vi "Text control 2 v7.3.vi"() -> ()   [LabVIEW 2019]
panel:
  in  "Tab Control":enum32{"Main", "Other parameters"}(tab)
  out "Vdg vs time (Bias Stress)":cluster{"Y data in":dbl[], "X data in":dbl[]}[](graph)
  out "Vp vs Vg (FPP)":cluster{"Y data in":dbl[], "X data in":dbl[]}[](graph)
  out "Vp2":dbl format="%.2e"
  out "Vp1":dbl format="%.2e"
  out "Vp vs time (FPP Bias Stress)":cluster{"Y data in":dbl[], "X data in":dbl[]}[](graph)
  in  "Plot sample extrema vs time":bool
  out "Line running":i32
  out "Total lines":i32
  out "Path":path=path "C:/users/rlp38/09Apr2009LTtesting/test2.txt"
  out "I vs Vg":cluster{"Y data in":dbl[], "X data in":dbl[]}[](graph)
  out "Is max":dbl format="%.2e"
  out "Id max":dbl format="%.2e"
  out "Ig max":dbl format="%.2e"
  out "Imax vs time":cluster{"Y data in":dbl[], "X data in":dbl[]}[](graph)
  out "Imin vs time":cluster{"Y data in":dbl[], "X data in":dbl[]}[](graph)
  out "I vs Vd":cluster{"Y data in":dbl[], "X data in":dbl[]}[](graph)
  in  "Script":string="#pulsedstressV d 0.03 20 0 0.5 0.0827 5\n#\n#itime m\n#gaterangemode a\n#drainrangemode a\n#pulsed on 0.05 0 0.02\n#transfer d -10 40 1 5 40 35\n#transfer d -10 40 1 5 40 35\n#transfer d -10 40 1 5 40 35\n#output d 0 40 20 0 40 1\n#\n#\n#sample 1 0.008 221 6 0.003\n#samplei 400e-6 200 6 0.002 0.1\n#vsu2pulse -10 4\n#\n#stressV 0.016 0.03 2e-4 0.1e-3 11\n#stressI 220e-7 0.08 15\n#transfer s -1 1 0.5 -0.005 0.005 0.005\n#output s 0 0 0 -0.008 0.008 0.002"
  out "Command running:":string
  out "Serial port data":string
  out "Elapsed Time":dbl caption="Elapsed Time (s)"
  in  "Time Units":u16(ring)=1 items=["Seconds", "Minutes", "Hours"]
  in  "Time Offset":dbl caption="Set Start Time (s)"
  in  "Reset":bool
  in  "Auto Reset":bool
  in  "integration time":u32(slide) max=2 step=1 scale=0.0..2.0
  out "Is on":dbl format="%.2e"
  out "Id on":dbl format="%.2e"
  out "Ig on":dbl format="%.2e"
  out "Ion vs time":cluster{"Y data in":dbl[], "X data in":dbl[]}[](graph)
  out "Ioff vs time":cluster{"Y data in":dbl[], "X data in":dbl[]}[](graph)
  out "Ig min":dbl format="%.2e"
  out "Id min":dbl format="%.2e"
  out "Is min":dbl format="%.2e"
  out "Is off":dbl format="%.2e"
  out "Id off":dbl format="%.2e"
  out "Ig off":dbl format="%.2e"
  in  "Integration time (long)":dbl=0.32 min=0.04 max=2.0 step=0.02 format="%.2f"
  in  "Integration time (short)":dbl=0.0019 min=8e-05 max=0.0019 step=8e-05 format="%^.0e"
  in  "Drain: Compliance":dbl=0.001 format="%.8f"
  in  "Gate: Compliance":dbl=0.001 format="%.8f"
  in  "Interrupt scan":bool
  in  "Interrupt program":bool
  in  "Plot output curve extrema vs time":bool
  in  "Plot transfer curve extrema vs time":bool
  out "I vs time (Bias Stress)":cluster{"Y data in":dbl[], "X data in":dbl[]}[](graph)
  in  "Sample I - Probe 4 (Disabled)":u32(ring)=3 items=["SMU1  ", "SMU2  ", "SMU3  ", "SMU4  ", "SMU5  ", "SMU6  ", "VSU1  ", "VSU2  "]
  in  "Sample I - Source/Common":u32(ring) items=["SMU1  ", "SMU2  ", "SMU3  ", "SMU4  ", "SMU5  ", "SMU6  ", "VSU1  ", "VSU2  "]
  in  "Sample I - Probe 3 (Disabled)":u32(ring)=2 items=["SMU1  ", "SMU2  ", "SMU3  ", "SMU4  ", "SMU5  ", "SMU6  ", "VSU1  ", "VSU2  "]
  in  "Sample I - Drain/Gate":u32(ring)=1 items=["SMU1  ", "SMU2  ", "SMU3  ", "SMU4  ", "SMU5  ", "SMU6  ", "VSU1  ", "VSU2  "]
  in  "Sample - Probe 4":u32(ring)=3 items=["SMU1  ", "SMU2  ", "SMU3  ", "SMU4  ", "SMU5  ", "SMU6  ", "VSU1  ", "VSU2  "]
  in  "Sample - Source/Common":u32(ring) items=["SMU1  ", "SMU2  ", "SMU3  ", "SMU4  ", "SMU5  ", "SMU6  ", "VSU1  ", "VSU2  "]
  in  "Sample - Gate":u32(ring)=2 items=["SMU1  ", "SMU2  ", "SMU3  ", "SMU4  ", "SMU5  ", "SMU6  ", "VSU1  ", "VSU2  "]
  in  "Sample - Drain":u32(ring)=1 items=["SMU1  ", "SMU2  ", "SMU3  ", "SMU4  ", "SMU5  ", "SMU6  ", "VSU1  ", "VSU2  "]
  in  "Gate Range\nmode":u16(ring) items=["Auto", "Limited", "Fixed"]
  in  "Gate Range":u8(slide)=3 max=11 scale=0.0..11.0
  in  "Source/Drain\nRange mode":u16(ring) items=["Auto", "Limited", "Fixed"]
  in  "Source/Drain Range":u8(slide)=3 max=11 scale=0.0..11.0
  in  "Panel Controls":T1={"Emergency Stop"=refnum, "TransGraph Max"=1e-05, "Text/Graph (text=false)"=TRUE} {"TransGraph Max" format="%.2e"}
  in  "Panel Controls 2":T2={"Emergency Stop"=refnum, "TransGraph Max"=1e-05, "Text/Graph (text=false)"=TRUE, "TransGraph Min"=1e-11} {"TransGraph Min" format="%.2e"; "TransGraph Max" format="%.2e"}
  out "error out":errorcluster
  in  "Delay before read (ms)":u32=1000
  in  "byte count":u32=64
  in  "Serial End Mode for Reads":u16(ring)=2 items=["None", "LastBit", "TermChar"]
  in  "Timeout (ms)":u32=10000
  in  "Enable Termination\nChar (T)":bool=TRUE
  in  "Termination char\n(0xA = '\\n' = LF)\n(0xD = '\\r' = CR)":u8=13 format="%.0x"
  in  "flow control":u16(ring) items=["None"=0, "XON/XOFF"=1, "RTS/CTS"=2, "DTR/DSR"=4]
  in  "stop bits":u16(ring)=10 items=["1.0"=10, "1.5"=15, "2.0"=20]
  in  "parity":u16(ring) items=["None", "Odd", "Even", "Mark", "Space"]
  in  "data bits":u16=8 min=5 max=8 step=1
  in  "VISA resource name":refnum<visa-resource-name>="COM6"
  in  "baud rate":u32=9600
  out "Timings Indicator":T3
  in  "Timings (overwritten by the Front Panel)":T4={"integration time"=0, "Short/Long integration time"=0.00064, "hold time (sec)"=0.0, "delay time (sec)"=0.0, "Step Time (0 disables)"=0.0, "sweep method"=0, "Pulse period"=0.005, "Base voltage"=0.0, "Pulse width"=0.0005} {"Pulse width" min=0.0005 max=0.1 step=0.0001 format="%.4f"; "Base voltage" format="%^.4e"; "Pulse period" min=0.005 max=1.0 step=0.0001 format="%.4f"; "sweep method" items=["Continuous", "Pulsed"]; "Step Time (0 disables)" format="%.2f"; "delay time (sec)" format="%.4f"; "hold time (sec)" format="%.4f"; "Short/Long integration time" format="%^.0e"; "integration time" scale=0.0..2.0}
  in  "Probe 4":cluster{"on/off":bool, "Voltage":dbl} {"Voltage" min=-100.0 max=100.0 format="%.2f"}
  in  "Full Reset":bool
  in  "Standby":T5
  out "Probe 4 Indicator":cluster{"on/off":bool, "Voltage":dbl} {"Voltage" min=-100.0 max=100.0 format="%.2f"}
  in  "Transfer/Output - Drain":u32(ring)=1 items=["SMU1  ", "SMU2  ", "SMU3  ", "SMU4  ", "SMU5  ", "SMU6  ", "VSU1  ", "VSU2  "]
  in  "Transfer/Output - Gate":u32(ring)=2 items=["SMU1  ", "SMU2  ", "SMU3  ", "SMU4  ", "SMU5  ", "SMU6  ", "VSU1  ", "VSU2  "]
  in  "Transfer/Output - Source/Common":u32(ring) items=["SMU1  ", "SMU2  ", "SMU3  ", "SMU4  ", "SMU5  ", "SMU6  ", "VSU1  ", "VSU2  "]
  in  "Transfer/Output - Probe 4":u32(ring)=3 items=["SMU1  ", "SMU2  ", "SMU3  ", "SMU4  ", "SMU5  ", "SMU6  ", "VSU1  ", "VSU2  "]
  in  "Pulsed Stress V - Probe 4":u32(ring)=3 items=["SMU1  ", "SMU2  ", "SMU3  ", "SMU4  ", "SMU5  ", "SMU6  ", "VSU1  ", "VSU2  "]
  in  "Pulsed Stress V - Vextra":u32(ring)=6 items=["SMU1  ", "SMU2  ", "SMU3  ", "SMU4  ", "SMU5  ", "SMU6  ", "VSU1  ", "VSU2  "]
  in  "Pulsed Stress V - Drain":u32(ring)=1 items=["SMU1  ", "SMU2  ", "SMU3  ", "SMU4  ", "SMU5  ", "SMU6  ", "VSU1  ", "VSU2  "]
  in  "Pulsed Stress V - Source/Common":u32(ring) items=["SMU1  ", "SMU2  ", "SMU3  ", "SMU4  ", "SMU5  ", "SMU6  ", "VSU1  ", "VSU2  "]
  in  "Pulsed Stress V - Gate":u32(ring)=2 items=["SMU1  ", "SMU2  ", "SMU3  ", "SMU4  ", "SMU5  ", "SMU6  ", "VSU1  ", "VSU2  "]
  in  "FPP - Drain":u32(ring)=1 items=["SMU1  ", "SMU2  ", "SMU3  ", "SMU4  ", "SMU5  ", "SMU6  ", "VSU1  ", "VSU2  "]
  in  "FPP - Gate":u32(ring)=2 items=["SMU1  ", "SMU2  ", "SMU3  ", "SMU4  ", "SMU5  ", "SMU6  ", "VSU1  ", "VSU2  "]
  in  "FPP - Probe 1":u32(ring) items=["SMU1  ", "SMU2  ", "SMU3  ", "SMU4  ", "SMU5  ", "SMU6  ", "VSU1  ", "VSU2  "]
  in  "FPP - Probe 2":u32(ring)=3 items=["SMU1  ", "SMU2  ", "SMU3  ", "SMU4  ", "SMU5  ", "SMU6  ", "VSU1  ", "VSU2  "]
  in  "FPP - Source":u32(ring)=6 items=["SMU1  ", "SMU2  ", "SMU3  ", "SMU4  ", "SMU5  ", "SMU6  ", "VSU1  ", "VSU2  "]
  in  "Stress V - Drain":u32(ring)=1 items=["SMU1  ", "SMU2  ", "SMU3  ", "SMU4  ", "SMU5  ", "SMU6  ", "VSU1  ", "VSU2  "]
  in  "Stress V - Gate":u32(ring)=2 items=["SMU1  ", "SMU2  ", "SMU3  ", "SMU4  ", "SMU5  ", "SMU6  ", "VSU1  ", "VSU2  "]
  in  "Stress V - Source/Common":u32(ring) items=["SMU1  ", "SMU2  ", "SMU3  ", "SMU4  ", "SMU5  ", "SMU6  ", "VSU1  ", "VSU2  "]
  in  "Stress I - Drain/Gate":u32(ring)=1 items=["SMU1  ", "SMU2  ", "SMU3  ", "SMU4  ", "SMU5  ", "SMU6  ", "VSU1  ", "VSU2  "]
  in  "Stress I - Source/Common":u32(ring) items=["SMU1  ", "SMU2  ", "SMU3  ", "SMU4  ", "SMU5  ", "SMU6  ", "VSU1  ", "VSU2  "]
  in  "VSU2 Stress - Source/Common":u32(ring) items=["SMU1  ", "SMU2  ", "SMU3  ", "SMU4  ", "SMU5  ", "SMU6  ", "VSU1  "]
  in  "VISA resource name in":refnum<visa-resource-name>="GPIB0::14::INSTR"
  in  "Gate":T6={"Gate Start"=0.0, "Gate Stop"=2.0, "Gate Step (linear only)"=1.0, "Gate Compliance"=0.0001, "Gate PComp"=0.0, "Range mode"=0, "Range"=6} {"Range" max=11 scale=0.0..11.0; "Range mode" items=["Auto", "Limited", "Fixed"]; "Gate PComp" format="%^.2e"; "Gate Compliance" format="%^.2e"; "Gate Step (linear only)" format="%^.4e"; "Gate Stop" format="%^.4e"; "Gate Start" format="%^.4e"}
  in  "Drain 2":T7={"Drain Start"=0.0, "Drain Stop"=2.0, "Drain Compliance"=0.0001, "Drain Step"=1.0, "Drain PComp"=0.0, "Range mode"=0, "Range"=6} {"Range" max=11 scale=0.0..11.0; "Range mode" items=["Auto", "Limited", "Fixed"]; "Drain PComp" format="%^.2e"; "Drain Step" format="%^.4e"; "Drain Compliance" format="%^.2e"; "Drain Stop" format="%^.4e"; "Drain Start" format="%^.4e"}
  # "Time"
  # "Syntax:\nitime [s|m|l] time(sec): [s|m|l] determines the integration time setting (small|medium|long) and time sets the value.\nNOTE: The value of the integration time has to be within the range allowed by its category (s|m|l), otherwise, the closest value will be used. (e.g. if the category is set to short but the time value is very long, the actual value used will be the maximum short integration time.\nIntegration times:\n    Short: Default: 640 us. Range: 8E-5 - 1.92E-3 seconds.\n    Medium: Fixed at 1 NPL cycle (0.02 seconds).\n    Long: Default: 16 NPL cycles (0.32 seconds). Range: 2-100 NPL cycles (0.04 seconds - 2 seconds).\ngaterangemode [a|l|f]\ndrainrangemode [a|l|f]\npulsed [on|off] PulsePeriod(sec) PulseBaseVoltage PulseONWidth(sec)\nstandby [on l off]\nwait NumMilliseconds\nwait-min NumMinutes\n# texthere = comment\nProbe4 [ON|OFF] Voltage\ntransfer [s|d] VgStart VgStop VgStep VdStart VdStop VdStep\noutput [s|d] VgStart VgStop VgStep VdStart VdStop VdStep\nsample Vg Vd NumSamples Time(s) SampleInterval(s)\nsamplei Idg NumSamples Time(s) SampleInterval(s) VDGcompliance\n100 samples is approximately 13 seconds with medium integration\n# if in doubt use SampleInterval(s) = 0.004\n    NOTE: When doing bias stress measurements, it is best to set the Time Units to \"Seconds\", as the \"sample\" command has been configured to give the output to seconds.\nstressV VG VD IGcompliance IDcompliance Duration(sec)\nstressI IDG VDGcompliance Duration(sec)\nvsu2pulse Bias Duration(s)\npulsedstressV [s|d] VEstop VgON VgOFF Period(s) PulseONwidth(s) Vd\nsample-fpp Vg Vd NumSamples Time\nresample-fpp Vg Vd\ntransfer-fpp [s|d] VgStart VgStop VgStep VdStart VdStop VdStep\noutput-fpp [s|d] VgStart VgStop VgStep VdStart VdStop VdStep\nserial SerialPortCommand"
  # "1\n2\n3\n4\n5\n6\n7\n8\n9\n10\n11\n12\n13\n14\n15\n16\n17\n18\n19\n20"
  # "SMUs"
  # "Serial port settings"
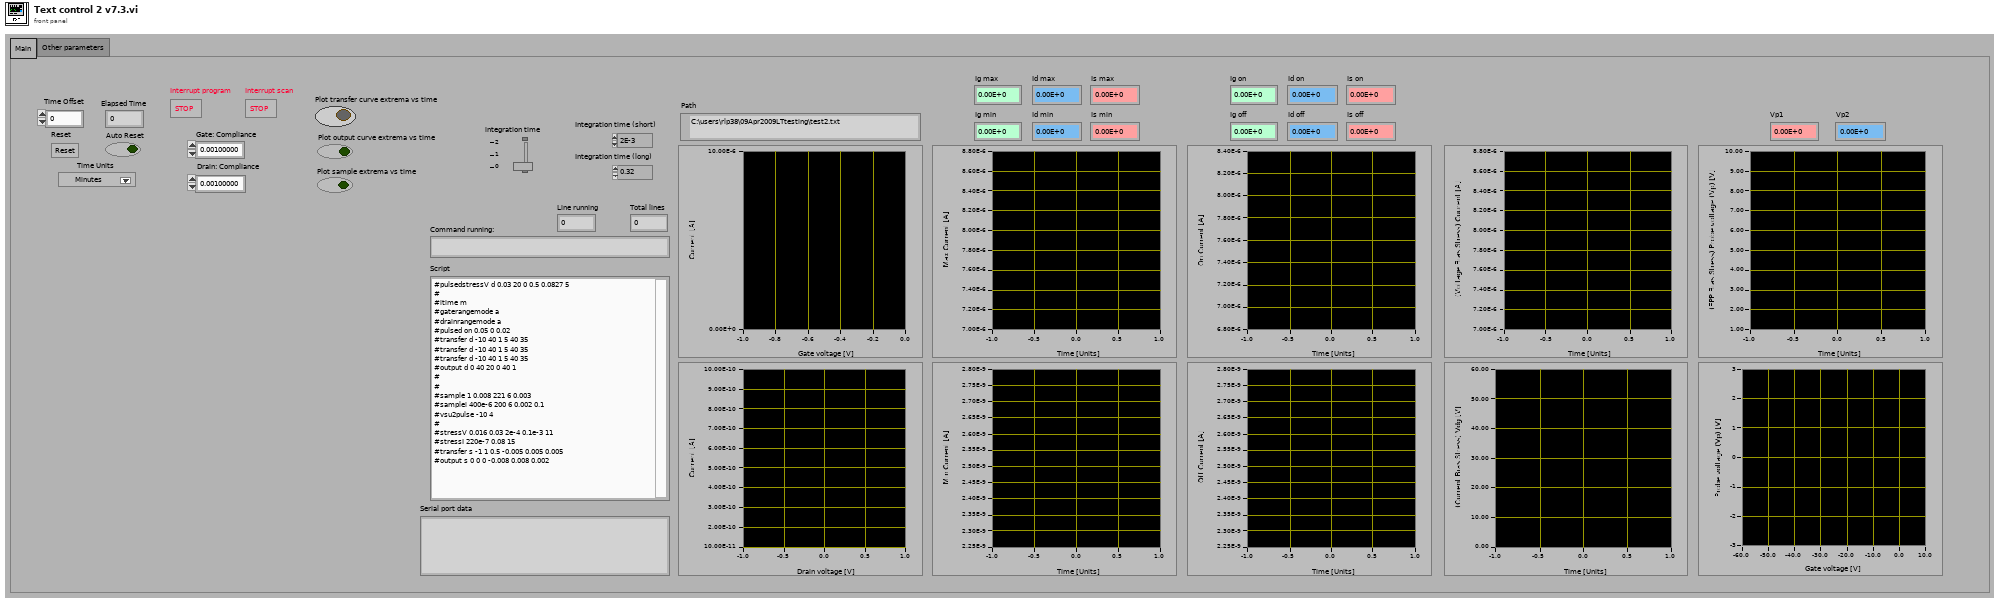
[diagram p1: front panel]
types:
  T1 = cluster{"Emergency Stop":refnum<vi>, "TransGraph Max":dbl, "Text/Graph (text=false)":bool}
  T2 = cluster{"Emergency Stop":refnum<vi>, "TransGraph Max":dbl, "Text/Graph (text=false)":bool, "TransGraph Min":dbl}
  T3 = cluster{"integration time (0:s, 1:m, 2:l)":u32, "Short/Long integration time":dbl, "hold time (sec)":dbl, "delay time (sec)":dbl, "Step Time (0 disables)":dbl, "sweep method":u16, "Pulse period":dbl, "Base voltage":dbl, "Pulse width":dbl}
  T4 = cluster{"integration time":u32, "Short/Long integration time":dbl, "hold time (sec)":dbl, "delay time (sec)":dbl, "Step Time (0 disables)":dbl, "sweep method":u16, "Pulse period":dbl, "Base voltage":dbl, "Pulse width":dbl}
  T5 = cluster{"Gate Standby":bool, "Drain Standby":bool}
  T6 = cluster{"Gate Start":dbl, "Gate Stop":dbl, "Gate Step (linear only)":dbl, "Gate Compliance":dbl, "Gate PComp":dbl, "Range mode":u16, "Range":u8}
  T7 = cluster{"Drain Start":dbl, "Drain Stop":dbl, "Drain Compliance":dbl, "Drain Step":dbl, "Drain PComp":dbl, "Range mode":u16, "Range":u8}
  T8 = enum16{"open", "replace", "create", "open or create", "replace or create", "replace or create with confirmation"}
  T9 = cluster{"V2 Start":dbl, "V2 Step":dbl, "Number of points":i32}
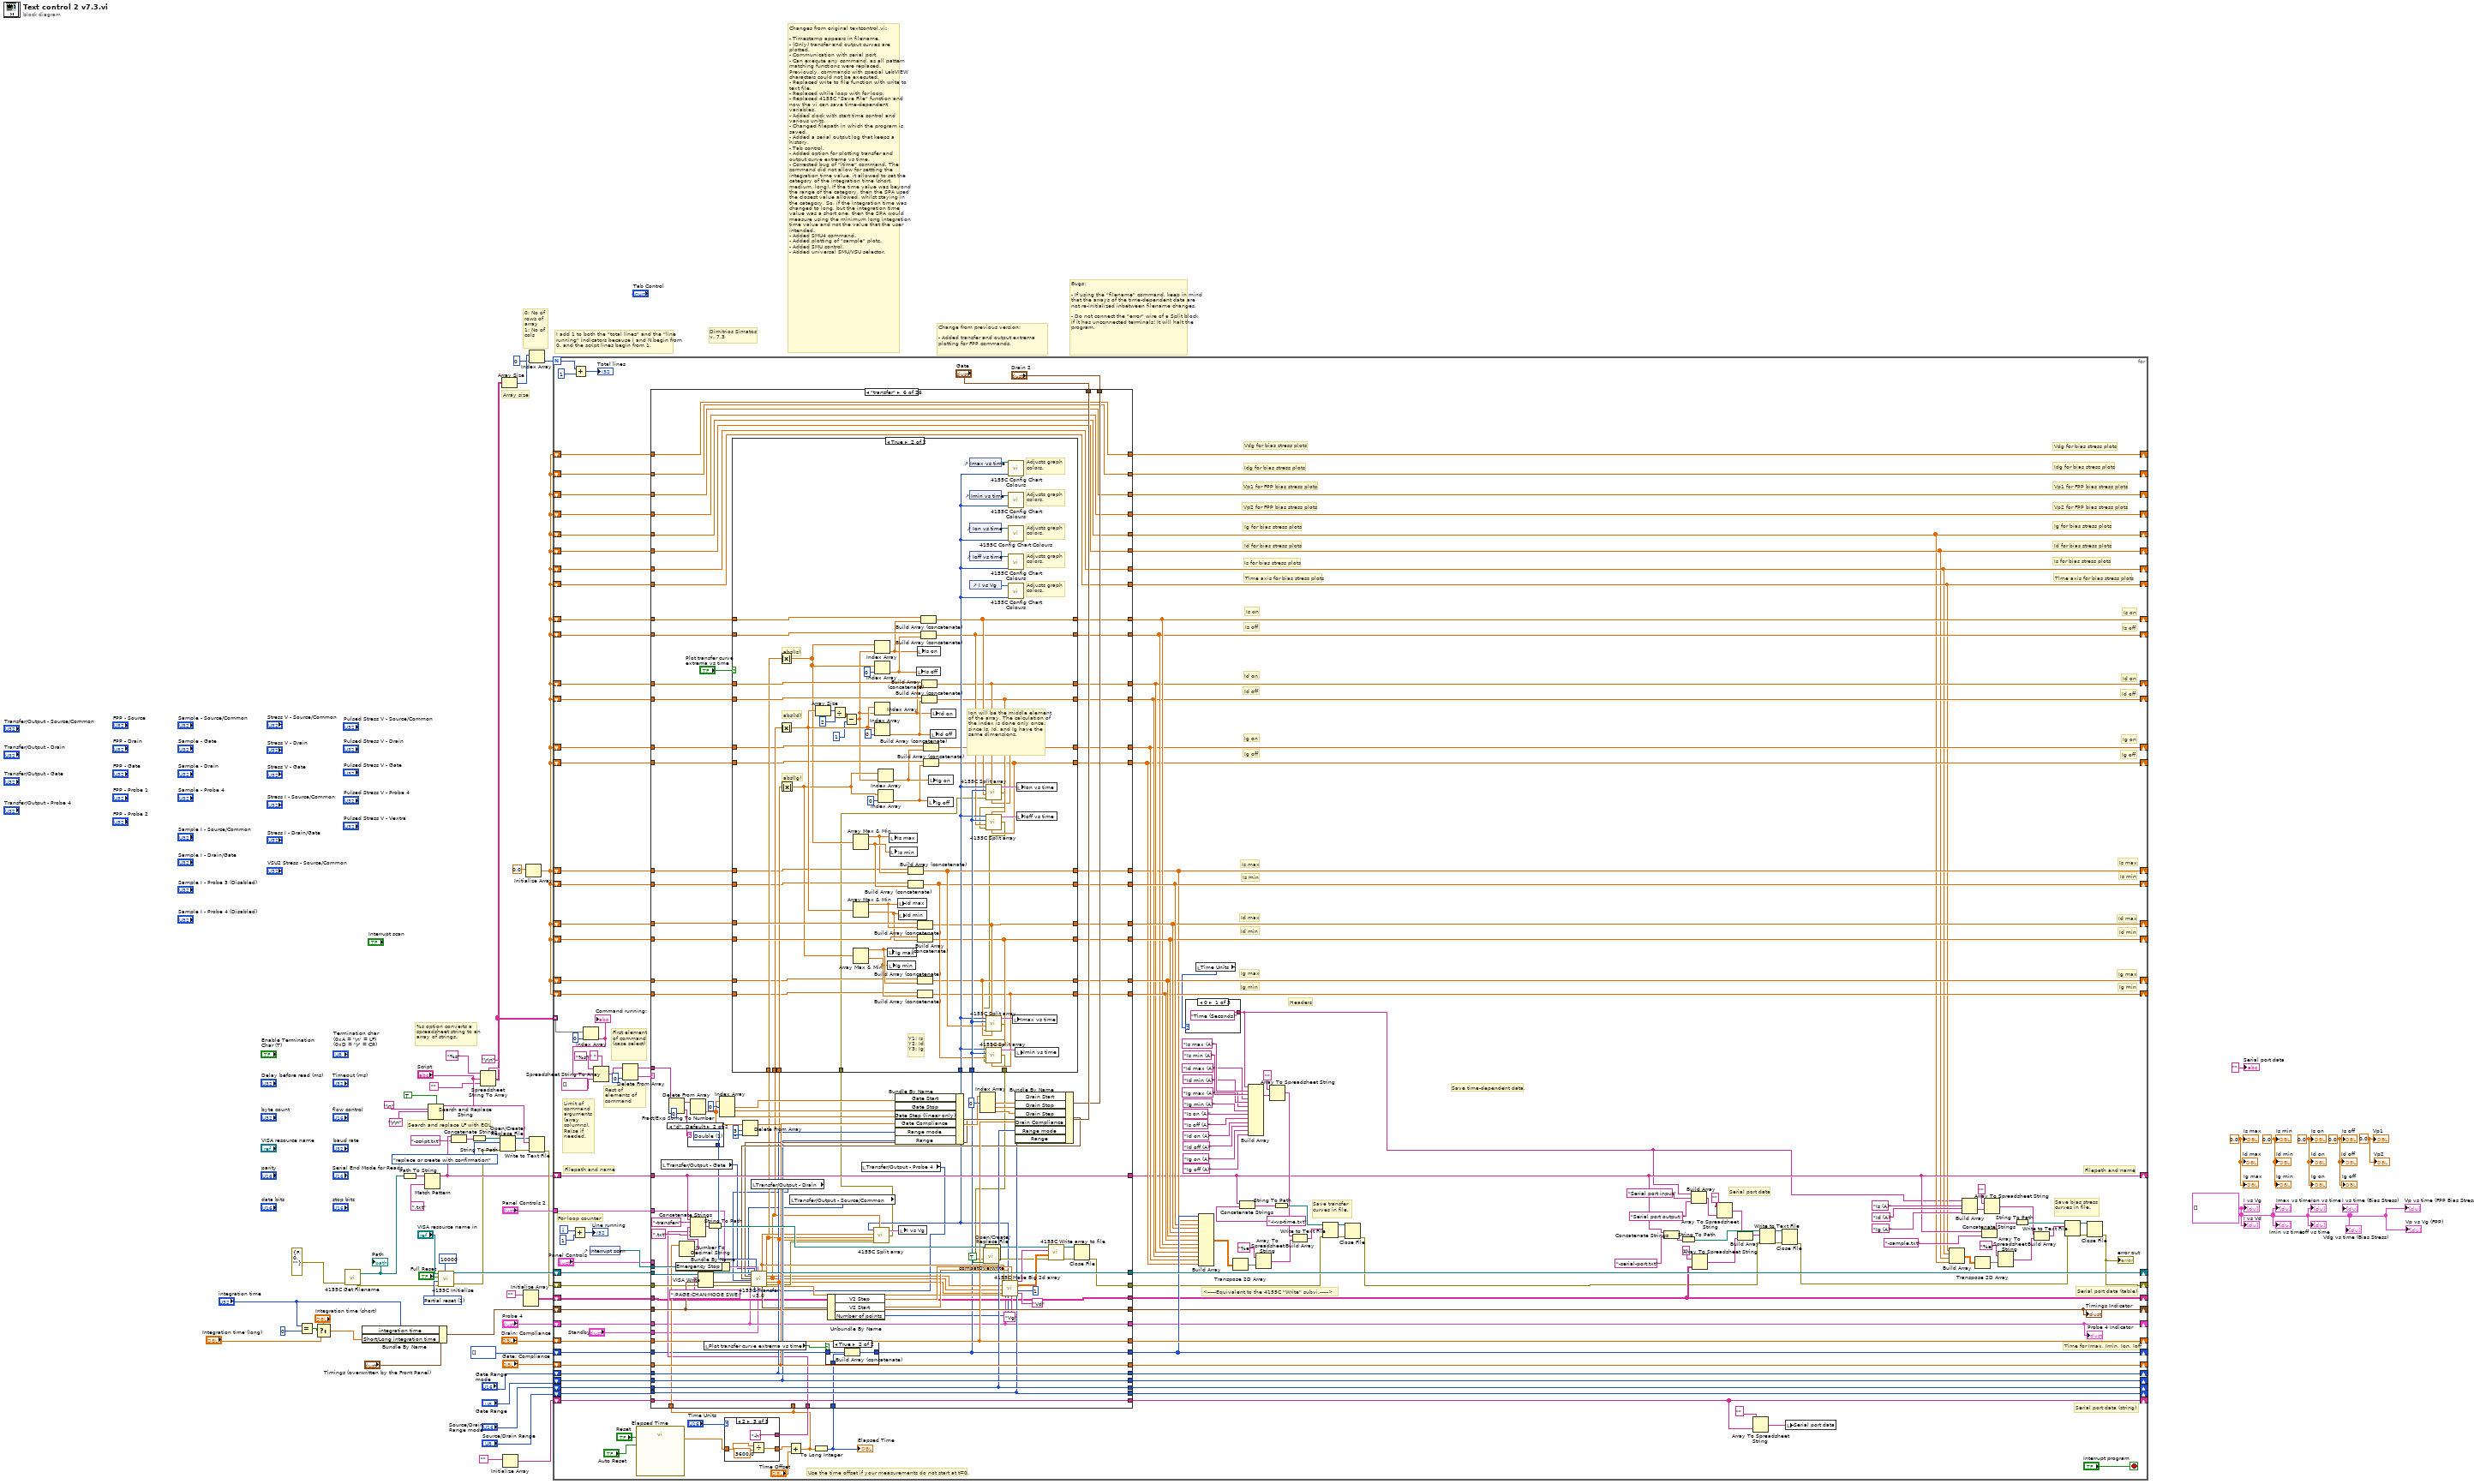
[diagram p0: block diagram]
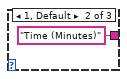
[diagram p2: hidden frame]
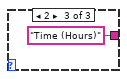
[diagram p3: hidden frame]
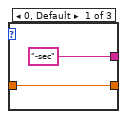
[diagram p4: hidden frame]
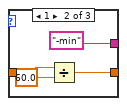
[diagram p5: hidden frame]
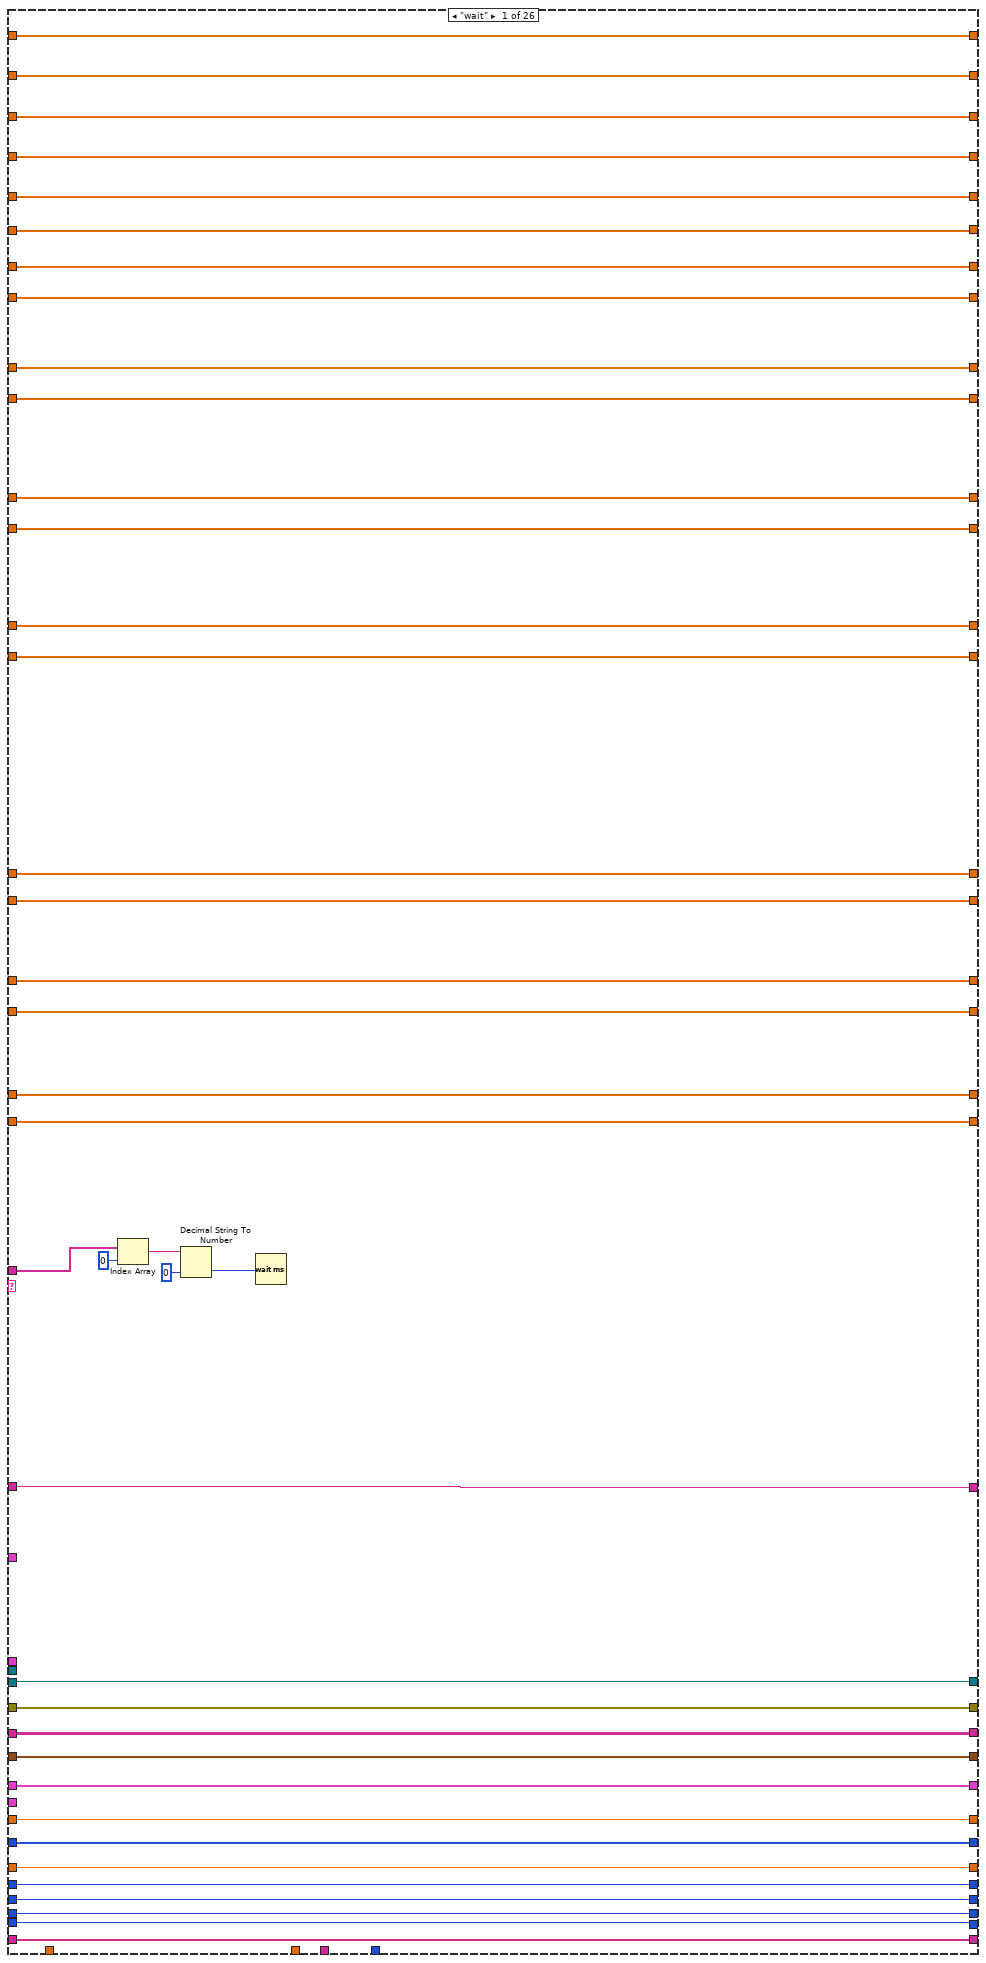
[diagram p6: hidden frame]
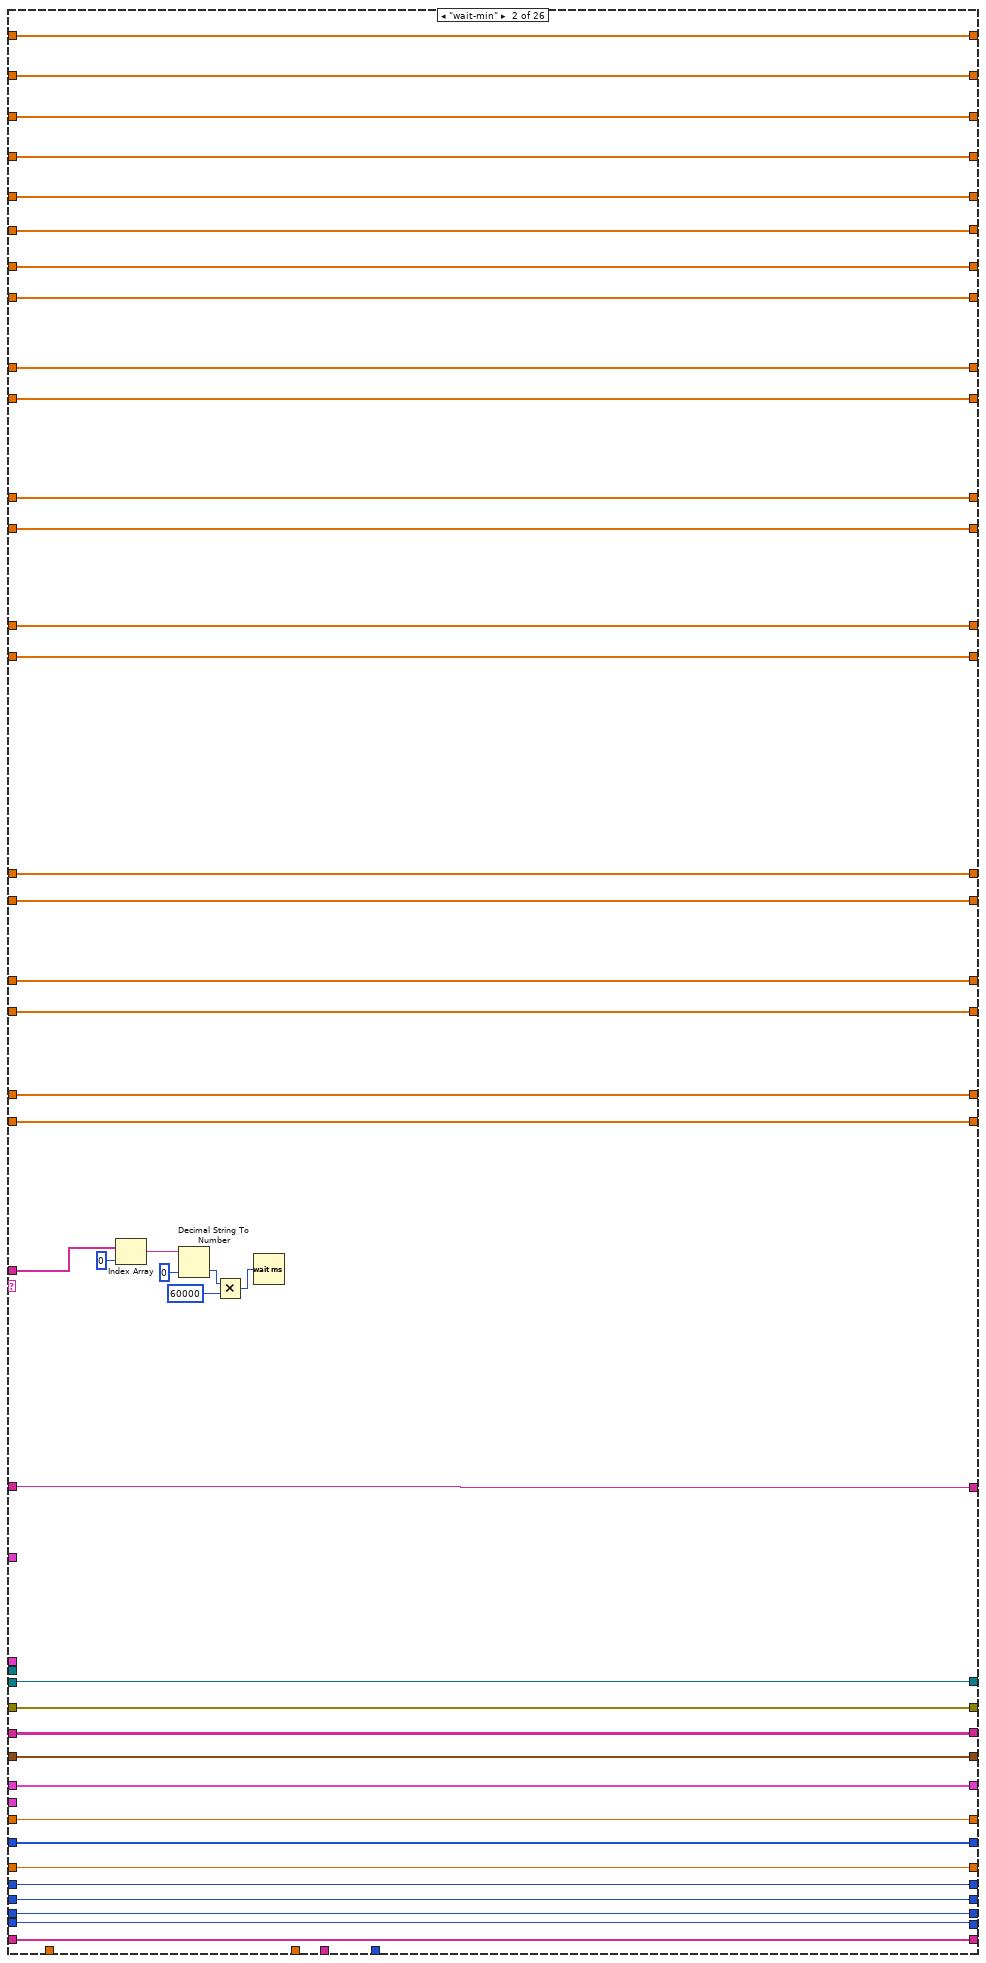
[diagram p7: hidden frame]
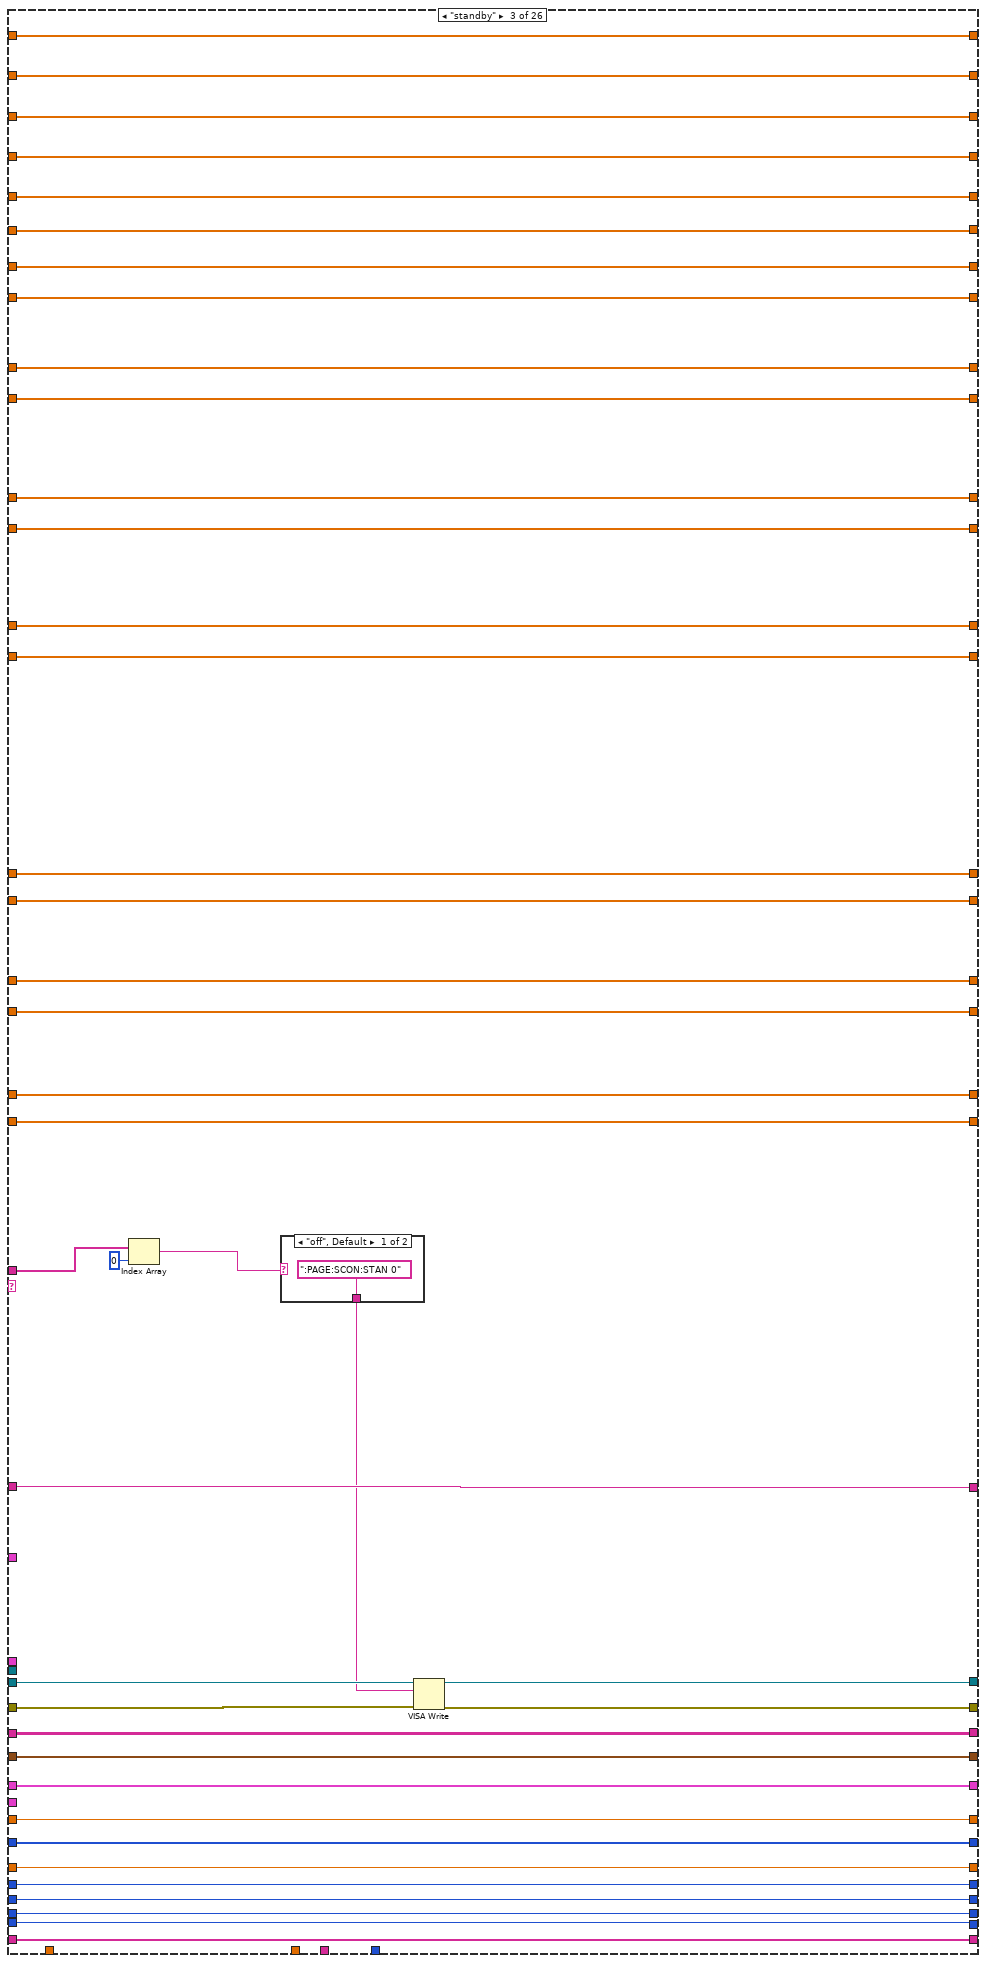
[diagram p8: hidden frame]
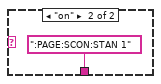
[diagram p9: hidden frame]
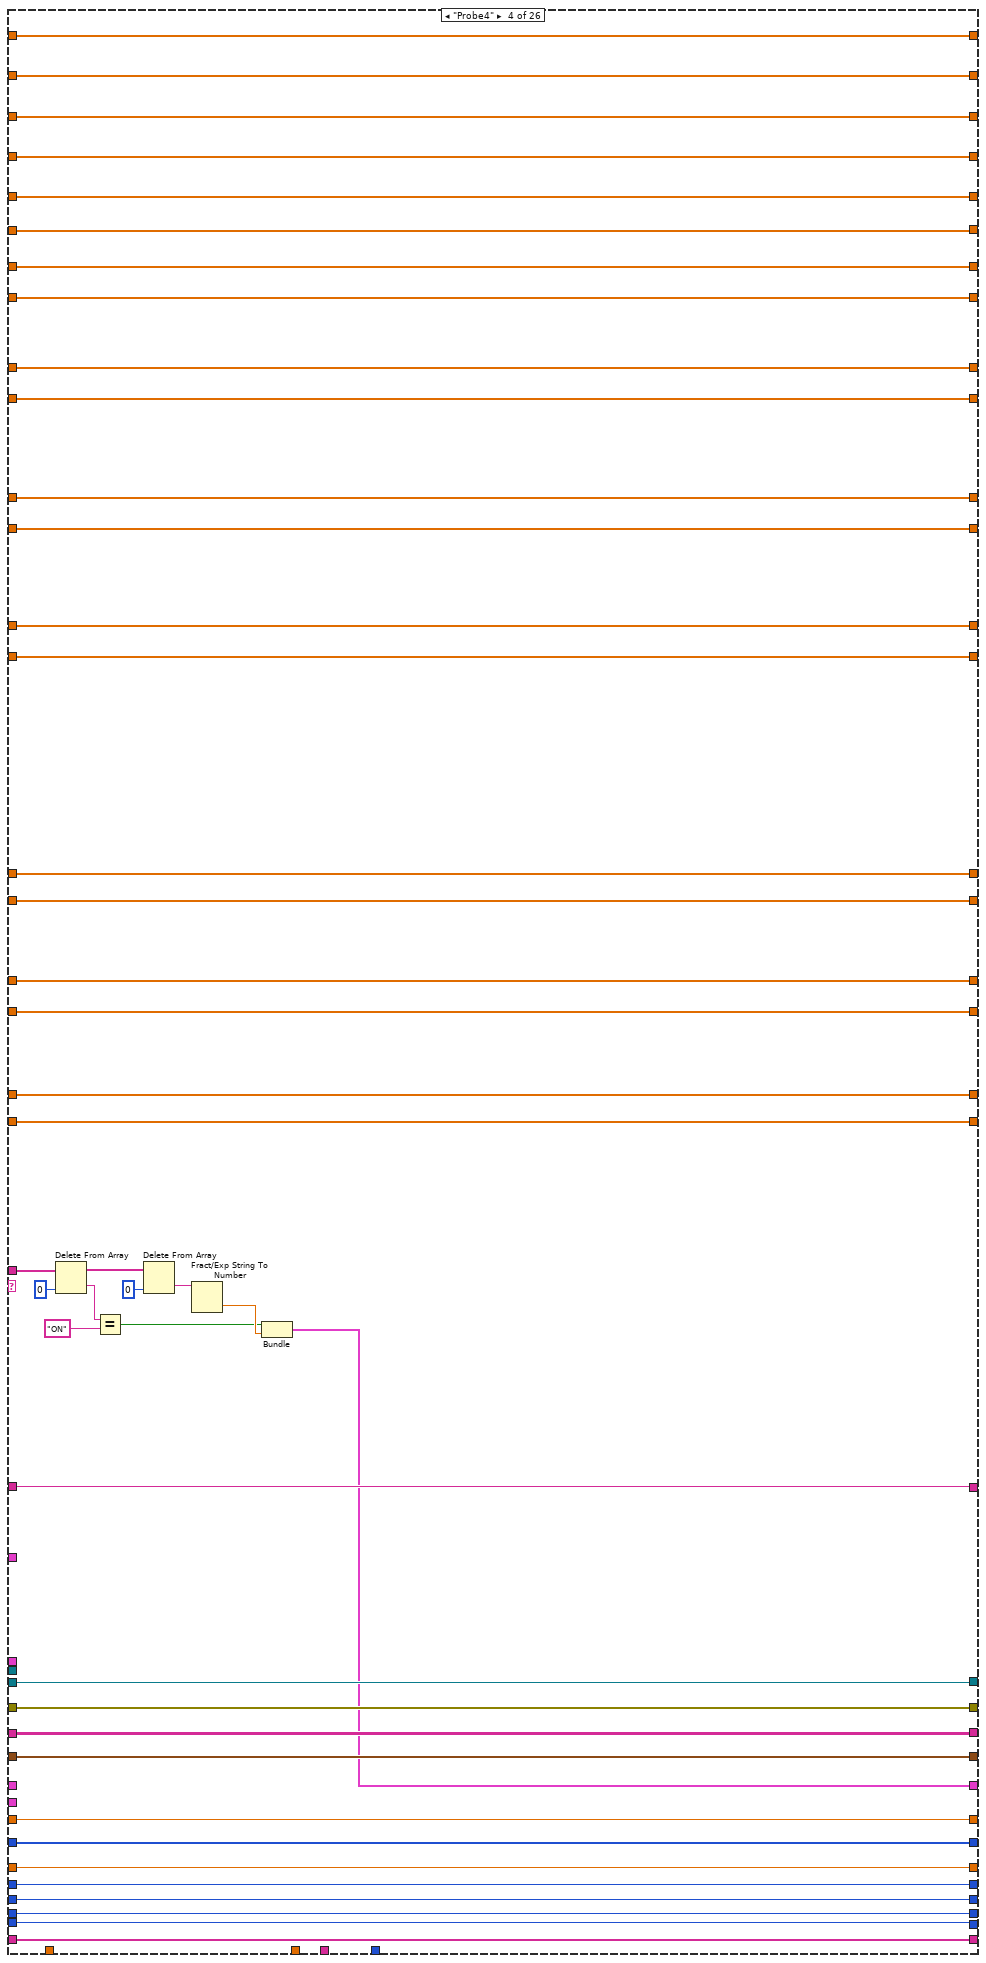
[diagram p10: hidden frame]
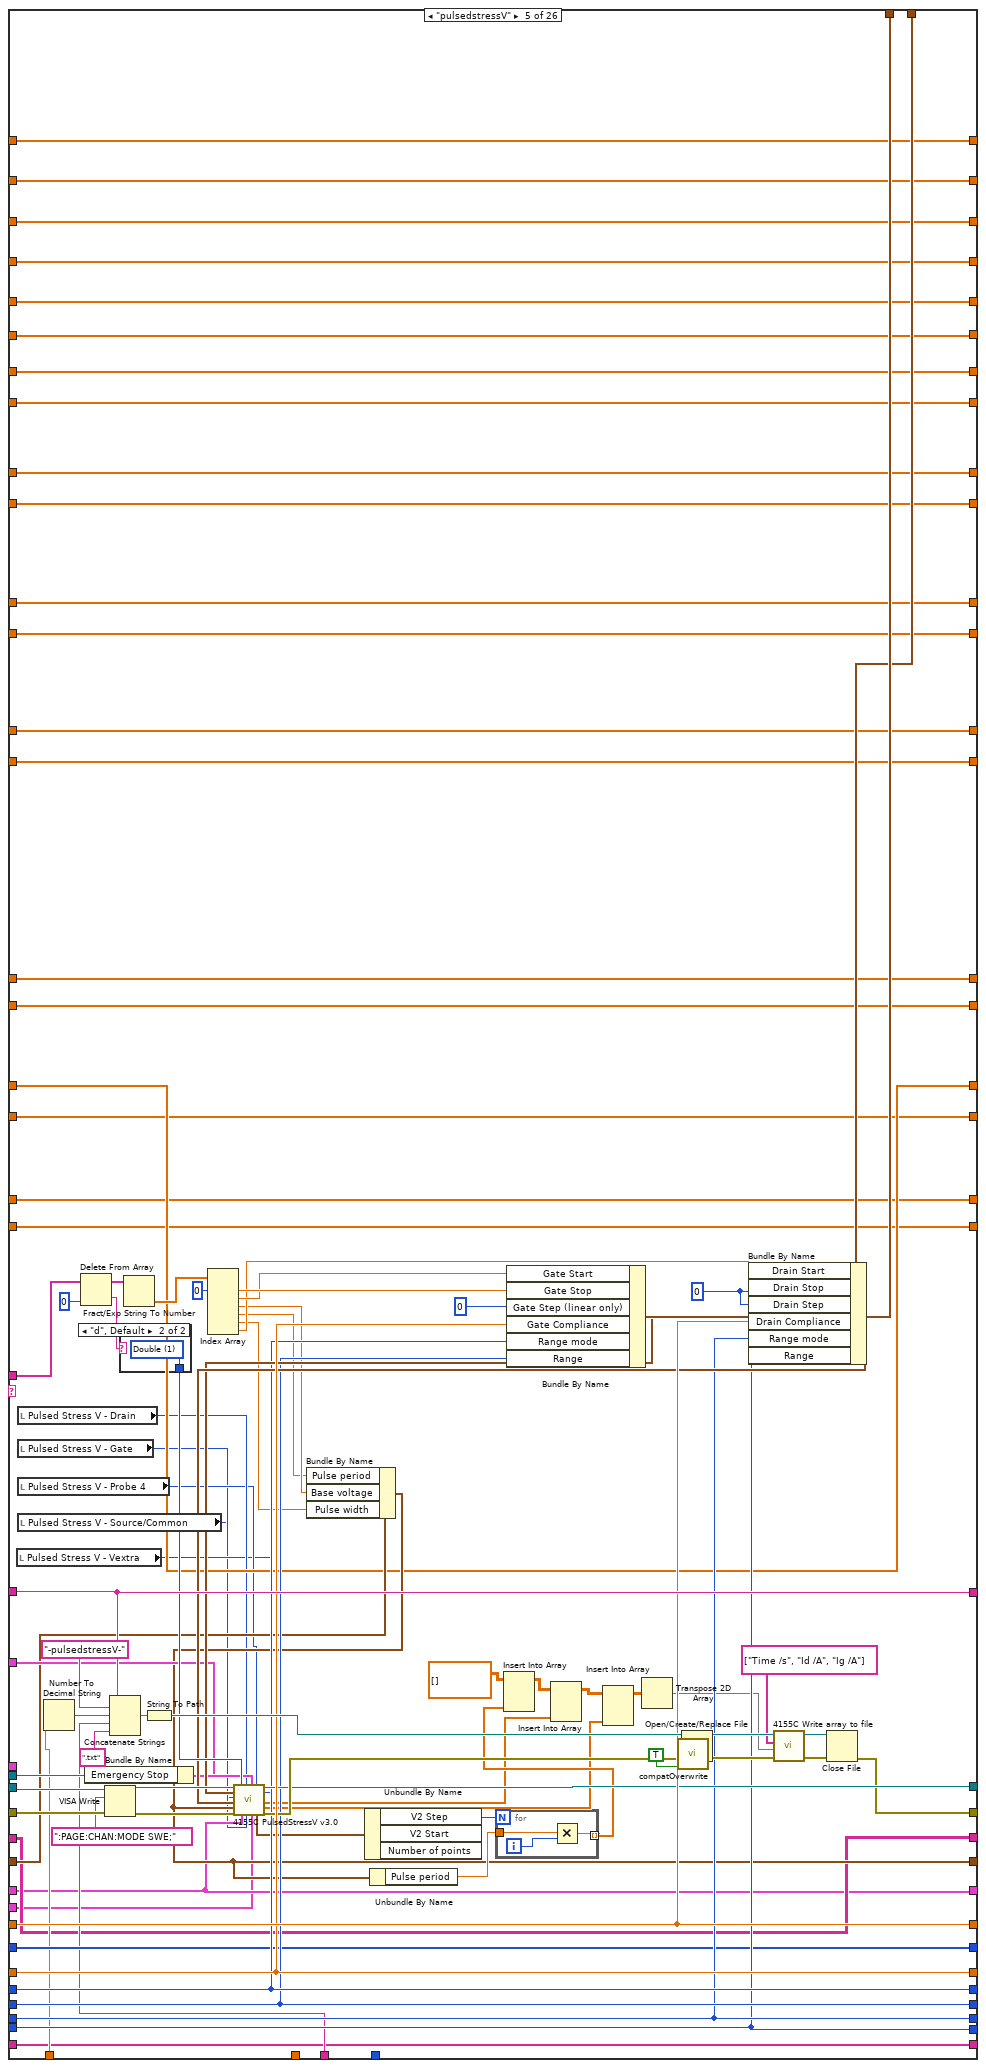
[diagram p11: hidden frame]
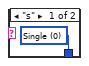
[diagram p12: hidden frame]
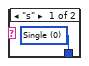
[diagram p15: hidden frame]
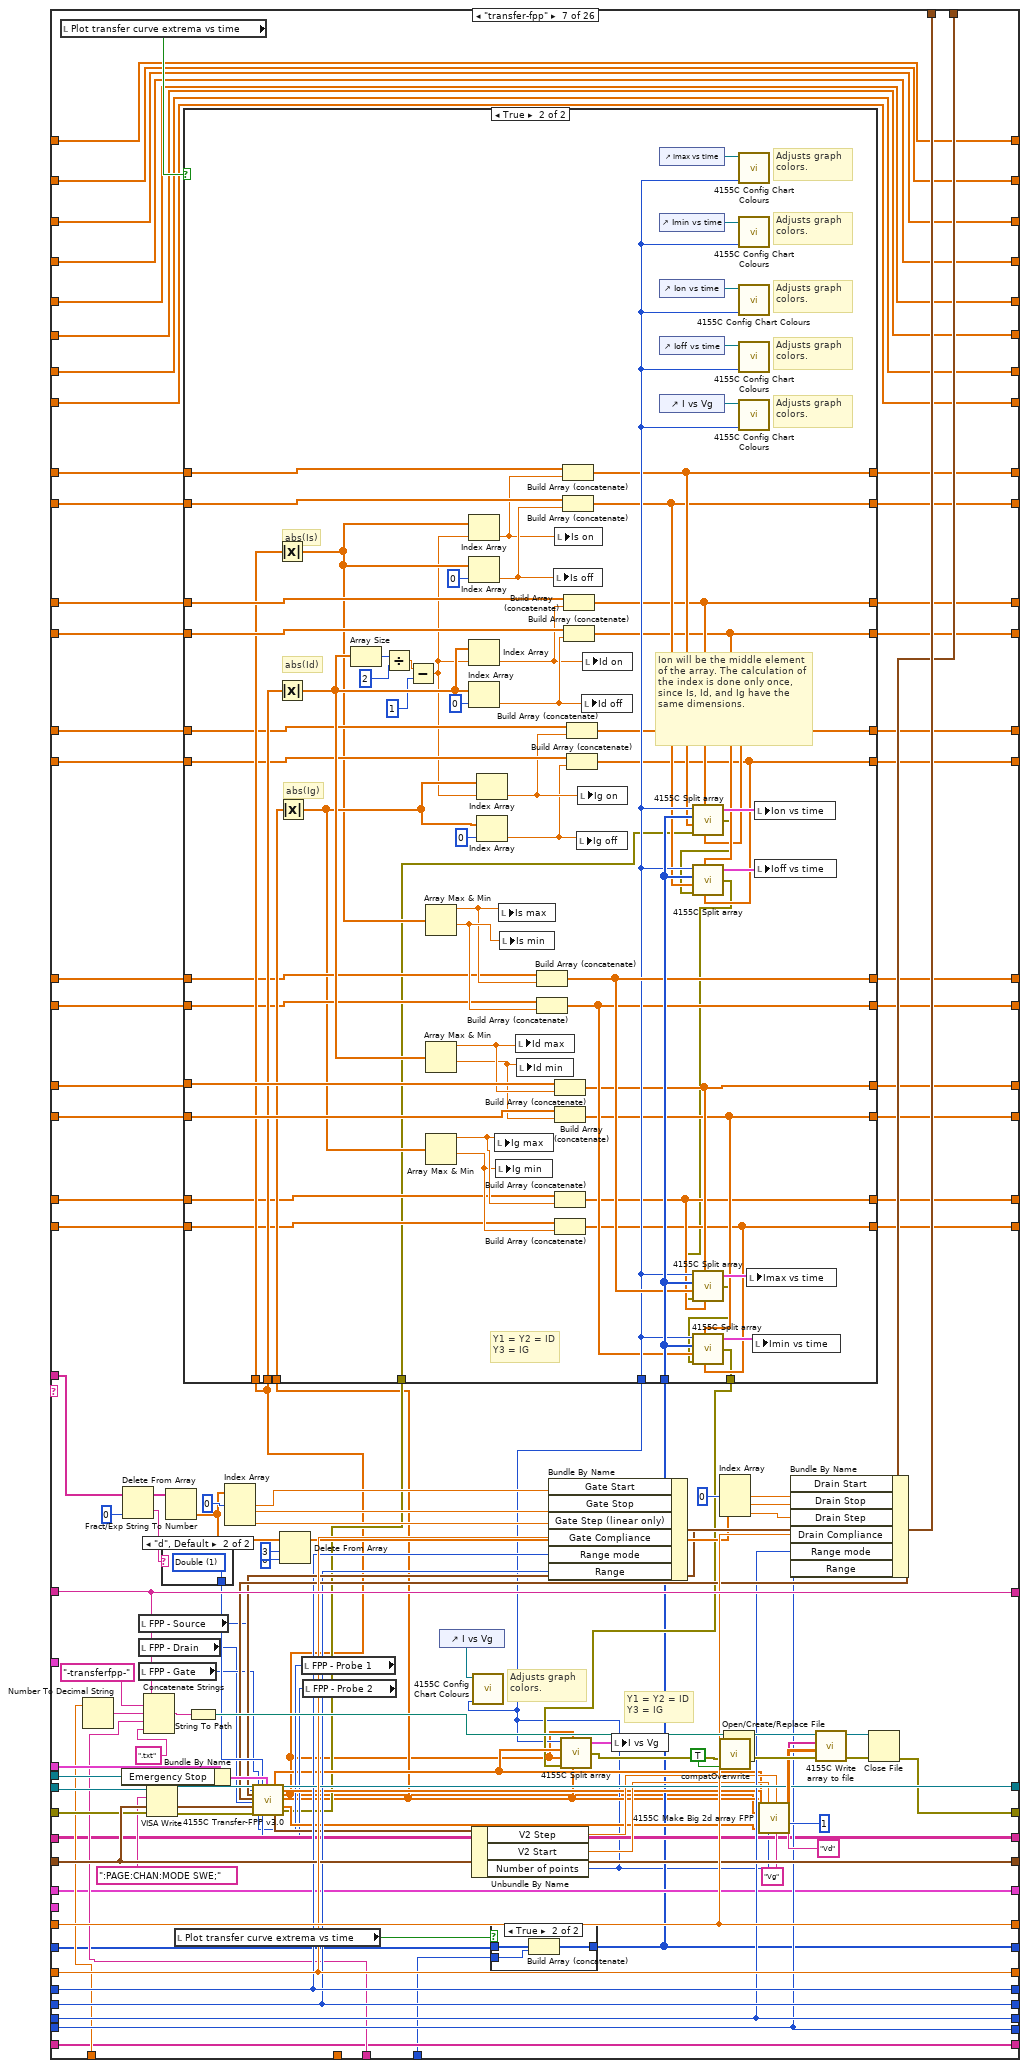
[diagram p16: hidden frame]
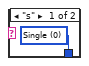
[diagram p19: hidden frame]
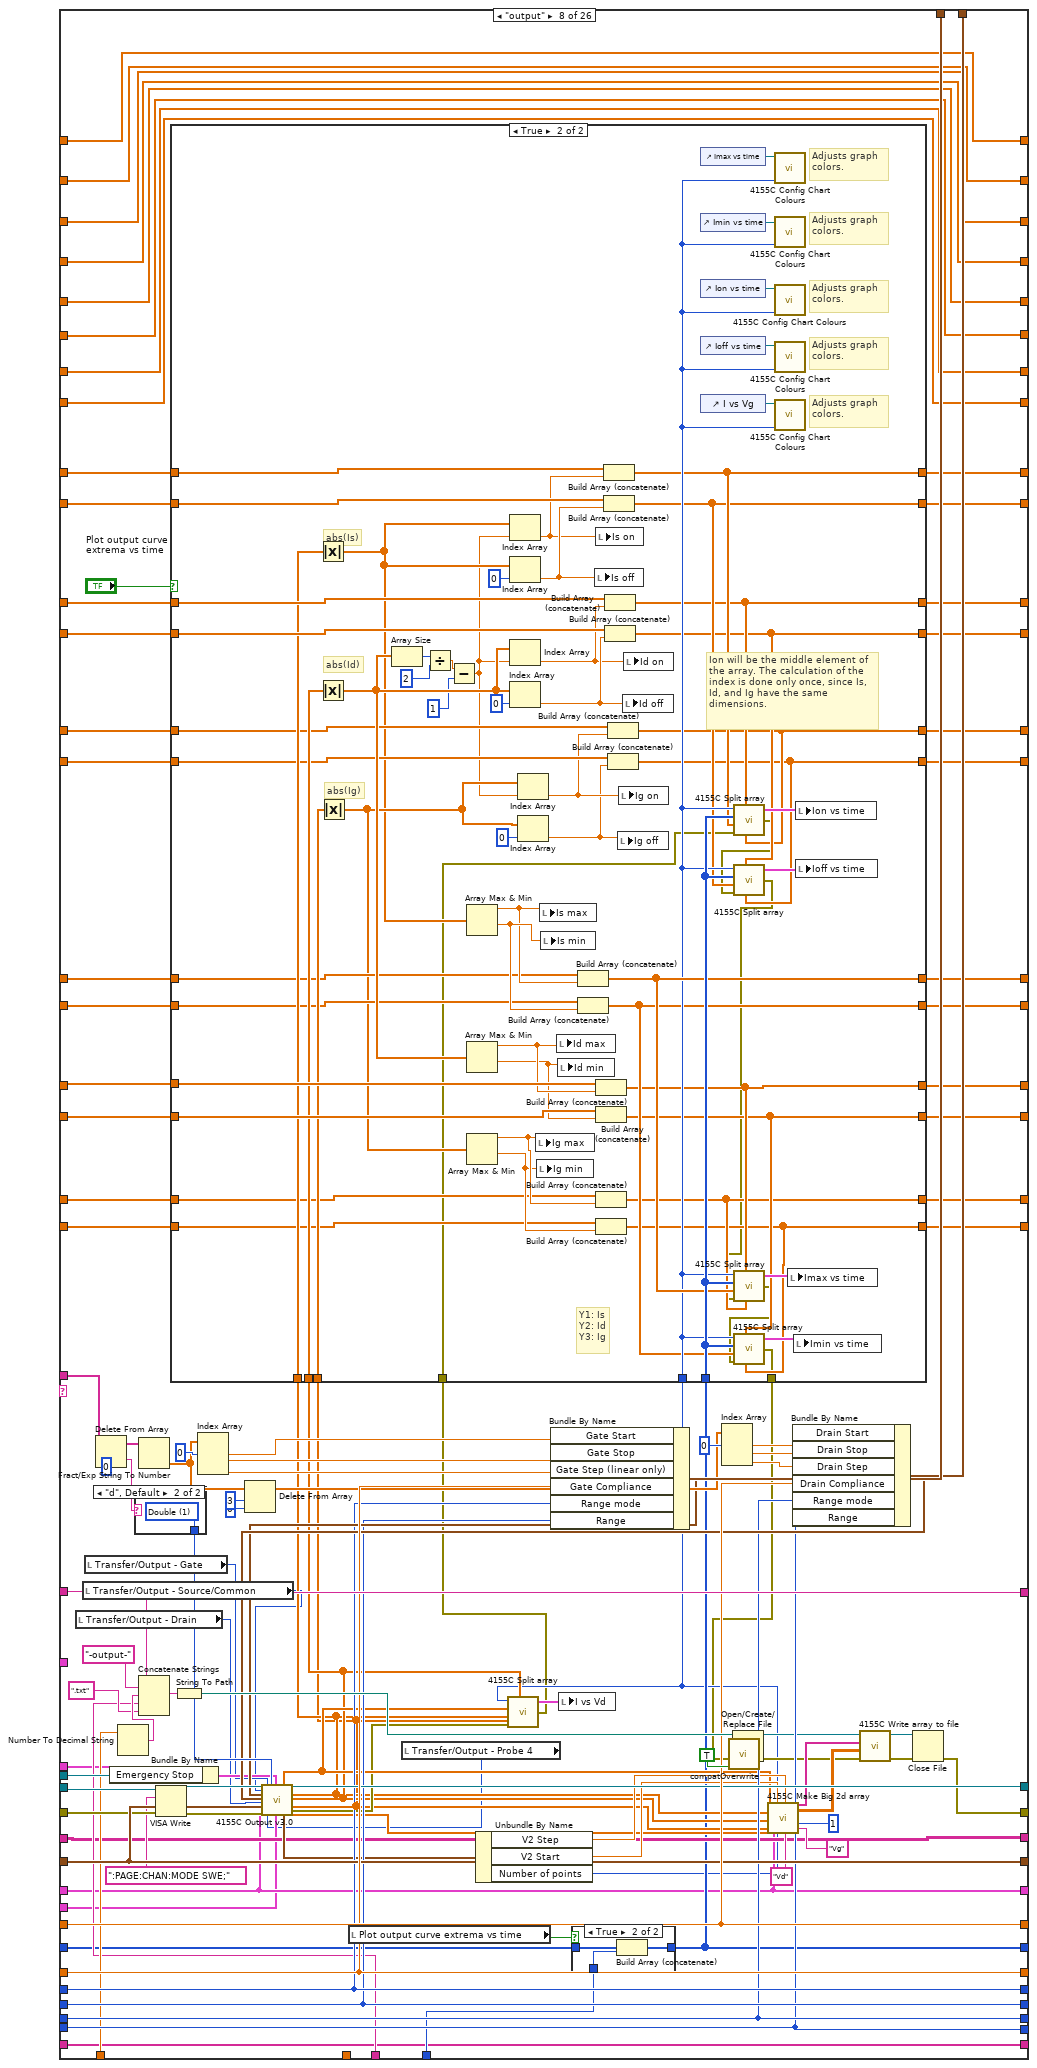
[diagram p20: hidden frame]
diagram:
  w3 = 0.0 ("Is off")
  w2 = cluster{"Y data in":dbl[], "X data in":dbl[]}[] [] ("I vs Vg")
  w10 = 0.0 ("Is off")
  w11 = 0.0 ("Is on")
  w12 = 0.0 ("Is min")
  w13 = 0.0 ("Is max")
  w56 = u16 1 items=["Reset All", "Partial reset"] ("Type of reset")
  # "Change from previous version:\n\n- Added transfer and output extrema plotting for FPP commands."
  # "I add 1 to both the \"total lines\" and the \"line running\" indicators because i and N begin from 0, and the script lines begin from 1."
  # "Bugs:\n\n- If using the \"filename\" command, keep in mind that the arrays of the time-dependent data are not re-initialized inbetween filename changes. \n\n- Do not connect the \"error\" wire of a Split block if it has unconnected terminals! It will halt the program."
  # "Array size"
  # "%s option converts a spreadsheet string to an array of strings."
  # "0: No of rows of array\n1: No of cols"
  # "Dimitrios Simatos\nv. 7.3"
  # "Changes from original textcontrol.vi:\n\n- Timestamp appears in filename.\n- (Only) transfer and output curves are plotted.\n- Communication with serial port.\n- Can execute any command, as all pattern matching functions were replaced. Previously, commands with special LabVIEW characters could not be executed.\n- Replaced write to file function with write to text file.\n- Replaced while loop with for loop.\n- Replaced 4155C \"Save File\" function and now the vi can save time-dependent variables.\n- Added clock with start time control and various units.\n- Changed filepath in which the program is saved.\n- Added a serial output log that keeps a history.\n- Tab control.\n- Added option for plotting transfer and output curve extrema vs time.\n- Corrected bug of \"itime\" command. The command did not allow for settting the integration time value, it allowed to set the category of the integration time (short, medium, long). If the time value was beyond the range of the category, then the SPA used the closest value allowed, whilst staying in the category. So, if the integration time was changed to long, but the integration time value was a short one, then the SPA would measure using the minimum long integration time value and not the value that the user intended.\n- Added SMU4 command.\n- Added plotting of \"sample\" plots.\n- Added SMU control.\n- Added universal SMU/VSU selector."
  # "Search and replace LF with EOL"
  n1 = Equal?(x="integration time", y=u32 0) -> (x = y?=w57:bool)
  n2 = Select(t="Integration time (short)", s=w57, f="Integration time (long)") -> (s? t:f=w18:dbl)
  n3 = call "4155C Get Filename.vi"("error in (no error)"=errorcluster {"status"=FALSE, "code"=0, "source"=""}) -> ("error out"=w51:errorcluster, "path"=w26:path)  [unwired: 2 in, 1 out]
  "Path" <- w26
  n4 = Bundle By Name(cluster="Timings (overwritten by the Front Panel)", "integration time"="integration time", "Short/Long integration time"=w18) -> (w49:T4)
  n5 = Path To String(path=w26) -> (string=w27:string)
  n6 = Match Pattern(string=w27, regular expression=".txt") -> (before substring=w16:string)  [unwired: 1 in, 3 out]
  n7 = Search and Replace String(replace all?=TRUE ("replace all? (F)"), input string="Script", search string="\n", replace string="\r\n") -> (result string=w39:string)  [unwired: 4 in, 3 out]
  n8 = call "4155C Initialise.vi"("VISA resource name in"="VISA resource name in", "Reset"="Full Reset", "Type of reset"=w56, "error in (no error)"=w51, "VISA Timeout Value"=u32 10000) -> ("VISA Resource Name out"=w50:refnum<visa-resource-name>, "error out"=w8:errorcluster)
  n9 = Concatenate Strings(w16, "-script.txt" ("string")) -> (w17:string)
  n10 = String To Path(string=w17) -> (path=w6:path)
  n11 = Spreadsheet String To Array(delimiter (Tab)="\r\n", format string="%s", spreadsheet string="Script", array type (2D Dbl)="") -> (array=w30:string[][])
  n12 = Open/Create/Replace File(file path (use dialog)=w6, error in=w8, operation (0:open)=T8."replace or create with confirmation") -> (refnum out=w5:refnum<file>, error out=w7:errorcluster)  [unwired: 3 in, 1 out]
  n13 = Array Size(array=w30) -> (size(s)=w34:i32[])
  n14 = Initialize Array("") -> (w21:string[])  [unwired: 1 in]
  n15 = Initialize Array("") -> (w19:string[][])  [unwired: 2 in]
  n16 = Initialize Array(0.0 ("element")) -> (w1:dbl[])  [unwired: 1 in]
  n17 = Index Array(array=w34, index=0) -> (element=w32:i32)
  n18 = Write to Text File(file (use dialog)=w5, text=w39, error in=w7) -> (error out=w24:errorcluster)  [unwired: 1 in, 2 out]
  n19 = for {
    N: w32 -> [w166]
    shift-left: "Source/Drain Range" -> [w206]
    shift-right: [w202] -> _
    shift-left: "Source/Drain\nRange mode" -> [w207]
    shift-right: [w203] -> _
    shift-left: "Gate Range" -> [w208]
    shift-right: [w204] -> _
    shift-left: "Gate Range\nmode" -> [w209]
    shift-right: [w205] -> _
    shift-left: "Gate: Compliance" -> [w217]
    shift-right: [w214] -> _
    shift-left: "Drain: Compliance" -> [w218]
    shift-right: [w215] -> _
    shift-left: w49 -> [w219]
    shift-right: [w71] -> _
    shift-left: w24 -> [w220]
    shift-right: [w72] -> _
    shift-left: w50 -> [w221]
    shift-right: [w216] -> _
    shift-left: w16 -> [w222]
    shift-right: [w79] -> _
    tunnel: "Panel Controls 2" -> [w200]
    shift-right: [w119] -> _
    shift-left: w1 -> [w199]
    shift-right: [w153] -> _
    shift-left: i32[] [] -> [w195]
    tunnel: w30 -> [w194] mode=indexing
    shift-right: [w118] -> _
    shift-left: w1 -> [w171]
    shift-right: [w148] -> _
    shift-left: w21 -> [w158]
    shift-right: [w149] -> _
    shift-left: w19 -> [w151]
    shift-right: [w112] -> _
    shift-left: w1 -> [w140]
    shift-right: [w113] -> _
    shift-left: w1 -> [w139]
    shift-right: [w117] -> _
    shift-left: w1 -> [w128]
    shift-right: [w116] -> _
    shift-left: w1 -> [w127]
    shift-right: [w110] -> _
    shift-left: w1 -> [w126]
    shift-right: [w120] -> _
    shift-left: w1 -> [w125]
    shift-right: [w111] -> _
    shift-left: w1 -> [w124]
    shift-right: [w109] -> _
    shift-left: w1 -> [w123]
    shift-right: [w115] -> _
    shift-left: w1 -> [w122]
    shift-right: [w114] -> _
    shift-left: w1 -> [w121]
    shift-right: [w70] -> _
    shift-left: "Probe 4" -> [w201]
    shift-right: [w75] -> _
    shift-left: w1 -> [w100]
    shift-right: [w76] -> _
    shift-left: w1 -> [w99]
    shift-right: [w77] -> _
    shift-left: w1 -> [w98]
    shift-right: [w78] -> _
    shift-left: w1 -> [w97]
    shift-right: [w67] -> _
    shift-left: w1 -> [w69]
    shift-right: [w66] -> _
    shift-left: w1 -> [w68]
    shift-right: [w63] -> _
    shift-left: w1 -> [w65]
    shift-right: [w62] -> _
    shift-left: w1 -> [w64]
    i -> [w161]
    stop <- "Interrupt program" stop-if-true
    # "Vdg for bias stress plots"
    # "Idg for bias stress plots"
    # "Vp2 for FPP bias stress plots"
    # "Vp1 for FPP bias stress plots"
    # "Ig for bias stress plots"
    # "Id for bias stress plots"
    # "Is for bias stress plots"
    # "Time axis for bias stress plots"
    # "Vdg for bias stress plots"
    # "Idg for bias stress plots"
    # "Vp2 for FPP bias stress plots"
    # "Vp1 for FPP bias stress plots"
    # "Ig for bias stress plots"
    # "Id for bias stress plots"
    # "Is for bias stress plots"
    # "Time axis for bias stress plots"
    # "Save bias stress curves in file."
    # "Is off"
    # "Is on"
    # "Ig off"
    # "Ig on"
    # "Is min"
    # "Is max"
    # "Ig min"
    # "Ig max"
    # "Id min"
    # "Id max"
    # "Id off"
    # "Id on"
    # "Is off"
    # "Is on"
    # "Ig off"
    # "Ig on"
    # "Is min"
    # "Is max"
    # "Ig min"
    # "Ig max"
    # "Id min"
    # "Id max"
    # "Id off"
    # "Id on"
    # "Filepath and name"
    # "Limit of command arguments (array columns). Raise if needed."
    # "Serial port data (string)"
    # "Serial port data (table)"
    # "Serial port data"
    # "For loop counter"
    # "<-----Equivalent to the 4155C \"Write\" subvi.----->"
    # "Headers"
    # "Save transfer curves in file."
    # "Filepath and name"
    # "Save time-dependent data."
    # "Use the time offset if your measurements do not start at t=0."
    # "Time for Imax, Imin, Ion, Ioff"
    # "Rest of elements of command"
    # "First element of command\n(case select)"
    n20 = Add(x=w161, y=1) -> (x+y=→"Line running":i32)
    n21 = Add(x=w166, y=1) -> (x+y=→"Total lines":i32)
    n22 = Index Array(array=w194, index=0 ("line index")) -> (element=w189:string)
    "Command running:" <- w189
    n23 = control-ref of="Interrupt scan"() -> (w213:refnum<vi>)
    n24 = Spreadsheet String To Array(delimiter (Tab)=" ", format string="%s", spreadsheet string=w189, array type (2D Dbl)=string[] []) -> (array=w187:string[])
    n25 = Delete From Array(array=w187, index=0) -> (deleted portion=w141:string, array with subset deleted=w186:string[])  [unwired: 1 in]
    n26 = call "Elapsed Time"("Reset"="Reset", "Auto Reset"="Auto Reset") -> ("Elapsed Time (s)"=w196:dbl)  [unwired: 10 in, 7 out]
    n27 = case shown="2" "Time Units" {
      tunnel: ["-sec" "-min" "-h"] -> w197
      tunnel: [w226 w230 w233] -> w167
      tunnel: w196 -> [w226 w229 w234]
      frame 0, Default {
      }
      frame 1 {
        n28 = Divide(x=w229, y=60.0) -> (x/y=w230:dbl)
      }
      frame 2 {
        n29 = Divide(x=w234, y=3600.0) -> (x/y=w233:dbl)
      }
    }
    n30 = Add(x=w167, y="Time Offset") -> (x+y=w101:dbl)
    n31 = To Long Integer(number=w101) -> (32bit integer=w102:i32)
    "Elapsed Time" <- w102
    n32 = case shown="\"transfer\"" w141 {
      tunnel: w186 -> [w274 w315 w355 w375 w426 w604 w739 w1005 w1141 w1316 w1393 w1442 w1489 w1532 w1568 _ _ w1766 w1917 _ w2038 w2106 w2171 w2292 w2444 w2530]
      tunnel: w222 -> [w269 w311 w353 w388 w485 w611 w803 w1012 w1205 w1333 w1382 w1434 w1482 w1526 w1561 w1602 w1666 w1747 w1901 w1961 w2025 w2093 w2159 w2286 w2440 w2532]
      tunnel: w221 -> [w268 w310 w344 w387 w470 w582 w774 w983 w1175 w1334 w1383 w1435 w1483 w1527 w1562 w1607 w1668 w1772 w1923 w1965 w2044 w2112 w2177 w2298 w2404 w2536]
      tunnel: w220 -> [w267 w309 w343 w386 w469 w581 w773 w982 w1172 w1335 w1384 w1436 w1484 w1528 w1563 w1606 w1639 w1771 w1922 w1964 w2043 w2111 w2176 w2297 w2403 w2535]
      tunnel: w219 -> [w266 w308 w352 w384 w446 w607 w799 w1008 w1201 w1343 w1392 w1433 w1481 w1525 w1560 w1605 w1663 w1739 w1893 w1970 w2018 w2086 w2152 w2285 w2439 w2537]
      tunnel: w218 -> [w265 w307 w351 w383 w483 w609 w801 w1010 w1203 w1342 w1391 w1441 w1488 w1531 w1567 w1604 w1648 w1770 w1921 w1973 w2042 w2110 w2175 w2296 w2448 w2538]
      tunnel: w217 -> [w264 w306 w350 w381 w482 w608 w800 w1009 w1202 w1341 w1390 w1440 w1487 w1530 w1566 w1603 w1649 w1748 w1902 w1972 w2026 w2094 w2160 w2287 w2441 w2540]
      tunnel: [w268 w310 w342 w387 w480 w606 w798 w1007 w1200 w1334 w1383 w1435 w1483 w1527 w1562 w1607 w1668 w1740 w1875 w1963 w2019 w2087 w2153 w2245 w2406 w2536] -> w216
      tunnel: [w267 w309 w341 w386 w479 w605 w797 w1006 w1199 w1335 w1384 w1436 w1484 w1528 w1563 w1606 w1638 w1749 w1876 w1962 w2027 w2095 w2161 w2244 w2405 w2534] -> w152
      tunnel: [w266 w308 w352 w384 w442 w607 w799 w1008 w1201 w1336 w1385 w1433 w1481 w1525 w1560 w1605 w1663 w1739 w1893 w1970 w2018 w2086 w2152 w2285 w2439 w2537] -> w71
      tunnel: [w265 w307 w351 w383 w483 w609 w801 w1010 w1203 w1342 w1391 w1441 w1488 w1531 w1567 w1604 w1648 w1770 w1921 w1973 w2042 w2110 w2175 w2296 w2448 w2538] -> w215
      tunnel: [w264 w306 w350 w381 w482 w608 w800 w1009 w1202 w1341 w1390 w1440 w1487 w1530 w1566 w1603 w1649 w1748 w1902 w1972 w2026 w2094 w2160 w2287 w2441 w2540] -> w214
      tunnel: [w269 w311 w353 w388 w485 w611 w803 w1012 w1205 w1333 w1382 w1434 w1482 w1526 w1561 w1602 w1666 w1747 w1901 w1961 w2025 w2093 w2159 w2286 w2440 w2532] -> w79
      tunnel: w213 -> [_ _ _ _ w489 w613 w807 w1014 w1209 _ _ _ _ _ _ _ _ w1744 w1898 _ w2024 w2092 w2158 w2264 w2422 _]
      tunnel: "Gate" -> [_ _ _ _ w473 w591 w784 w992 w1186 _ _ _ _ _ _ _ _ _ _ _ _ _ _ _ _ _]
      tunnel: "Drain 2" -> [_ _ _ _ w472 w590 w783 w991 w1185 _ _ _ _ _ _ _ _ _ _ _ _ _ _ _ _ _]
      tunnel: "Panel Controls" -> [_ _ _ _ _ _ w782 w918 w1184 _ _ _ _ _ _ _ _ _ _ _ _ _ _ _ _ _]
      tunnel: w209 -> [w263 w305 w349 w380 w463 w575 w767 w976 w1170 w1340 w1389 _ w1480 w1524 w1559 w1601 w1650 w1735 w1889 w1966 w2014 w2082 w2148 w2281 w2435 w2541]
      tunnel: w208 -> [w262 w304 w348 w379 w462 w574 w766 w975 w1169 w1339 w1388 w1439 _ w1515 w1565 w1600 w1651 w1736 w1890 w1967 w2015 w2083 w2149 w2282 w2436 w2542]
      tunnel: w207 -> [w261 w303 w347 w378 w461 w573 w765 w974 w1168 w1338 w1387 w1438 w1486 w1529 _ w1599 w1652 w1737 w1891 w1968 w2016 w2084 w2150 w2283 w2437 w2543]
      tunnel: w206 -> [w260 w302 w346 w377 w460 w572 w764 w973 w1171 w1337 w1386 w1437 w1485 _ w1564 w1598 w1653 w1738 w1892 w1969 w2017 w2085 w2151 w2284 w2438 w2544]
      tunnel: [w263 w305 w349 w380 w463 w575 w767 w976 w1170 w1340 w1389 w1432 w1480 w1524 w1559 w1601 w1650 w1735 w1889 w1966 w2014 w2082 w2148 w2281 w2435 w2541] -> w205
      tunnel: [w262 w304 w348 w379 w462 w574 w766 w975 w1169 w1339 w1388 w1439 w1472 w1515 w1565 w1600 w1651 w1736 w1890 w1967 w2015 w2083 w2149 w2282 w2436 w2542] -> w204
      tunnel: [w261 w303 w347 w378 w461 w573 w765 w974 w1168 w1338 w1387 w1438 w1486 w1529 w1558 w1599 w1652 w1737 w1891 w1968 w2016 w2084 w2150 w2283 w2437 w2543] -> w203
      tunnel: [w260 w302 w346 w377 w460 w572 w764 w973 w1171 w1337 w1386 w1437 w1485 w1516 w1564 w1598 w1653 w1738 w1892 w1969 w2017 w2085 w2151 w2284 w2438 w2544] -> w202
      tunnel: w201 -> [w244 w283 w324 _ w415 w513 w752 w914 w1158 w1313 w1365 w1416 w1456 w1499 w1542 w1582 w1616 w1722 w1856 w1945 w1985 w2057 w2124 w2231 w2388 w2501]
      tunnel: w200 -> [_ _ _ _ w457 w566 _ _ _ _ _ _ _ _ _ _ _ _ _ _ _ _ _ _ _ _]
      tunnel: [w259 w298 w339 w392 w434 w528 w724 w930 w1124 w1332 w1380 w1431 w1471 w1514 w1557 w1597 w1634 w1712 w1860 w1960 w2003 w2075 w2142 w2206 w2367 w2533] -> w119
      tunnel: w199 -> [w259 w298 w339 w392 w434 w563 w700 w965 w1136 w1332 w1380 w1431 w1471 w1514 w1557 w1597 w1634 w1718 w1860 w1960 w2003 w2075 w2142 w2212 w2373 w2533]
      tunnel: w101 -> [_ _ _ _ w431 w562 w757 w964 w1162 _ _ _ _ _ _ _ w1632 w1727 w1872 _ w2000 w2072 w2139 w2241 w2397 _]
      tunnel: w197 -> [_ _ _ _ w430 w559 w755 w961 w1161 _ _ _ _ _ _ _ w1630 w1725 w1871 _ w1999 w2071 w2138 w2240 w2398 _]
      tunnel: w102 -> [_ _ _ _ _ w555 w740 w957 w1144 _ _ _ _ _ _ _ _ _ _ _ _ _ _ _ _ _]
      tunnel: [w258 w297 w338 w382 w433 w532 w704 w934 w1103 w1331 w1379 w1430 w1470 w1513 w1556 w1596 w1633 w1697 w1844 w1959 w2002 w2074 w2141 w2200 w2362 w2539] -> w153
      tunnel: w195 -> [w258 w297 w338 w382 w433 w558 w741 w960 w1143 w1331 w1379 w1430 w1470 w1513 w1556 w1596 w1633 w1699 w1845 w1959 w2002 w2074 w2141 w2201 w2364 w2539]
      tunnel: [w257 w296 w337 w391 w429 w527 w725 w929 w1125 w1330 w1378 w1429 w1469 w1512 w1555 w1595 w1629 w1711 w1859 w1958 w1998 w2070 w2137 w2205 w2366 w2528] -> w118
      tunnel: w171 -> [w257 w296 w337 w391 w429 w554 w730 w956 w1137 w1330 w1378 w1429 w1469 w1512 w1555 w1595 w1629 w1717 w1859 w1958 w1998 w2070 w2137 w2211 w2372 w2528]
      tunnel: [w256 w295 w336 w376 w428 w547 w754 w949 w1160 w1329 w1377 w1428 w1468 w1511 w1554 w1594 w1628 w1724 w1870 w1957 w1997 w2069 w2136 w2239 w2396 w2527] -> w148
      tunnel: w158 -> [w256 w295 w336 w376 w428 w547 w754 w949 w1160 w1329 w1377 w1428 w1468 w1511 w1554 w1594 w1628 w1724 w1870 w1957 w1997 w2069 w2136 w2239 w2396 w2526]
      tunnel: [w255 w294 w335 w385 w427 w546 w753 w948 w1159 w1328 w1376 w1427 w1467 w1510 w1553 w1593 w1627 w1723 w1869 w1956 w1996 w2068 w2135 w2238 w2395 w2512] -> w149
      tunnel: w151 -> [w255 w294 w335 w385 w427 w546 w753 w948 w1159 w1328 w1376 w1427 w1467 w1510 w1553 w1593 w1627 w1723 w1869 w1956 w1996 w2068 w2135 w2238 w2395 w2512]
      tunnel: [w253 w292 w333 w397 w424 w521 w716 w923 w1119 w1326 w1375 w1426 w1465 w1508 w1551 w1591 w1625 w1705 w1868 w1955 w1995 w2067 w2133 w2237 w2394 w2511] -> w112
      tunnel: w140 -> [w253 w292 w333 w397 w424 w545 w735 w947 w1131 w1326 w1375 w1426 w1465 w1508 w1551 w1591 w1625 w1705 w1868 w1955 w1995 w2067 w2133 w2237 w2394 w2511]
      tunnel: [w254 w293 w334 w398 w425 w522 w717 w924 w1118 w1327 w1374 w1425 w1466 w1509 w1552 w1592 w1626 w1706 w1867 w1954 w1994 w2066 w2134 w2236 w2393 w2510] -> w113
      tunnel: w139 -> [w254 w293 w334 w398 w425 w544 w736 w946 w1130 w1327 w1374 w1425 w1466 w1509 w1552 w1592 w1626 w1706 w1867 w1954 w1994 w2066 w2134 w2236 w2393 w2510]
      tunnel: [w246 w285 w326 w390 w421 w526 w726 w928 w1126 w1319 w1372 w1423 w1463 w1506 w1549 w1589 w1618 w1710 w1858 w1953 w1987 w2059 w2126 w2204 w2369 w2503] -> w117
      tunnel: w128 -> [w246 w285 w326 w390 w421 w540 w731 w942 w1138 w1319 w1372 w1423 w1463 w1506 w1549 w1589 w1618 w1716 w1858 w1953 w1987 w2059 w2126 w2210 w2371 w2503]
      tunnel: [w245 w284 w325 w389 w422 w525 w727 w927 w1127 w1318 w1373 w1424 w1464 w1507 w1550 w1590 w1617 w1709 w1857 w1952 w1986 w2058 w2125 w2203 w2368 w2502] -> w116
      tunnel: w127 -> [w245 w284 w325 w389 w422 w539 w732 w941 w1139 w1318 w1373 w1424 w1464 w1507 w1550 w1590 w1617 w1715 w1857 w1952 w1986 w2058 w2125 w2209 w2370 w2502]
      tunnel: [w248 w287 w328 w394 w420 w531 w722 w933 w1122 w1324 w1370 w1421 w1461 w1504 w1547 w1587 w1620 w1714 w1862 w1947 w1989 w2061 w2128 w2208 w2375 w2507] -> w110
      tunnel: w126 -> [w248 w287 w328 w394 w420 w538 w728 w940 w1134 w1324 w1370 w1421 w1461 w1504 w1547 w1587 w1620 w1720 w1862 w1947 w1989 w2061 w2128 w2214 w2377 w2507]
      tunnel: [w247 w286 w327 w393 w423 w529 w723 w931 w1123 w1325 w1371 w1422 w1462 w1505 w1548 w1588 w1619 w1713 w1861 w1946 w1988 w2060 w2127 w2207 w2365 w2506] -> w120
      tunnel: w125 -> [w247 w286 w327 w393 w423 w537 w729 w939 w1135 w1325 w1371 w1422 w1462 w1505 w1548 w1588 w1619 w1719 w1861 w1946 w1988 w2060 w2127 w2213 w2374 w2506]
      tunnel: [w250 w289 w330 w396 w419 w520 w720 w922 w1120 w1322 w1368 w1419 w1459 w1502 w1545 w1585 w1622 w1704 w1864 w1949 w1991 w2063 w2130 w2233 w2390 w2509] -> w111
      tunnel: w124 -> [w250 w289 w330 w396 w419 w536 w734 w938 w1132 w1322 w1368 w1419 w1459 w1502 w1545 w1585 w1622 w1704 w1864 w1949 w1991 w2063 w2130 w2233 w2390 w2509]
      tunnel: [w249 w288 w329 w395 w418 w519 w721 w921 w1121 w1323 w1369 w1420 w1460 w1503 w1546 w1586 w1621 w1703 w1863 w1948 w1990 w2062 w2129 w2232 w2389 w2508] -> w109
      tunnel: w123 -> [w249 w288 w329 w395 w418 w535 w733 w937 w1133 w1323 w1369 w1420 w1460 w1503 w1546 w1586 w1621 w1703 w1863 w1948 w1990 w2062 w2129 w2232 w2389 w2508]
      tunnel: [w252 w291 w332 w400 w417 w524 w719 w926 w1116 w1320 w1366 w1417 w1457 w1500 w1543 w1583 w1624 w1708 w1866 w1951 w1993 w2065 w2132 w2235 w2392 w2505] -> w115
      tunnel: w122 -> [w252 w291 w332 w400 w417 w534 w738 w936 w1128 w1320 w1366 w1417 w1457 w1500 w1543 w1583 w1624 w1708 w1866 w1951 w1993 w2065 w2132 w2235 w2392 w2505]
      tunnel: [w251 w290 w331 w399 w416 w523 w718 w925 w1117 w1321 w1367 w1418 w1458 w1501 w1544 w1584 w1623 w1707 w1865 w1950 w1992 w2064 w2131 w2234 w2391 w2504] -> w114
      tunnel: w121 -> [w251 w290 w331 w399 w416 w533 w737 w935 w1129 w1321 w1367 w1418 w1458 w1501 w1544 w1584 w1623 w1707 w1865 w1950 w1992 w2064 w2131 w2234 w2391 w2504]
      tunnel: [w244 w283 w324 w366 w415 w513 w752 w914 w1158 w1313 w1365 w1416 w1456 w1499 w1542 w1582 w1616 w1722 w1856 w1945 w1985 w2057 w2124 w2231 w2388 w2501] -> w70
      tunnel: w101 -> [_ _ _ _ _ _ _ _ _ _ _ _ _ _ _ _ _ w1674 w1840 _ _ _ _ w2215 w2381 _]
      tunnel: [w243 w282 w323 w365 w414 w512 w711 w913 w1109 w1312 w1364 w1415 w1455 w1498 w1541 w1581 w1615 w1686 w1855 w1944 w1984 w2056 w2123 w2221 w2384 w2500] -> w75
      tunnel: [w242 w281 w322 w364 w413 w511 w712 w912 w1110 w1311 w1363 w1414 w1454 w1497 w1540 w1580 w1614 w1683 w1854 w1943 w1983 w2055 w2122 w2182 w2345 w2499] -> w76
      tunnel: [w241 w280 w321 w363 w412 w510 w713 w911 w1111 w1310 w1362 w1413 w1453 w1496 w1539 w1579 w1613 w1684 w1827 w1942 w1982 w2054 w2121 w2194 w2357 w2498] -> w77
      tunnel: [w240 w279 w320 w362 w411 w509 w714 w910 w1112 w1309 w1361 w1412 w1452 w1495 w1538 w1578 w1612 w1685 w1834 w1941 w1981 w2053 w2120 w2190 w2353 w2497] -> w78
      tunnel: w100 -> [w243 w282 w323 w365 w414 w512 w711 w913 w1109 w1312 w1364 w1415 w1455 w1498 w1541 w1581 w1615 w1690 w1855 w1944 w1984 w2056 w2123 w2224 w2387 w2500]
      tunnel: w99 -> [w242 w281 w322 w364 w413 w511 w712 w912 w1110 w1311 w1363 w1414 w1454 w1497 w1540 w1580 w1614 w1689 w1854 w1943 w1983 w2055 w2122 w2223 w2386 w2499]
      tunnel: w98 -> [w241 w280 w321 w363 w412 w510 w713 w911 w1111 w1310 w1362 w1413 w1453 w1496 w1539 w1579 w1613 w1688 w1828 w1942 w1982 w2054 w2121 w2194 w2357 w2498]
      tunnel: w97 -> [w240 w279 w320 w362 w411 w509 w714 w910 w1112 w1309 w1361 w1412 w1452 w1495 w1538 w1578 w1612 w1687 w1836 w1941 w1981 w2053 w2120 w2222 w2385 w2497]
      tunnel: "Standby" -> [_ _ _ _ w410 w508 _ w909 _ _ _ _ _ _ _ _ _ w1681 w1853 _ _ _ _ w2230 _ _]
      tunnel: w69 -> [w239 w278 w319 w361 w404 w503 w709 w903 w1107 w1308 w1360 w1411 w1451 w1494 w1537 w1577 w1611 w1672 w1848 w1940 w1977 w2050 w2118 w2188 w2351 w2496]
      tunnel: w68 -> [w238 w277 w318 w360 w403 w502 w710 w904 w1108 w1307 w1359 w1410 w1450 w1493 w1536 w1576 w1610 w1671 w1847 w1939 w1976 w2049 w2117 w2187 w2350 w2495]
      tunnel: [w239 w278 w319 w361 w404 w503 w709 w903 w1107 w1308 w1360 w1411 w1451 w1494 w1537 w1577 w1611 w1672 w1848 w1940 w1977 w2050 w2118 w2183 w2346 w2496] -> w67
      tunnel: [w238 w277 w318 w360 w403 w502 w710 w904 w1108 w1307 w1359 w1410 w1450 w1493 w1536 w1576 w1610 w1671 w1847 w1939 w1976 w2049 w2117 w2186 w2349 w2495] -> w66
      tunnel: w65 -> [w237 w276 w317 w359 w401 w500 w707 w901 w1105 w1305 w1357 w1408 w1448 w1491 w1534 w1574 w1608 w1670 w1833 w1938 w1975 w2048 w2116 w2181 w2344 w2494]
      tunnel: w64 -> [w236 w275 w316 w358 w402 w501 w708 w902 w1106 w1306 w1358 w1409 w1449 w1492 w1535 w1575 w1609 w1669 w1832 w1937 w1974 w2047 w2115 w2180 w2343 w2493]
      tunnel: [w237 w276 w317 w359 w401 w500 w707 w901 w1105 w1305 w1357 w1408 w1448 w1491 w1534 w1574 w1608 w1670 w1825 w1938 w1975 w2048 w2116 w2181 w2344 w2494] -> w63
      tunnel: [w236 w275 w316 w358 w402 w501 w708 w902 w1106 w1306 w1358 w1409 w1449 w1492 w1535 w1575 w1609 w1669 w1831 w1937 w1974 w2047 w2115 w2180 w2343 w2493] -> w62
      frame "wait" {
        n33 = Index Array(array=w274, index=0 ("Index")) -> (element=w272:string)
        n34 = Decimal String To Number(string=w272, default (0L)=u32 0) -> (number=w271:u32)  [unwired: 1 in, 1 out]
        n35 = Wait (ms)(milliseconds to wait=w271) -> ()  [unwired: 1 out]
      }
      frame "wait-min" {
        n36 = Index Array(array=w315, index=0 ("Index")) -> (element=w313:string)
        n37 = Decimal String To Number(string=w313, default (0L)=u32 0) -> (number=w301:u32)  [unwired: 1 in, 1 out]
        n38 = Multiply(x=w301, y=u32 60000) -> (x*y=w300:u32)
        n39 = Wait (ms)(milliseconds to wait=w300) -> ()  [unwired: 1 out]
      }
      frame "standby" {
        n40 = Index Array(array=w355, index=0 ("Index")) -> (element=w345:string)
        n41 = case shown="\"off\", Default" w345 {
          tunnel: [":PAGE:SCON:STAN 0" ":PAGE:SCON:STAN 1"] -> w340
          frame "off", Default {
          }
          frame "on" {
          }
        }
        n42 = VISA Write(VISA resource name=w344, write buffer=w340, error in (no error)=w343) -> (VISA resource name out=w342:refnum<visa-resource-name>, error out=w341:errorcluster)  [unwired: 1 out]
      }
      frame "Probe4" {
        n43 = Delete From Array(array=w375, index=0) -> (deleted portion=w369:string, array with subset deleted=w372:string[])  [unwired: 1 in]
        n44 = Equal?(x=w369, y="ON") -> (x = y?=w367:bool)
        n45 = Delete From Array(array=w372, index=0) -> (deleted portion=w371:string)  [unwired: 1 in, 1 out]
        n46 = Fract/Exp String To Number(string=w371) -> (number=w368:dbl)  [unwired: 3 in, 1 out]
        n47 = Bundle(w367, w368) -> (w366:cluster{bool, dbl})  [unwired: 1 in]
      }
      frame "pulsedstressV" {
        w440 = 0
        n48 = local read "Pulsed Stress V - Vextra"() -> (w407:u32)
        n49 = local read "Pulsed Stress V - Drain"() -> (w409:u32)
        n50 = local read "Pulsed Stress V - Gate"() -> (w406:u32)
        n51 = local read "Pulsed Stress V - Probe 4"() -> (w408:u32)
        n52 = local read "Pulsed Stress V - Source/Common"() -> (w405:u32)
        n53 = Number To Decimal String(number=w431) -> (decimal integer string=w486:string)  [unwired: 1 in]
        n54 = Delete From Array(array=w426, index=0 ("Index")) -> (deleted portion=w477:string, array with subset deleted=w476:string[])  [unwired: 1 in]
        n55 = Bundle By Name(cluster=w457, "Emergency Stop"=w489) -> (w458:T2)
        n56 = VISA Write(VISA resource name=w470, write buffer=":PAGE:CHAN:MODE SWE;" ("write buffer (\"\")"), error in (no error)=w469) -> (VISA resource name out=w467:refnum<visa-resource-name>, error out=w468:errorcluster)  [unwired: 1 out]
        n57 = Concatenate Strings(w485, "-pulsedstressV-" ("Substring"), w486, w430, ".txt" ("Substring")) -> (w488:string)
        n58 = case shown="\"d\", Default" w477 {
          tunnel: [w498 w499] -> w475
          frame "s" {
            w498 = u16 0 items=["Single", "Double"] ("sweep mode")
          }
          frame "d", Default {
            w499 = u16 1 items=["Single", "Double"] ("sweep mode")
          }
        }
        n59 = Fract/Exp String To Number(string=w476) -> (number=w471:dbl[])  [unwired: 3 in, 1 out]
        n60 = String To Path(string=w488) -> (path=w484:path)
        n61 = Index Array(array=w471, index #1=0 ("Index")) -> (element #1=w449:dbl, element #2=w448:dbl, element #3=w445:dbl, element #4=w444:dbl, element #5=w443:dbl, element #6=w447:dbl)  [unwired: 5 in]
        n62 = Bundle By Name(cluster=w446, "Pulse period"=w444, "Base voltage"=w445, "Pulse width"=w443) -> (w442:T4)
        n63 = Unbundle By Name(w442) -> ("Pulse period"=w450:dbl)
        n64 = Bundle By Name(cluster=w473, "Gate Start"=w448, "Gate Stop"=w449, "Gate Step (linear only)"=0, "Gate Compliance"=w482, "Range mode"=w463, "Range"=w462) -> (w464:T6)
        n65 = call <vilib>:"compatOverwrite.vi"("overwrite (F)"=TRUE) -> ("overwrite?"=w435:T8)
        n66 = Bundle By Name(cluster=w472, "Drain Start"=w447, "Drain Stop"=w440, "Drain Step"=w440, "Drain Compliance"=w483, "Range mode"=w461, "Range"=w460) -> (w465:T7)
        n67 = call "4155C PulsedStressV v3.0.vi"("VISA resource name in"=w467, "Gate"=w464, "Pulsed Stress V - Source/Common"=w405, "Drain"=w465, "Timings"=w442, "error in (no error)"=w468, "sweep mode"=w475, "Probe 4"=w415, "Pulsed Stress V - Drain"=w409, "Pulsed Stress V - Gate"=w406, "Panel Controls"=w458, "Standby"=w410, "Pulsed Stress V - Probe 4"=w408, "Pulsed Stress V - Vextra"=w407) -> ("Outparams"=w459:T9, "VISA Resource Name out"=w480:refnum<visa-resource-name>, "ID"=w438:dbl[], "IG"=w436:dbl[], "error out"=w481:errorcluster)  [unwired: 1 in]
        n68 = Unbundle By Name(w459) -> ("Number of points"=w437:i32)  [unwired: 2 out]
        n69 = for {
          N: w437 -> [_]
          tunnel: [w495] -> w439 mode=indexing
          tunnel: w450 -> [w497]
          i -> [w496]
          n70 = Multiply(x=w497, y=w496) -> (x*y=w495:dbl)
        }
        n71 = Insert Into Array(array=dbl[][] [] ("Input Array"), new element=w439) -> (w451:dbl[][])  [unwired: 2 in]
        n72 = Insert Into Array(array=w451, new element=w438) -> (w456:dbl[][])  [unwired: 2 in]
        n73 = Insert Into Array(array=w456, new element=w436) -> (w455:dbl[][])  [unwired: 2 in]
        n74 = Transpose 2D Array(2D array=w455) -> (transposed array=w454:dbl[][])
        n75 = Open/Create/Replace File(file path (use dialog)=w484, error in=w481, operation (0:open)=w435) -> (refnum out=w492:refnum<file>, error out=w493:errorcluster)  [unwired: 3 in, 1 out]
        n76 = call "4155C Write array to file.vi"("Byte Stream File Refnum"=w492, "Header"=string[] ["Time /s", "Id /A", "Ig /A"], "Data Array"=w454, "error in (no error)"=w493) -> ("dup refnum"=w490:refnum<file>, "error out"=w491:errorcluster)  [unwired: 1 in]
        n77 = Close File(refnum=w490, error in=w491) -> (error out=w479:errorcluster)  [unwired: 1 out]
      }
      frame "transfer" {
        n78 = local read "Transfer/Output - Gate"() -> (w507:u32)
        n79 = Delete From Array(array=w604, index=0 ("Index")) -> (deleted portion=w602:string, array with subset deleted=w601:string[])  [unwired: 1 in]
        n80 = Bundle By Name(cluster=w566, "Emergency Stop"=w613) -> (w567:T2)
        n81 = Number To Decimal String(number=w562) -> (decimal integer string=w561:string)  [unwired: 1 in]
        n82 = case shown="\"d\", Default" w602 {
          tunnel: [w698 w699] -> w600
          frame "s" {
            w698 = u16 0 items=["Single", "Double"] ("sweep mode")
          }
          frame "d", Default {
            w699 = u16 1 items=["Single", "Double"] ("sweep mode")
          }
        }
        n83 = Fract/Exp String To Number(string=w601) -> (number=w586:dbl[])  [unwired: 3 in, 1 out]
        n84 = Concatenate Strings(w611, "-transfer-" ("Prefix"), w561, w559, ".txt" ("Suffix (transfer)")) -> (w612:string)
        n85 = VISA Write(VISA resource name=w582, write buffer=":PAGE:CHAN:MODE SWE;" ("write buffer (\"\")"), error in (no error)=w581) -> (VISA resource name out=w579:refnum<visa-resource-name>, error out=w580:errorcluster)  [unwired: 1 out]
        n86 = local read "Plot transfer curve extrema vs time"() -> (w514:bool)
        n87 = String To Path(string=w612) -> (path=w610:path)
        n88 = Index Array(array=w586, index #1=0 ("Index")) -> (element #1=w599:dbl, element #2=w598:dbl, element #3=w597:dbl)  [unwired: 2 in]
        n89 = Delete From Array(array=w586, length=3 ("Length"), index=0 ("Index")) -> (array with subset deleted=w584:dbl[])  [unwired: 1 out]
        n90 = local read "Transfer/Output - Drain"() -> (w504:u32)
        n91 = local read "Transfer/Output - Source/Common"() -> (w506:u32)
        n92 = case shown="True" w514 {
          tunnel: w558 -> [w615 w618]
          tunnel: w555 -> [_ w617]
          tunnel: [w615 w616] -> w532
          frame False {
          }
          frame True {
            n93 = Build Array (concatenate)(w618, w617) -> (w616:i32[])
          }
        }
        n94 = local read "Transfer/Output - Probe 4"() -> (w505:u32)
        n95 = Bundle By Name(cluster=w591, "Gate Start"=w599, "Gate Stop"=w598, "Gate Step (linear only)"=w597, "Gate Compliance"=w608, "Range mode"=w575, "Range"=w574) -> (w576:T6)
        n96 = Index Array(array=w584, index #1=0 ("Index")) -> (element #1=w594:dbl, element #2=w593:dbl, element #3=w592:dbl)  [unwired: 2 in]
        n97 = call <vilib>:"compatOverwrite.vi"("overwrite (F)"=TRUE) -> ("overwrite?"=w565:T8)
        n98 = Bundle By Name(cluster=w590, "Drain Start"=w594, "Drain Stop"=w593, "Drain Step"=w592, "Drain Compliance"=w609, "Range mode"=w573, "Range"=w572) -> (w577:T7)
        n99 = call "4155C Transfer v3.0.vi"("VISA resource name in"=w579, "Source/Common"=w506, 2:"Gate"=w576, 3:"Drain"=w577, 4:"Drain"=w504, "Timings"=w607, "error in (no error)"=w580, 7:"Probe 4"=w513, 8:"Gate"=w507, 9:"Probe 4"=w505, "sweep mode"=w600, "Panel Controls"=w567, "Standby"=w508) -> ("VG"=w564:dbl[], "Outparams"=w571:T9, "VISA Resource Name out"=w606:refnum<visa-resource-name>, "IS"=w542:dbl[], "ID"=w543:dbl[], "IG"=w541:dbl[], "error out"=w556:errorcluster, "Probe 4"=w568:dbl[])  [unwired: 7 in]
        n100 = Unbundle By Name(w571) -> ("V2 Step"=w570:dbl, "V2 Start"=w569:dbl, "Number of points"=w530:i32)
        n101 = call "4155C Split array.vi"("Number of VAR2 steps"=w530, "Y2 data in"=w543, "X data in"=w564, "Y1 data in"=w542, "Y3 data in"=w541, "error in (no error)"=w556) -> ("Array of clusters"=w557:cluster{"Y data in":dbl[], "X data in":dbl[]}[], "error out"=w518:errorcluster)  [unwired: 1 in]
        n102 = case shown="True" "Plot transfer curve extrema vs time" {
          tunnel: w563 -> [w621 w697]
          tunnel: w554 -> [w622 w692]
          tunnel: w545 -> [w628 w688]
          tunnel: w544 -> [w629 w687]
          tunnel: w543 -> [_ w684]
          tunnel: w542 -> [_ w682]
          tunnel: w541 -> [_ w681]
          tunnel: w540 -> [w623 w677]
          tunnel: w539 -> [w625 w676]
          tunnel: w538 -> [w619 w673]
          tunnel: w537 -> [w620 w672]
          tunnel: w536 -> [w627 w669]
          tunnel: w535 -> [w626 w668]
          tunnel: w534 -> [w631 w665]
          tunnel: w533 -> [w630 w664]
          tunnel: w532 -> [_ w657]
          tunnel: [w619 w652] -> w531
          tunnel: w530 -> [_ w651]
          tunnel: [w620 w650] -> w529
          tunnel: [w621 w649] -> w528
          tunnel: [w622 w648] -> w527
          tunnel: [w623 w647] -> w526
          tunnel: [w625 w646] -> w525
          tunnel: [w631 w645] -> w524
          tunnel: [w630 w644] -> w523
          tunnel: [w629 w643] -> w522
          tunnel: [w628 w642] -> w521
          tunnel: [w627 w641] -> w520
          tunnel: [w626 w640] -> w519
          tunnel: w518 -> [w624 w639]
          tunnel: [w624 w635] -> w517
          frame False {
          }
          frame True {
            # "Adjusts graph colors."
            # "Adjusts graph colors."
            # "Ion will be the middle element of the array. The calculation of the index is done only once, since Is, Id, and Ig have the same dimensions."
            # "abs(Ig)"
            # "abs(Is)"
            # "Y1: Is\nY2: Id\nY3: Ig"
            # "abs(Id)"
            # "Adjusts graph colors."
            # "Adjusts graph colors."
            # "Adjusts graph colors."
            n103 = Absolute Value(x=w682) -> (abs(x)=w667:dbl[])
            n104 = Absolute Value(x=w684) -> (abs(x)=w683:dbl[])
            n105 = Absolute Value(x=w681) -> (abs(x)=w670:dbl[])
            n106 = Array Size(array=w683) -> (size(s)=w691:i32)
            n107 = Divide(x=w691, y=2) -> (x/y=w634:dbl)
            n108 = Subtract(x=w634, y=1) -> (x-y=w633:dbl)
            n109 = Array Max & Min(array=w667) -> (max value=w674:dbl, min value=w675:dbl)  [unwired: 2 out]
            n110 = Array Max & Min(array=w683) -> (max value=w696:dbl, min value=w680:dbl)  [unwired: 2 out]
            n111 = Array Max & Min(array=w670) -> (max value=w679:dbl, min value=w678:dbl)  [unwired: 2 out]
            n112 = Index Array(array=w667, index=w633) -> (element=w658:dbl)
            n113 = Index Array(array=w667, index=0) -> (element=w659:dbl)
            n114 = Index Array(array=w683, index=w633) -> (element=w660:dbl)
            n115 = Index Array(array=w683, index=0) -> (element=w661:dbl)
            n116 = Index Array(array=w670, index=w633) -> (element=w663:dbl)
            n117 = Index Array(array=w670, index=0) -> (element=w662:dbl)
            n118 = local write "Ig max"(w679) -> ()
            n119 = local write "Ig min"(w678) -> ()
            n120 = local write "Is max"(w674) -> ()
            n121 = local write "Is min"(w675) -> ()
            n122 = local write "Id max"(w696) -> ()
            n123 = local write "Id min"(w680) -> ()
            n124 = Build Array (concatenate)(w673, w674) -> (w652:dbl[])
            n125 = Build Array (concatenate)(w672, w675) -> (w650:dbl[])
            n126 = local write "Is off"(w659) -> ()
            n127 = local write "Is on"(w658) -> ()
            n128 = Build Array (concatenate)(w697, w696) -> (w649:dbl[])
            n129 = Build Array (concatenate)(w692, w680) -> (w648:dbl[])
            n130 = Build Array (concatenate)(w677, w679) -> (w647:dbl[])
            n131 = Build Array (concatenate)(w676, w678) -> (w646:dbl[])
            n132 = Build Array (concatenate)(w665, w658) -> (w645:dbl[])
            n133 = Build Array (concatenate)(w664, w659) -> (w644:dbl[])
            n134 = Build Array (concatenate)(w687, w660) -> (w643:dbl[])
            n135 = Build Array (concatenate)(w688, w661) -> (w642:dbl[])
            n136 = Build Array (concatenate)(w669, w663) -> (w641:dbl[])
            n137 = Build Array (concatenate)(w668, w662) -> (w640:dbl[])
            n138 = local write "Ig off"(w662) -> ()
            n139 = local write "Ig on"(w663) -> ()
            n140 = local write "Id off"(w661) -> ()
            n141 = local write "Id on"(w660) -> ()
            n142 = control-ref of="Imax vs time"() -> (w686:refnum<vi>)
            n143 = control-ref of="Imin vs time"() -> (w685:refnum<vi>)
            n144 = control-ref of="Ion vs time"() -> (w654:refnum<vi>)
            n145 = control-ref of="Ioff vs time"() -> (w653:refnum<vi>)
            n146 = control-ref of="I vs Vg"() -> (w695:refnum<vi>)
            n147 = call "4155C Split array.vi"("Number of VAR2 steps"=w651, "Y2 data in"=w643, "X data in"=w657, "Y1 data in"=w645, "Y3 data in"=w641, "error in (no error)"=w639) -> ("Array of clusters"=w655:cluster{"Y data in":dbl[], "X data in":dbl[]}[], "error out"=w638:errorcluster)  [unwired: 1 in]
            n148 = call "4155C Split array.vi"("Number of VAR2 steps"=w651, "Y2 data in"=w642, "X data in"=w657, "Y1 data in"=w644, "Y3 data in"=w640, "error in (no error)"=w638) -> ("Array of clusters"=w656:cluster{"Y data in":dbl[], "X data in":dbl[]}[], "error out"=w637:errorcluster)  [unwired: 1 in]
            n149 = call "4155C Split array.vi"("Number of VAR2 steps"=w651, "Y2 data in"=w649, "X data in"=w657, "Y1 data in"=w652, "Y3 data in"=w647, "error in (no error)"=w637) -> ("Array of clusters"=w694:cluster{"Y data in":dbl[], "X data in":dbl[]}[], "error out"=w636:errorcluster)  [unwired: 1 in]
            n150 = call "4155C Split array.vi"("Number of VAR2 steps"=w651, "Y2 data in"=w648, "X data in"=w657, "Y1 data in"=w650, "Y3 data in"=w646, "error in (no error)"=w636) -> ("Array of clusters"=w693:cluster{"Y data in":dbl[], "X data in":dbl[]}[], "error out"=w635:errorcluster)  [unwired: 1 in]
            n151 = call "4155C Config Chart Colours.vi"("Numeric"=w651, "XY Graph 2"=w686) -> ()  [unwired: 6 in]
            n152 = call "4155C Config Chart Colours.vi"("Numeric"=w651, "XY Graph 2"=w685) -> ()  [unwired: 6 in]
            n153 = call "4155C Config Chart Colours.vi"("Numeric"=w651, "XY Graph 2"=w654) -> ()  [unwired: 6 in]
            n154 = call "4155C Config Chart Colours.vi"("Numeric"=w651, "XY Graph 2"=w653) -> ()  [unwired: 6 in]
            n155 = call "4155C Config Chart Colours.vi"("Numeric"=w651, "XY Graph 2"=w695) -> ()  [unwired: 6 in]
            n156 = local write "Imax vs time"(w694) -> ()
            n157 = local write "Imin vs time"(w693) -> ()
            n158 = local write "Ion vs time"(w655) -> ()
            n159 = local write "Ioff vs time"(w656) -> ()
          }
        }
        n160 = local write "I vs Vg"(w557) -> ()
        n161 = Open/Create/Replace File(file path (use dialog)=w610, error in=w517, operation (0:open)=w565) -> (refnum out=w552:refnum<file>, error out=w550:errorcluster)  [unwired: 3 in, 1 out]
        n162 = call "4155C Make Big 2d array.vi"("1D Var1"=w564, "1d IS"=w542, "1d ID"=w543, "1d IG"=w541, "1d SMU4"=w568, "SMU4"=w513, "VAR2 START"=w569, "Number of VAR2 steps"=w530, "VAR2 STEP"=w570, "VAR1 Name"="Vg", "Decimal places in header"=i8 1, "VAR2 Name"="Vd") -> ("Header array"=w553:string[], "Data array"=w551:dbl[][])  [unwired: 14 in]
        n163 = call "4155C Write array to file.vi"("Byte Stream File Refnum"=w552, "Header"=w553, "Data Array"=w551, "error in (no error)"=w550) -> ("dup refnum"=w549:refnum<file>, "error out"=w548:errorcluster)  [unwired: 1 in]
        n164 = Close File(refnum=w549, error in=w548) -> (error out=w605:errorcluster)  [unwired: 1 out]
      }
      frame "transfer-fpp" {
        # "Adjusts graph colors."
        # "Y1 = Y2 = ID\nY3 = IG"
        n165 = local read "Plot transfer curve extrema vs time"() -> (w715:bool)
        n166 = Number To Decimal String(number=w757) -> (decimal integer string=w804:string)  [unwired: 1 in]
        n167 = Bundle By Name(cluster=w782, "Emergency Stop"=w807) -> (w815:T1)
        n168 = Delete From Array(array=w739, index=0 ("Index")) -> (deleted portion=w795:string, array with subset deleted=w794:string[])  [unwired: 1 in]
        n169 = local read "FPP - Source"() -> (w751:u32)
        n170 = local read "FPP - Drain"() -> (w749:u32)
        n171 = local read "FPP - Gate"() -> (w750:u32)
        n172 = Concatenate Strings(w803, "-transferfpp-" ("Substring"), w804, w755, ".txt" ("Substring")) -> (w806:string)
        n173 = VISA Write(VISA resource name=w774, write buffer=":PAGE:CHAN:MODE SWE;" ("write buffer (\"\")"), error in (no error)=w773) -> (VISA resource name out=w771:refnum<visa-resource-name>, error out=w772:errorcluster)  [unwired: 1 out]
        n174 = case shown="\"d\", Default" w795 {
          tunnel: [w899 w900] -> w793
          frame "s" {
            w899 = u16 0 items=["Single", "Double"] ("sweep mode")
          }
          frame "d", Default {
            w900 = u16 1 items=["Single", "Double"] ("sweep mode")
          }
        }
        n175 = Fract/Exp String To Number(string=w794) -> (number=w778:dbl[])  [unwired: 3 in, 1 out]
        n176 = local read "Plot transfer curve extrema vs time"() -> (w742:bool)
        n177 = String To Path(string=w806) -> (path=w802:path)
        n178 = Index Array(array=w778, index #1=0 ("Index")) -> (element #1=w792:dbl, element #2=w791:dbl, element #3=w790:dbl)  [unwired: 2 in]
        n179 = Delete From Array(array=w778, length=3 ("Length"), index=0 ("Index")) -> (array with subset deleted=w776:dbl[])  [unwired: 1 out]
        n180 = local read "FPP - Probe 1"() -> (w747:u32)
        n181 = local read "FPP - Probe 2"() -> (w748:u32)
        n182 = control-ref of="I vs Vg"() -> (w743:refnum<vi>)
        n183 = case shown="True" w742 {
          tunnel: w741 -> [w895 w898]
          tunnel: [w895 w897] -> w704
          tunnel: w740 -> [_ w896]
          frame False {
          }
          frame True {
            n184 = Build Array (concatenate)(w898, w896) -> (w897:i32[])
          }
        }
        n185 = Bundle By Name(cluster=w784, "Gate Start"=w792, "Gate Stop"=w791, "Gate Step (linear only)"=w790, "Gate Compliance"=w800, "Range mode"=w767, "Range"=w766) -> (w768:T6)
        n186 = Index Array(array=w776, index #1=0 ("Index")) -> (element #1=w787:dbl, element #2=w786:dbl, element #3=w785:dbl)  [unwired: 2 in]
        n187 = call <vilib>:"compatOverwrite.vi"("overwrite (F)"=TRUE) -> ("overwrite?"=w758:T8)
        n188 = Bundle By Name(cluster=w783, "Drain Start"=w787, "Drain Stop"=w786, "Drain Step"=w785, "Drain Compliance"=w801, "Range mode"=w765, "Range"=w764) -> (w769:T7)
        n189 = call "4155C Transfer-FPP v3.0.vi"("VISA resource name in"=w771, "FPP - Source"=w751, "Gate"=w768, "Drain"=w769, "FPP - Drain"=w749, "Timings"=w799, "error in (no error)"=w772, "FPP - Gate"=w750, "FPP - Probe 1"=w747, "sweep mode"=w793, "FPP - Probe 2"=w748, "Panel Controls"=w815) -> ("VG"=w745:dbl[], "Outparams"=w763:T9, "VISA Resource Name out"=w798:refnum<visa-resource-name>, "Vprobe2"=w760:dbl[], "ID"=w701:dbl[], "IG"=w703:dbl[], "Vprobe1"=w759:dbl[], "error out"=w706:errorcluster)  [unwired: 8 in]
        n190 = Unbundle By Name(w763) -> ("V2 Step"=w762:dbl, "V2 Start"=w761:dbl, "Number of points"=w702:i32)
        n191 = case shown="True" w715 {
          tunnel: w700 -> [w818 w894]
          tunnel: w730 -> [w819 w889]
          tunnel: w735 -> [w825 w885]
          tunnel: w736 -> [w826 w884]
          tunnel: w701 -> [_ w881]
          tunnel: w701 -> [_ w879]
          tunnel: w703 -> [_ w878]
          tunnel: w731 -> [w820 w874]
          tunnel: w732 -> [w822 w873]
          tunnel: w728 -> [w816 w870]
          tunnel: w729 -> [w817 w869]
          tunnel: w734 -> [w824 w866]
          tunnel: w733 -> [w823 w865]
          tunnel: w738 -> [w828 w862]
          tunnel: w737 -> [w827 w861]
          tunnel: w704 -> [_ w854]
          tunnel: [w816 w849] -> w722
          tunnel: w702 -> [_ w848]
          tunnel: [w817 w847] -> w723
          tunnel: [w818 w846] -> w724
          tunnel: [w819 w845] -> w725
          tunnel: [w820 w844] -> w726
          tunnel: [w822 w843] -> w727
          tunnel: [w828 w842] -> w719
          tunnel: [w827 w841] -> w718
          tunnel: [w826 w840] -> w717
          tunnel: [w825 w839] -> w716
          tunnel: [w824 w838] -> w720
          tunnel: [w823 w837] -> w721
          tunnel: w706 -> [w821 w836]
          tunnel: [w821 w832] -> w705
          frame False {
          }
          frame True {
            # "Y1 = Y2 = ID\nY3 = IG"
            # "Adjusts graph colors."
            # "Adjusts graph colors."
            # "Ion will be the middle element of the array. The calculation of the index is done only once, since Is, Id, and Ig have the same dimensions."
            # "abs(Ig)"
            # "abs(Is)"
            # "abs(Id)"
            # "Adjusts graph colors."
            # "Adjusts graph colors."
            # "Adjusts graph colors."
            n192 = Absolute Value(x=w879) -> (abs(x)=w864:dbl[])
            n193 = Absolute Value(x=w881) -> (abs(x)=w880:dbl[])
            n194 = Absolute Value(x=w878) -> (abs(x)=w867:dbl[])
            n195 = Array Size(array=w880) -> (size(s)=w888:i32)
            n196 = Divide(x=w888, y=2) -> (x/y=w831:dbl)
            n197 = Subtract(x=w831, y=1) -> (x-y=w830:dbl)
            n198 = Array Max & Min(array=w864) -> (max value=w871:dbl, min value=w872:dbl)  [unwired: 2 out]
            n199 = Array Max & Min(array=w880) -> (max value=w893:dbl, min value=w877:dbl)  [unwired: 2 out]
            n200 = Array Max & Min(array=w867) -> (max value=w876:dbl, min value=w875:dbl)  [unwired: 2 out]
            n201 = Index Array(array=w864, index=w830) -> (element=w855:dbl)
            n202 = Index Array(array=w864, index=0) -> (element=w856:dbl)
            n203 = Index Array(array=w880, index=w830) -> (element=w857:dbl)
            n204 = Index Array(array=w880, index=0) -> (element=w858:dbl)
            n205 = Index Array(array=w867, index=w830) -> (element=w860:dbl)
            n206 = Index Array(array=w867, index=0) -> (element=w859:dbl)
            n207 = local write "Ig max"(w876) -> ()
            n208 = local write "Ig min"(w875) -> ()
            n209 = local write "Is max"(w871) -> ()
            n210 = local write "Is min"(w872) -> ()
            n211 = local write "Id max"(w893) -> ()
            n212 = local write "Id min"(w877) -> ()
            n213 = Build Array (concatenate)(w870, w871) -> (w849:dbl[])
            n214 = Build Array (concatenate)(w869, w872) -> (w847:dbl[])
            n215 = local write "Is off"(w856) -> ()
            n216 = local write "Is on"(w855) -> ()
            n217 = Build Array (concatenate)(w894, w893) -> (w846:dbl[])
            n218 = Build Array (concatenate)(w889, w877) -> (w845:dbl[])
            n219 = Build Array (concatenate)(w874, w876) -> (w844:dbl[])
            n220 = Build Array (concatenate)(w873, w875) -> (w843:dbl[])
            n221 = Build Array (concatenate)(w862, w855) -> (w842:dbl[])
            n222 = Build Array (concatenate)(w861, w856) -> (w841:dbl[])
            n223 = Build Array (concatenate)(w884, w857) -> (w840:dbl[])
            n224 = Build Array (concatenate)(w885, w858) -> (w839:dbl[])
            n225 = Build Array (concatenate)(w866, w860) -> (w838:dbl[])
            n226 = Build Array (concatenate)(w865, w859) -> (w837:dbl[])
            n227 = local write "Ig off"(w859) -> ()
            n228 = local write "Ig on"(w860) -> ()
            n229 = local write "Id off"(w858) -> ()
            n230 = local write "Id on"(w857) -> ()
            n231 = control-ref of="Imax vs time"() -> (w883:refnum<vi>)
            n232 = control-ref of="Imin vs time"() -> (w882:refnum<vi>)
            n233 = control-ref of="Ion vs time"() -> (w851:refnum<vi>)
            n234 = control-ref of="Ioff vs time"() -> (w850:refnum<vi>)
            n235 = control-ref of="I vs Vg"() -> (w892:refnum<vi>)
            n236 = call "4155C Split array.vi"("Number of VAR2 steps"=w848, "Y2 data in"=w840, "X data in"=w854, "Y1 data in"=w842, "Y3 data in"=w838, "error in (no error)"=w836) -> ("Array of clusters"=w852:cluster{"Y data in":dbl[], "X data in":dbl[]}[], "error out"=w835:errorcluster)  [unwired: 1 in]
            n237 = call "4155C Split array.vi"("Number of VAR2 steps"=w848, "Y2 data in"=w839, "X data in"=w854, "Y1 data in"=w841, "Y3 data in"=w837, "error in (no error)"=w835) -> ("Array of clusters"=w853:cluster{"Y data in":dbl[], "X data in":dbl[]}[], "error out"=w834:errorcluster)  [unwired: 1 in]
            n238 = call "4155C Split array.vi"("Number of VAR2 steps"=w848, "Y2 data in"=w846, "X data in"=w854, "Y1 data in"=w849, "Y3 data in"=w844, "error in (no error)"=w834) -> ("Array of clusters"=w891:cluster{"Y data in":dbl[], "X data in":dbl[]}[], "error out"=w833:errorcluster)  [unwired: 1 in]
            n239 = call "4155C Split array.vi"("Number of VAR2 steps"=w848, "Y2 data in"=w845, "X data in"=w854, "Y1 data in"=w847, "Y3 data in"=w843, "error in (no error)"=w833) -> ("Array of clusters"=w890:cluster{"Y data in":dbl[], "X data in":dbl[]}[], "error out"=w832:errorcluster)  [unwired: 1 in]
            n240 = call "4155C Config Chart Colours.vi"("Numeric"=w848, "XY Graph 2"=w883) -> ()  [unwired: 6 in]
            n241 = call "4155C Config Chart Colours.vi"("Numeric"=w848, "XY Graph 2"=w882) -> ()  [unwired: 6 in]
            n242 = call "4155C Config Chart Colours.vi"("Numeric"=w848, "XY Graph 2"=w851) -> ()  [unwired: 6 in]
            n243 = call "4155C Config Chart Colours.vi"("Numeric"=w848, "XY Graph 2"=w850) -> ()  [unwired: 6 in]
            n244 = call "4155C Config Chart Colours.vi"("Numeric"=w848, "XY Graph 2"=w892) -> ()  [unwired: 6 in]
            n245 = local write "Imax vs time"(w891) -> ()
            n246 = local write "Imin vs time"(w890) -> ()
            n247 = local write "Ion vs time"(w852) -> ()
            n248 = local write "Ioff vs time"(w853) -> ()
          }
        }
        n249 = call "4155C Config Chart Colours.vi"("Numeric"=w702, "XY Graph 2"=w743) -> ()  [unwired: 6 in]
        n250 = call "4155C Split array.vi"("Number of VAR2 steps"=w702, "Y2 data in"=w701, "X data in"=w745, "Y1 data in"=w701, "Y3 data in"=w703, "error in (no error)"=w705) -> ("Array of clusters"=w746:cluster{"Y data in":dbl[], "X data in":dbl[]}[], "error out"=w744:errorcluster)  [unwired: 1 in]
        n251 = local write "I vs Vg"(w746) -> ()
        n252 = Open/Create/Replace File(file path (use dialog)=w802, error in=w744, operation (0:open)=w758) -> (refnum out=w812:refnum<file>, error out=w813:errorcluster)  [unwired: 3 in, 1 out]
        n253 = call "4155C Make Big 2d array FPP.vi"("1D Var1"=w745, "1d ID"=w701, "1d Vp2"=w760, "1d IG"=w703, "1d Vp1"=w759, "VAR2 START"=w761, "Number of VAR2 steps"=w702, "VAR2 STEP"=w762, "VAR1 Name"="Vg", "Decimal places in header"=i8 1, "VAR2 Name"="Vd") -> ("Header array"=w808:string[], "Data array"=w809:dbl[][])  [unwired: 15 in]
        n254 = call "4155C Write array to file.vi"("Byte Stream File Refnum"=w812, "Header"=w808, "Data Array"=w809, "error in (no error)"=w813) -> ("dup refnum"=w810:refnum<file>, "error out"=w811:errorcluster)  [unwired: 1 in]
        n255 = Close File(refnum=w810, error in=w811) -> (error out=w797:errorcluster)  [unwired: 1 out]
      }
      frame "output" {
        n256 = local read "Transfer/Output - Drain"() -> (w906:u32)
        n257 = local read "Transfer/Output - Source/Common"() -> (w905:u32)
        n258 = local read "Transfer/Output - Gate"() -> (w907:u32)
        n259 = Delete From Array(array=w1005, index=0 ("Index")) -> (deleted portion=w1003:string, array with subset deleted=w1002:string[])  [unwired: 1 in]
        n260 = Bundle By Name(cluster=w918, "Emergency Stop"=w1014) -> (w968:T1)
        n261 = Number To Decimal String(number=w964) -> (decimal integer string=w963:string)  [unwired: 1 in]
        n262 = case shown="\"d\", Default" w1003 {
          tunnel: [w1099 w1100] -> w1001
          frame "s" {
            w1099 = u16 0 items=["Single", "Double"] ("sweep mode")
          }
          frame "d", Default {
            w1100 = u16 1 items=["Single", "Double"] ("sweep mode")
          }
        }
        n263 = Fract/Exp String To Number(string=w1002) -> (number=w987:dbl[])  [unwired: 3 in, 1 out]
        n264 = Concatenate Strings(w1012, "-output-" ("Substring"), w963, w961, ".txt" ("Suffix (transfer)")) -> (w1013:string)
        n265 = VISA Write(VISA resource name=w983, write buffer=":PAGE:CHAN:MODE SWE;" ("write buffer (\"\")"), error in (no error)=w982) -> (VISA resource name out=w980:refnum<visa-resource-name>, error out=w981:errorcluster)  [unwired: 1 out]
        n266 = String To Path(string=w1013) -> (path=w1011:path)
        n267 = Index Array(array=w987, index #1=0 ("Index")) -> (element #1=w1000:dbl, element #2=w999:dbl, element #3=w998:dbl)  [unwired: 2 in]
        n268 = Delete From Array(array=w987, length=3 ("Length"), index=0 ("Index")) -> (array with subset deleted=w985:dbl[])  [unwired: 1 out]
        n269 = local read "Plot output curve extrema vs time"() -> (w915:bool)
        n270 = local read "Transfer/Output - Probe 4"() -> (w908:u32)
        n271 = Bundle By Name(cluster=w992, "Gate Start"=w1000, "Gate Stop"=w999, "Gate Step (linear only)"=w998, "Gate Compliance"=w1009, "Range mode"=w976, "Range"=w975) -> (w977:T6)
        n272 = case shown="True" w915 {
          tunnel: w960 -> [w1016 w1019]
          tunnel: w957 -> [_ w1018]
          tunnel: [w1016 w1017] -> w934
          frame False {
          }
          frame True {
            n273 = Build Array (concatenate)(w1019, w1018) -> (w1017:i32[])
          }
        }
        n274 = Index Array(array=w985, index #1=0 ("Index")) -> (element #1=w995:dbl, element #2=w994:dbl, element #3=w993:dbl)  [unwired: 2 in]
        n275 = call <vilib>:"compatOverwrite.vi"("overwrite (F)"=TRUE) -> ("overwrite?"=w967:T8)
        n276 = Bundle By Name(cluster=w991, "Drain Start"=w995, "Drain Stop"=w994, "Drain Step"=w993, "Drain Compliance"=w1010, "Range mode"=w974, "Range"=w973) -> (w978:T7)
        n277 = call "4155C Output v3.0.vi"("VISA resource name in"=w980, "Source/Common"=w905, 2:"Gate"=w977, 3:"Drain"=w978, 4:"Drain"=w906, "Timings"=w1008, "error in (no error)"=w981, 7:"Probe 4"=w914, 8:"Gate"=w907, 9:"Probe 4"=w908, "sweep mode"=w1001, "Panel controls"=w968, "Standby"=w909) -> ("VD"=w966:dbl[], "Outparams"=w972:T9, "VISA Resource Name out"=w1007:refnum<visa-resource-name>, "IS"=w944:dbl[], "ID"=w945:dbl[], "IG"=w943:dbl[], "error out"=w958:errorcluster, "Probe 4"=w969:dbl[])  [unwired: 7 in]
        n278 = Unbundle By Name(w972) -> ("V2 Step"=w971:dbl, "V2 Start"=w970:dbl, "Number of points"=w932:i32)
        n279 = call "4155C Split array.vi"("Number of VAR2 steps"=w932, "Y2 data in"=w945, "X data in"=w966, "Y1 data in"=w944, "Y3 data in"=w943, "error in (no error)"=w958) -> ("Array of clusters"=w959:cluster{"Y data in":dbl[], "X data in":dbl[]}[], "error out"=w920:errorcluster)  [unwired: 1 in]
        n280 = case shown="True" "Plot output curve extrema vs time" {
          tunnel: w965 -> [w1028 w1098]
          tunnel: w956 -> [w1029 w1093]
          tunnel: w947 -> [w1023 w1089]
          tunnel: w946 -> [w1022 w1088]
          tunnel: w945 -> [_ w1085]
          tunnel: w944 -> [_ w1083]
          tunnel: w943 -> [_ w1082]
          tunnel: w942 -> [w1030 w1078]
          tunnel: w941 -> [w1031 w1077]
          tunnel: w940 -> [w1026 w1074]
          tunnel: w939 -> [w1027 w1073]
          tunnel: w938 -> [w1024 w1070]
          tunnel: w937 -> [w1025 w1069]
          tunnel: w936 -> [w1020 w1066]
          tunnel: w935 -> [w1021 w1065]
          tunnel: w934 -> [_ w1058]
          tunnel: [w1026 w1053] -> w933
          tunnel: w932 -> [_ w1052]
          tunnel: [w1027 w1051] -> w931
          tunnel: [w1028 w1050] -> w930
          tunnel: [w1029 w1049] -> w929
          tunnel: [w1030 w1048] -> w928
          tunnel: [w1031 w1047] -> w927
          tunnel: [w1020 w1046] -> w926
          tunnel: [w1021 w1045] -> w925
          tunnel: [w1022 w1044] -> w924
          tunnel: [w1023 w1043] -> w923
          tunnel: [w1024 w1042] -> w922
          tunnel: [w1025 w1041] -> w921
          tunnel: w920 -> [w1032 w1040]
          tunnel: [w1032 w1036] -> w919
          frame False {
          }
          frame True {
            # "Adjusts graph colors."
            # "Adjusts graph colors."
            # "Ion will be the middle element of the array. The calculation of the index is done only once, since Is, Id, and Ig have the same dimensions."
            # "abs(Ig)"
            # "abs(Is)"
            # "Y1: Is\nY2: Id\nY3: Ig"
            # "abs(Id)"
            # "Adjusts graph colors."
            # "Adjusts graph colors."
            # "Adjusts graph colors."
            n281 = Absolute Value(x=w1083) -> (abs(x)=w1068:dbl[])
            n282 = Absolute Value(x=w1085) -> (abs(x)=w1084:dbl[])
            n283 = Absolute Value(x=w1082) -> (abs(x)=w1071:dbl[])
            n284 = Array Size(array=w1084) -> (size(s)=w1092:i32)
            n285 = Divide(x=w1092, y=2) -> (x/y=w1035:dbl)
            n286 = Subtract(x=w1035, y=1) -> (x-y=w1034:dbl)
            n287 = Array Max & Min(array=w1068) -> (max value=w1075:dbl, min value=w1076:dbl)  [unwired: 2 out]
            n288 = Array Max & Min(array=w1084) -> (max value=w1097:dbl, min value=w1081:dbl)  [unwired: 2 out]
            n289 = Array Max & Min(array=w1071) -> (max value=w1080:dbl, min value=w1079:dbl)  [unwired: 2 out]
            n290 = Index Array(array=w1068, index=w1034) -> (element=w1059:dbl)
            n291 = Index Array(array=w1068, index=0) -> (element=w1060:dbl)
            n292 = Index Array(array=w1084, index=w1034) -> (element=w1061:dbl)
            n293 = Index Array(array=w1084, index=0) -> (element=w1062:dbl)
            n294 = Index Array(array=w1071, index=w1034) -> (element=w1064:dbl)
            n295 = Index Array(array=w1071, index=0) -> (element=w1063:dbl)
            n296 = local write "Ig max"(w1080) -> ()
            n297 = local write "Ig min"(w1079) -> ()
            n298 = local write "Is max"(w1075) -> ()
            n299 = local write "Is min"(w1076) -> ()
            n300 = local write "Id max"(w1097) -> ()
            n301 = local write "Id min"(w1081) -> ()
            n302 = Build Array (concatenate)(w1074, w1075) -> (w1053:dbl[])
            n303 = Build Array (concatenate)(w1073, w1076) -> (w1051:dbl[])
            n304 = local write "Is off"(w1060) -> ()
            n305 = local write "Is on"(w1059) -> ()
            n306 = Build Array (concatenate)(w1098, w1097) -> (w1050:dbl[])
            n307 = Build Array (concatenate)(w1093, w1081) -> (w1049:dbl[])
            n308 = Build Array (concatenate)(w1078, w1080) -> (w1048:dbl[])
            n309 = Build Array (concatenate)(w1077, w1079) -> (w1047:dbl[])
            n310 = Build Array (concatenate)(w1066, w1059) -> (w1046:dbl[])
            n311 = Build Array (concatenate)(w1065, w1060) -> (w1045:dbl[])
            n312 = Build Array (concatenate)(w1088, w1061) -> (w1044:dbl[])
            n313 = Build Array (concatenate)(w1089, w1062) -> (w1043:dbl[])
            n314 = Build Array (concatenate)(w1070, w1064) -> (w1042:dbl[])
            n315 = Build Array (concatenate)(w1069, w1063) -> (w1041:dbl[])
            n316 = local write "Ig off"(w1063) -> ()
            n317 = local write "Ig on"(w1064) -> ()
            n318 = local write "Id off"(w1062) -> ()
            n319 = local write "Id on"(w1061) -> ()
            n320 = control-ref of="Imax vs time"() -> (w1087:refnum<vi>)
            n321 = control-ref of="Imin vs time"() -> (w1086:refnum<vi>)
            n322 = control-ref of="Ion vs time"() -> (w1055:refnum<vi>)
            n323 = control-ref of="Ioff vs time"() -> (w1054:refnum<vi>)
            n324 = control-ref of="I vs Vg"() -> (w1096:refnum<vi>)
            n325 = call "4155C Split array.vi"("Number of VAR2 steps"=w1052, "Y2 data in"=w1044, "X data in"=w1058, "Y1 data in"=w1046, "Y3 data in"=w1042, "error in (no error)"=w1040) -> ("Array of clusters"=w1056:cluster{"Y data in":dbl[], "X data in":dbl[]}[], "error out"=w1039:errorcluster)  [unwired: 1 in]
            n326 = call "4155C Split array.vi"("Number of VAR2 steps"=w1052, "Y2 data in"=w1043, "X data in"=w1058, "Y1 data in"=w1045, "Y3 data in"=w1041, "error in (no error)"=w1039) -> ("Array of clusters"=w1057:cluster{"Y data in":dbl[], "X data in":dbl[]}[], "error out"=w1038:errorcluster)  [unwired: 1 in]
            n327 = call "4155C Split array.vi"("Number of VAR2 steps"=w1052, "Y2 data in"=w1050, "X data in"=w1058, "Y1 data in"=w1053, "Y3 data in"=w1048, "error in (no error)"=w1038) -> ("Array of clusters"=w1095:cluster{"Y data in":dbl[], "X data in":dbl[]}[], "error out"=w1037:errorcluster)  [unwired: 1 in]
            n328 = call "4155C Split array.vi"("Number of VAR2 steps"=w1052, "Y2 data in"=w1049, "X data in"=w1058, "Y1 data in"=w1051, "Y3 data in"=w1047, "error in (no error)"=w1037) -> ("Array of clusters"=w1094:cluster{"Y data in":dbl[], "X data in":dbl[]}[], "error out"=w1036:errorcluster)  [unwired: 1 in]
            n329 = call "4155C Config Chart Colours.vi"("Numeric"=w1052, "XY Graph 2"=w1087) -> ()  [unwired: 6 in]
            n330 = call "4155C Config Chart Colours.vi"("Numeric"=w1052, "XY Graph 2"=w1086) -> ()  [unwired: 6 in]
            n331 = call "4155C Config Chart Colours.vi"("Numeric"=w1052, "XY Graph 2"=w1055) -> ()  [unwired: 6 in]
            n332 = call "4155C Config Chart Colours.vi"("Numeric"=w1052, "XY Graph 2"=w1054) -> ()  [unwired: 6 in]
            n333 = call "4155C Config Chart Colours.vi"("Numeric"=w1052, "XY Graph 2"=w1096) -> ()  [unwired: 6 in]
            n334 = local write "Imax vs time"(w1095) -> ()
            n335 = local write "Imin vs time"(w1094) -> ()
            n336 = local write "Ion vs time"(w1056) -> ()
            n337 = local write "Ioff vs time"(w1057) -> ()
          }
        }
        n338 = local write "I vs Vd"(w959) -> ()
        n339 = Open/Create/Replace File(file path (use dialog)=w1011, error in=w919, operation (0:open)=w967) -> (refnum out=w954:refnum<file>, error out=w952:errorcluster)  [unwired: 3 in, 1 out]
        n340 = call "4155C Make Big 2d array.vi"("1D Var1"=w966, "1d IS"=w944, "1d ID"=w945, "1d IG"=w943, "1d SMU4"=w969, "SMU4"=w914, "VAR2 START"=w970, "Number of VAR2 steps"=w932, "VAR2 STEP"=w971, "VAR1 Name"="Vd", "Decimal places in header"=i8 1, "VAR2 Name"="Vg") -> ("Header array"=w955:string[], "Data array"=w953:dbl[][])  [unwired: 14 in]
        n341 = call "4155C Write array to file.vi"("Byte Stream File Refnum"=w954, "Header"=w955, "Data Array"=w953, "error in (no error)"=w952) -> ("dup refnum"=w951:refnum<file>, "error out"=w950:errorcluster)  [unwired: 1 in]
        n342 = Close File(refnum=w951, error in=w950) -> (error out=w1006:errorcluster)  [unwired: 1 out]
      }
      frame "output-fpp" {
        # "Y1 = Y2 = ID\nY3 = IG"
        # "Adjusts graph colors."
        # "Adjusts graph colors."
        # "Y1 = Vp2\nY2 = Y3 = Vp1"
        n343 = local read "Plot output curve extrema vs time"() -> (w1140:bool)
        n344 = Number To Decimal String(number=w1162) -> (decimal integer string=w1206:string)  [unwired: 1 in]
        n345 = Bundle By Name(cluster=w1184, "Emergency Stop"=w1209) -> (w1219:T1)
        n346 = local read "Plot output curve extrema vs time"() -> (w1142:bool)
        n347 = local read "FPP - Source"() -> (w1155:u32)
        n348 = Delete From Array(array=w1141, index=0 ("Index")) -> (deleted portion=w1197:string, array with subset deleted=w1196:string[])  [unwired: 1 in]
        n349 = local read "FPP - Drain"() -> (w1156:u32)
        n350 = local read "FPP - Gate"() -> (w1157:u32)
        n351 = VISA Write(VISA resource name=w1175, write buffer=":PAGE:CHAN:MODE SWE;" ("write buffer (\"\")"), error in (no error)=w1172) -> (VISA resource name out=w1174:refnum<visa-resource-name>, error out=w1173:errorcluster)  [unwired: 1 out]
        n352 = Concatenate Strings(w1205, "-outputfpp-" ("Substring"), w1206, w1161, ".txt" ("Substring")) -> (w1208:string)
        n353 = case shown="\"d\", Default" w1197 {
          tunnel: [w1303 w1304] -> w1195
          frame "s" {
            w1303 = u16 0 items=["Single", "Double"] ("sweep mode")
          }
          frame "d", Default {
            w1304 = u16 1 items=["Single", "Double"] ("sweep mode")
          }
        }
        n354 = Fract/Exp String To Number(string=w1196) -> (number=w1178:dbl[])  [unwired: 3 in, 1 out]
        n355 = String To Path(string=w1208) -> (path=w1204:path)
        n356 = Index Array(array=w1178, index #1=0 ("Index")) -> (element #1=w1194:dbl, element #2=w1193:dbl, element #3=w1192:dbl)  [unwired: 2 in]
        n357 = Delete From Array(array=w1178, length=3 ("Length"), index=0 ("Index")) -> (array with subset deleted=w1177:dbl[])  [unwired: 1 out]
        n358 = local read "FPP - Probe 1"() -> (w1153:u32)
        n359 = local read "FPP - Probe 2"() -> (w1154:u32)
        n360 = case shown="True" w1142 {
          tunnel: w1143 -> [w1299 w1302]
          tunnel: w1144 -> [_ w1301]
          tunnel: [w1299 w1300] -> w1103
          frame False {
          }
          frame True {
            n361 = Build Array (concatenate)(w1302, w1301) -> (w1300:i32[])
          }
        }
        n362 = Bundle By Name(cluster=w1186, "Gate Start"=w1194, "Gate Stop"=w1193, "Gate Step (linear only)"=w1192, "Gate Compliance"=w1202, "Range mode"=w1170, "Range"=w1169) -> (w1218:T6)
        n363 = Index Array(array=w1177, index #1=0 ("Index")) -> (element #1=w1189:dbl, element #2=w1188:dbl, element #3=w1187:dbl)  [unwired: 2 in]
        n364 = call <vilib>:"compatOverwrite.vi"("overwrite (F)"=TRUE) -> ("overwrite?"=w1164:T8)
        n365 = Bundle By Name(cluster=w1185, "Drain Start"=w1189, "Drain Stop"=w1188, "Drain Step"=w1187, "Drain Compliance"=w1203, "Range mode"=w1168, "Range"=w1171) -> (w1217:T7)
        n366 = call "4155C Output-FPP v3.0.vi"("VISA resource name in"=w1174, "FPP - Source"=w1155, "Gate"=w1218, "Drain"=w1217, "FPP - Drain"=w1156, "Timings"=w1201, "error in (no error)"=w1173, "FPP - Gate"=w1157, "FPP - Probe 1"=w1153, "sweep mode"=w1195, "FPP - Probe 2"=w1154, "Panel controls"=w1219) -> ("VD"=w1149:dbl[], "Outparams"=w1166:T9, "VISA Resource Name out"=w1200:refnum<visa-resource-name>, "Vprobe2"=w1148:dbl[], "ID"=w1102:dbl[], "IG"=w1101:dbl[], "Vprobe1"=w1147:dbl[], "error out"=w1115:errorcluster)  [unwired: 8 in]
        n367 = Unbundle By Name(w1166) -> ("V2 Step"=w1167:dbl, "V2 Start"=w1165:dbl, "Number of points"=w1104:i32)
        n368 = case shown="True" w1140 {
          tunnel: w1136 -> [w1228 w1298]
          tunnel: w1137 -> [w1229 w1293]
          tunnel: w1131 -> [w1223 w1289]
          tunnel: w1130 -> [w1222 w1288]
          tunnel: w1102 -> [_ w1285]
          tunnel: w1102 -> [_ w1283]
          tunnel: w1101 -> [_ w1282]
          tunnel: w1138 -> [w1230 w1278]
          tunnel: w1139 -> [w1231 w1277]
          tunnel: w1134 -> [w1226 w1274]
          tunnel: w1135 -> [w1227 w1273]
          tunnel: w1132 -> [w1224 w1270]
          tunnel: w1133 -> [w1225 w1269]
          tunnel: w1128 -> [w1220 w1266]
          tunnel: w1129 -> [w1221 w1265]
          tunnel: w1103 -> [_ w1258]
          tunnel: [w1226 w1253] -> w1122
          tunnel: w1104 -> [_ w1252]
          tunnel: [w1227 w1251] -> w1123
          tunnel: [w1228 w1250] -> w1124
          tunnel: [w1229 w1249] -> w1125
          tunnel: [w1230 w1248] -> w1126
          tunnel: [w1231 w1247] -> w1127
          tunnel: [w1220 w1246] -> w1116
          tunnel: [w1221 w1245] -> w1117
          tunnel: [w1222 w1244] -> w1118
          tunnel: [w1223 w1243] -> w1119
          tunnel: [w1224 w1242] -> w1120
          tunnel: [w1225 w1241] -> w1121
          tunnel: w1115 -> [w1232 w1240]
          tunnel: [w1232 w1236] -> w1114
          frame False {
          }
          frame True {
            # "Y1 = Y2 = ID\nY3 = IG"
            # "Adjusts graph colors."
            # "Adjusts graph colors."
            # "Ion will be the middle element of the array. The calculation of the index is done only once, since Is, Id, and Ig have the same dimensions."
            # "abs(Ig)"
            # "abs(Is)"
            # "abs(Id)"
            # "Adjusts graph colors."
            # "Adjusts graph colors."
            # "Adjusts graph colors."
            n369 = Absolute Value(x=w1283) -> (abs(x)=w1268:dbl[])
            n370 = Absolute Value(x=w1285) -> (abs(x)=w1284:dbl[])
            n371 = Absolute Value(x=w1282) -> (abs(x)=w1271:dbl[])
            n372 = Array Size(array=w1284) -> (size(s)=w1292:i32)
            n373 = Divide(x=w1292, y=2) -> (x/y=w1235:dbl)
            n374 = Subtract(x=w1235, y=1) -> (x-y=w1234:dbl)
            n375 = Array Max & Min(array=w1268) -> (max value=w1275:dbl, min value=w1276:dbl)  [unwired: 2 out]
            n376 = Array Max & Min(array=w1284) -> (max value=w1297:dbl, min value=w1281:dbl)  [unwired: 2 out]
            n377 = Array Max & Min(array=w1271) -> (max value=w1280:dbl, min value=w1279:dbl)  [unwired: 2 out]
            n378 = Index Array(array=w1268, index=w1234) -> (element=w1259:dbl)
            n379 = Index Array(array=w1268, index=0) -> (element=w1260:dbl)
            n380 = Index Array(array=w1284, index=w1234) -> (element=w1261:dbl)
            n381 = Index Array(array=w1284, index=0) -> (element=w1262:dbl)
            n382 = Index Array(array=w1271, index=w1234) -> (element=w1264:dbl)
            n383 = Index Array(array=w1271, index=0) -> (element=w1263:dbl)
            n384 = local write "Ig max"(w1280) -> ()
            n385 = local write "Ig min"(w1279) -> ()
            n386 = local write "Is max"(w1275) -> ()
            n387 = local write "Is min"(w1276) -> ()
            n388 = local write "Id max"(w1297) -> ()
            n389 = local write "Id min"(w1281) -> ()
            n390 = Build Array (concatenate)(w1274, w1275) -> (w1253:dbl[])
            n391 = Build Array (concatenate)(w1273, w1276) -> (w1251:dbl[])
            n392 = local write "Is off"(w1260) -> ()
            n393 = local write "Is on"(w1259) -> ()
            n394 = Build Array (concatenate)(w1298, w1297) -> (w1250:dbl[])
            n395 = Build Array (concatenate)(w1293, w1281) -> (w1249:dbl[])
            n396 = Build Array (concatenate)(w1278, w1280) -> (w1248:dbl[])
            n397 = Build Array (concatenate)(w1277, w1279) -> (w1247:dbl[])
            n398 = Build Array (concatenate)(w1266, w1259) -> (w1246:dbl[])
            n399 = Build Array (concatenate)(w1265, w1260) -> (w1245:dbl[])
            n400 = Build Array (concatenate)(w1288, w1261) -> (w1244:dbl[])
            n401 = Build Array (concatenate)(w1289, w1262) -> (w1243:dbl[])
            n402 = Build Array (concatenate)(w1270, w1264) -> (w1242:dbl[])
            n403 = Build Array (concatenate)(w1269, w1263) -> (w1241:dbl[])
            n404 = local write "Ig off"(w1263) -> ()
            n405 = local write "Ig on"(w1264) -> ()
            n406 = local write "Id off"(w1262) -> ()
            n407 = local write "Id on"(w1261) -> ()
            n408 = control-ref of="Imax vs time"() -> (w1287:refnum<vi>)
            n409 = control-ref of="Imin vs time"() -> (w1286:refnum<vi>)
            n410 = control-ref of="Ion vs time"() -> (w1255:refnum<vi>)
            n411 = control-ref of="Ioff vs time"() -> (w1254:refnum<vi>)
            n412 = control-ref of="I vs Vg"() -> (w1296:refnum<vi>)
            n413 = call "4155C Split array.vi"("Number of VAR2 steps"=w1252, "Y2 data in"=w1244, "X data in"=w1258, "Y1 data in"=w1246, "Y3 data in"=w1242, "error in (no error)"=w1240) -> ("Array of clusters"=w1256:cluster{"Y data in":dbl[], "X data in":dbl[]}[], "error out"=w1239:errorcluster)  [unwired: 1 in]
            n414 = call "4155C Split array.vi"("Number of VAR2 steps"=w1252, "Y2 data in"=w1243, "X data in"=w1258, "Y1 data in"=w1245, "Y3 data in"=w1241, "error in (no error)"=w1239) -> ("Array of clusters"=w1257:cluster{"Y data in":dbl[], "X data in":dbl[]}[], "error out"=w1238:errorcluster)  [unwired: 1 in]
            n415 = call "4155C Split array.vi"("Number of VAR2 steps"=w1252, "Y2 data in"=w1250, "X data in"=w1258, "Y1 data in"=w1253, "Y3 data in"=w1248, "error in (no error)"=w1238) -> ("Array of clusters"=w1295:cluster{"Y data in":dbl[], "X data in":dbl[]}[], "error out"=w1237:errorcluster)  [unwired: 1 in]
            n416 = call "4155C Split array.vi"("Number of VAR2 steps"=w1252, "Y2 data in"=w1249, "X data in"=w1258, "Y1 data in"=w1251, "Y3 data in"=w1247, "error in (no error)"=w1237) -> ("Array of clusters"=w1294:cluster{"Y data in":dbl[], "X data in":dbl[]}[], "error out"=w1236:errorcluster)  [unwired: 1 in]
            n417 = call "4155C Config Chart Colours.vi"("Numeric"=w1252, "XY Graph 2"=w1287) -> ()  [unwired: 6 in]
            n418 = call "4155C Config Chart Colours.vi"("Numeric"=w1252, "XY Graph 2"=w1286) -> ()  [unwired: 6 in]
            n419 = call "4155C Config Chart Colours.vi"("Numeric"=w1252, "XY Graph 2"=w1255) -> ()  [unwired: 6 in]
            n420 = call "4155C Config Chart Colours.vi"("Numeric"=w1252, "XY Graph 2"=w1254) -> ()  [unwired: 6 in]
            n421 = call "4155C Config Chart Colours.vi"("Numeric"=w1252, "XY Graph 2"=w1296) -> ()  [unwired: 6 in]
            n422 = local write "Imax vs time"(w1295) -> ()
            n423 = local write "Imin vs time"(w1294) -> ()
            n424 = local write "Ion vs time"(w1256) -> ()
            n425 = local write "Ioff vs time"(w1257) -> ()
          }
        }
        n426 = call "4155C Split array.vi"("Number of VAR2 steps"=w1104, "Y2 data in"=w1147, "X data in"=w1149, "Y1 data in"=w1148, "Y3 data in"=w1147, "error in (no error)"=w1114) -> ("Array of clusters"=w1150:cluster{"Y data in":dbl[], "X data in":dbl[]}[], "error out"=w1113:errorcluster)  [unwired: 1 in]
        n427 = call "4155C Split array.vi"("Number of VAR2 steps"=w1104, "Y2 data in"=w1102, "X data in"=w1149, "Y1 data in"=w1102, "Y3 data in"=w1101, "error in (no error)"=w1113) -> ("Array of clusters"=w1152:cluster{"Y data in":dbl[], "X data in":dbl[]}[], "error out"=w1151:errorcluster)  [unwired: 1 in]
        n428 = local write "I vs Vd"(w1152) -> ()
        n429 = local write "Vp vs Vg (FPP)"(w1150) -> ()
        n430 = Open/Create/Replace File(file path (use dialog)=w1204, error in=w1151, operation (0:open)=w1164) -> (refnum out=w1214:refnum<file>, error out=w1215:errorcluster)  [unwired: 3 in, 1 out]
        n431 = call "4155C Make Big 2d array FPP.vi"("1D Var1"=w1149, "1d ID"=w1102, "1d Vp2"=w1148, "1d IG"=w1101, "1d Vp1"=w1147, "VAR2 START"=w1165, "Number of VAR2 steps"=w1104, "VAR2 STEP"=w1167, "VAR1 Name"="Vd", "Decimal places in header"=i8 1, "VAR2 Name"="Vg") -> ("Header array"=w1210:string[], "Data array"=w1211:dbl[][])  [unwired: 15 in]
        n432 = control-ref of="I vs Vd"() -> (w1146:refnum<vi>)
        n433 = control-ref of="Vp vs Vg (FPP)"() -> (w1145:refnum<vi>)
        n434 = call "4155C Write array to file.vi"("Byte Stream File Refnum"=w1214, "Header"=w1210, "Data Array"=w1211, "error in (no error)"=w1215) -> ("dup refnum"=w1212:refnum<file>, "error out"=w1213:errorcluster)  [unwired: 1 in]
        n435 = Close File(refnum=w1212, error in=w1213) -> (error out=w1199:errorcluster)  [unwired: 1 out]
        n436 = call "4155C Config Chart Colours.vi"("Numeric"=w1104, "XY Graph 2"=w1146) -> ()  [unwired: 6 in]
        n437 = call "4155C Config Chart Colours.vi"("Numeric"=w1104, "XY Graph 2"=w1145) -> ()  [unwired: 6 in]
      }
      frame "itime" {
        n438 = Delete From Array(array=w1316, index=1) -> (deleted portion=w1315:string)  [unwired: 1 in, 1 out]
        n439 = Delete From Array(array=w1316, index=0 ("Index")) -> (deleted portion=w1344:string)  [unwired: 1 in, 1 out]
        n440 = Fract/Exp String To Number(string=w1315) -> (number=w1314:dbl)  [unwired: 3 in, 1 out]
        n441 = case shown="\"l\"" w1344 {
          tunnel: w1343 -> [w1349 w1351 w1355]
          tunnel: [w1348 w1350 w1354] -> w1336
          tunnel: w1314 -> [w1346 _ w1353]
          frame "s" {
            w1347 = u32 0 items=["short  ", "medium  ", "long  "] ("integration time 2")
            n442 = Bundle By Name(cluster=w1349, "integration time"=w1347, "Short/Long integration time"=w1346) -> (w1348:T4)
          }
          frame "m", Default {
            w1352 = u32 1 items=["short  ", "medium  ", "long  "] ("integration time 2")
            n443 = Bundle By Name(cluster=w1351, "integration time"=w1352) -> (w1350:T4)
          }
          frame "l" {
            w1356 = u32 2 items=["short  ", "medium  ", "long  "] ("integration time 2")
            n444 = Bundle By Name(cluster=w1355, "integration time"=w1356, "Short/Long integration time"=w1353) -> (w1354:T4)
          }
        }
      }
      frame "pulsed" {
        n445 = Delete From Array(array=w1393, index=0 ("Index")) -> (deleted portion=w1394:string, array with subset deleted=w1381:string[])  [unwired: 1 in]
        n446 = case shown="\"on\", Default" w1394 {
          tunnel: w1392 -> [w1404 w1407]
          tunnel: [w1403 w1406] -> w1385
          tunnel: w1381 -> [w1401 _]
          frame "on", Default {
            w1402 = u16 1 items=["Continuous", "Pulsed"] ("sweep method")
            n447 = Fract/Exp String To Number(string=w1401) -> (number=w1399:dbl[])  [unwired: 3 in, 1 out]
            n448 = Index Array(array=w1399, index #1=0 ("Index")) -> (element #1=w1398:dbl, element #2=w1397:dbl, element #3=w1396:dbl)  [unwired: 2 in]
            n449 = Bundle By Name(cluster=w1404, "sweep method"=w1402, "Pulse period"=w1398, "Base voltage"=w1397, "Pulse width"=w1396) -> (w1403:T4)
          }
          frame "off" {
            w1405 = u16 0 items=["Continuous", "Pulsed"] ("sweep method")
            n450 = Bundle By Name(cluster=w1407, "sweep method"=w1405) -> (w1406:T4)
          }
        }
      }
      frame "gaterangemode" {
        n451 = Delete From Array(array=w1442, index=0 ("Index")) -> (deleted portion=w1443:string)  [unwired: 1 in, 1 out]
        n452 = case shown="\"f\"" w1443 {
          tunnel: [w1445 w1446 w1447] -> w1432
          frame "a", Default {
            w1445 = u16 0 items=["Auto", "Limited", "Fixed"] ("Gate Range\nmode 2")
          }
          frame "f" {
            w1446 = u16 2 items=["Auto", "Limited", "Fixed"] ("Gate Range\nmode 2")
          }
          frame "l" {
            w1447 = u16 1 items=["Auto", "Limited", "Fixed"] ("Gate Range\nmode 2")
          }
        }
      }
      frame "gaterange" {
        (unwired) u8 11 items=["10fA  ", "100fA  ", "1nA  ", "10nA", "100nA", "1uA", "10uA", "100uA", "1mA", "10mA", "100mA", "1A"] ("Gate Range 2")
        n453 = Delete From Array(array=w1489, index=0 ("Index")) -> (deleted portion=w1479:string)  [unwired: 1 in, 1 out]
        n454 = Scan Value(string=w1479, format string="") -> (value=w1477:dbl)  [unwired: 1 in, 1 out]
        n455 = Logarithm Base 10(1:w1477) -> (0:w1476:dbl)
        n456 = Round To Nearest(number=w1476) -> (nearest integer value=w1475:dbl)
        n457 = Add(x=w1475, y=11.0) -> (x+y=w1473:dbl)
        n458 = To Unsigned Byte Integer(number=w1473) -> (unsigned 8bit integer=w1472:u8)
      }
      frame "drainrange" {
        (unwired) u8 11 items=["10fA  ", "100fA  ", "1nA  ", "10nA", "100nA", "1uA", "10uA", "100uA", "1mA", "10mA", "100mA", "1A"] ("Gate Range 2")
        n459 = Delete From Array(array=w1532, index=0 ("Index")) -> (deleted portion=w1523:string)  [unwired: 1 in, 1 out]
        n460 = Scan Value(string=w1523, format string="") -> (value=w1521:dbl)  [unwired: 1 in, 1 out]
        n461 = Logarithm Base 10(1:w1521) -> (0:w1520:dbl)
        n462 = Round To Nearest(number=w1520) -> (nearest integer value=w1519:dbl)
        n463 = Add(x=w1519, y=11.0) -> (x+y=w1517:dbl)
        n464 = To Unsigned Byte Integer(number=w1517) -> (unsigned 8bit integer=w1516:u8)
      }
      frame "drainrangemode" {
        n465 = Delete From Array(array=w1568, index=0 ("Index")) -> (deleted portion=w1569:string)  [unwired: 1 in, 1 out]
        n466 = case shown="\"f\"" w1569 {
          tunnel: [w1571 w1572 w1573] -> w1558
          frame "a", Default {
            w1571 = u16 0 items=["Auto", "Limited", "Fixed"] ("Gate Range\nmode 2")
          }
          frame "f" {
            w1572 = u16 2 items=["Auto", "Limited", "Fixed"] ("Gate Range\nmode 2")
          }
          frame "l" {
            w1573 = u16 1 items=["Auto", "Limited", "Fixed"] ("Gate Range\nmode 2")
          }
        }
      }
      frame "Error", Default {
      }
      frame "logfile" {
        n467 = Number To Decimal String(number=w1632) -> (decimal integer string=w1667:string)  [unwired: 1 in]
        n468 = Concatenate Strings(w1666, "logfile" ("Substring"), w1667, w1630, ".txt" ("Substring")) -> (w1664:string)
        n469 = String To Path(string=w1664) -> (path=w1637:path)
        n470 = Unbundle(w1663) -> ("integration time"=w1662:u32, "Short/Long integration time"=w1661:dbl, "hold time (sec)"=w1660:dbl, "delay time (sec)"=w1659:dbl, "Step Time (0 disables)"=w1658:dbl, "sweep method"=w1657:u16, "Pulse period"=w1656:dbl, "Base voltage"=w1655:dbl, "Pulse width"=w1654:dbl)
        n471 = Build Array(w1662, w1661, w1660, w1659, w1658, w1657, w1656, w1655, w1654, w1648, w1649, w1650, w1651, w1652, w1653) -> (w1641:dbl[])
        n472 = Insert Into Array(array=dbl[][] [] ("Input Array"), new element=w1641) -> (w1640:dbl[][])  [unwired: 2 in]
        n473 = call <vilib>:"compatOverwrite.vi"("overwrite (F)"=TRUE) -> ("overwrite?"=w1635:T8)
        n474 = Open/Create/Replace File(file path (use dialog)=w1637, error in=w1639, operation (0:open)=w1635) -> (refnum out=w1645:refnum<file>, error out=w1644:errorcluster)  [unwired: 3 in, 1 out]
        n475 = call "4155C Write array to file.vi"("Byte Stream File Refnum"=w1645, "Header"=string[] ["Int Time", "Short/Long Itime", "Hold time", "Delay time", "Step time", "Sweep method", "Pulse period", "Base Voltage", "Pulse width", "Drain compliance", "Gate compliance", "Gate range mode", "Gate range", "S/D range mode", "S/D range"], "Data Array"=w1640, "error in (no error)"=w1644) -> ("dup refnum"=w1647:refnum<file>, "error out"=w1646:errorcluster)  [unwired: 1 in]
        n476 = Close File(refnum=w1647, error in=w1646) -> (error out=w1638:errorcluster)  [unwired: 1 out]
      }
      frame "sample" {
        w1695 = 1
        # "Add a time offset (elapsed time) to the time axis."
        # "Adjusts graph colors."
        n477 = Number To Decimal String(number=w1727) -> (decimal integer string=w1769:string)  [unwired: 1 in]
        n478 = Fract/Exp String To Number(string=w1766) -> (number=w1731:dbl[])  [unwired: 3 in, 1 out]
        n479 = local read "Sample - Probe 4"() -> (w1677:u32)
        n480 = Concatenate Strings(w1747, "-sample-" ("Substring"), w1769, w1725, ".txt" ("Substring")) -> (w1767:string)
        n481 = local read "Sample - Drain"() -> (w1678:u32)
        n482 = Index Array(array=w1731, index=0 ("Index")) -> (element=w1764:dbl)
        n483 = String To Path(string=w1767) -> (path=w1751:path)
        n484 = Index Array(array=w1731, index=2 ("Index")) -> (element=w1760:dbl)
        n485 = Index Array(array=w1731, index=3 ("Index")) -> (element=w1733:dbl)
        n486 = Index Array(array=w1731, index=4 ("Index")) -> (element=w1730:dbl)
        n487 = Index Array(array=w1731, index=1 ("Index")) -> (element=w1761:dbl)
        n488 = local read "Plot sample extrema vs time"() -> (w1698:bool)
        n489 = local read "Time Units"() -> (w1673:u16)
        n490 = local read "Sample - Gate"() -> (w1680:u32)
        n491 = local read "Sample - Source/Common"() -> (w1679:u32)
        n492 = call "4155C Config Sampling Measurements v3.0.vi"("VISA session"=w1772, "Num Points"=w1760, "Sample - Drain"=w1678, "Display on/off"=TRUE, "Gate Compliance"=w1748, "Sampling interval"=w1730, "Sample - Source/Common"=w1679, "Sample - Probe 4"=w1677, "Drain Compliance"=w1770, "Standby"=w1681, "error in (no error)"=w1771, "Timings"=w1739, "Sample - Gate"=w1680, "Sample time"=w1733) -> ("dup VISA resource name"=w1774:refnum<visa-resource-name>, "error out"=w1773:errorcluster)
        n493 = call "4155C Take Sample v3.0.vi"("VISA resource name in"=w1774, "Emergency Stop"=w1744, "Sample - Gate"=w1680, "Vg"=w1764, "Sample - Drain"=w1678, "Vd"=w1761, "error in (no error)"=w1773) -> ("Time"=w1675:dbl[], "VISA Resource Name out"=w1741:refnum<visa-resource-name>, "Ig"=w1691:dbl[], "Id"=w1692:dbl[], "Is"=w1693:dbl[], "error out"=w1696:errorcluster)  [unwired: 3 in]
        n494 = case shown="0, Default" w1673 {
          tunnel: [w1777 w1778 w1781] -> w1676
          tunnel: w1675 -> [w1776 w1778 w1780]
          frame 2 {
            n495 = Divide(x=w1776, y=3600.0) -> (x/y=w1777:dbl[])
          }
          frame 0, Default {
          }
          frame 1 {
            n496 = Divide(x=w1780, y=60.0) -> (x/y=w1781:dbl[])
          }
        }
        n497 = Insert Into Array(array=w1689, new element=w1692) -> (w1683:dbl[])  [unwired: 1 in]
        n498 = Add(x=w1676, y=w1674) -> (x+y=w1694:dbl[])
        n499 = Insert Into Array(array=w1688, new element=w1693) -> (w1684:dbl[])  [unwired: 1 in]
        n500 = Insert Into Array(array=w1690, new element=w1691) -> (w1686:dbl[])  [unwired: 1 in]
        n501 = case shown="True" w1698 {
          tunnel: w1699 -> [w1782 w1784]
          tunnel: [w1782 w1785] -> w1697
          tunnel: w1694 -> [_ w1783]
          frame False {
          }
          frame True {
            n502 = Insert Into Array(array=w1784, new element=w1783) -> (w1785:i32[])  [unwired: 1 in]
          }
        }
        n503 = case shown="True" "Plot sample extrema vs time" {
          tunnel: w1693 -> [_ w1813]
          tunnel: w1692 -> [_ w1814]
          tunnel: w1691 -> [_ w1815]
          tunnel: [w1792 w1802] -> w1682
          tunnel: w1696 -> [w1792 w1806]
          tunnel: w1720 -> [w1791 w1818]
          tunnel: w1719 -> [w1790 w1817]
          tunnel: w1718 -> [w1789 w1819]
          tunnel: w1717 -> [w1788 w1816]
          tunnel: w1716 -> [w1787 w1821]
          tunnel: w1715 -> [w1786 w1820]
          tunnel: [w1791 w1804] -> w1714
          tunnel: [w1790 w1797] -> w1713
          tunnel: [w1789 w1798] -> w1712
          tunnel: [w1788 w1822] -> w1711
          tunnel: [w1787 w1805] -> w1710
          tunnel: [w1786 w1799] -> w1709
          tunnel: w1697 -> [_ w1793]
          frame False {
          }
          frame True {
            w1800 = 1
            # "Number of VAR2 steps is 1."
            # "abs(Ig)"
            # "abs(Is)"
            # "abs(Id)"
            # "Adjusts graph colors."
            n504 = Absolute Value(x=w1815) -> (abs(x)=w1794:dbl[])
            n505 = Absolute Value(x=w1814) -> (abs(x)=w1795:dbl[])
            n506 = Absolute Value(x=w1813) -> (abs(x)=w1796:dbl[])
            n507 = Array Max & Min(array=w1796) -> (max value=w1812:dbl, min value=w1809:dbl)  [unwired: 2 out]
            n508 = Array Max & Min(array=w1795) -> (max value=w1811:dbl, min value=w1808:dbl)  [unwired: 2 out]
            n509 = Array Max & Min(array=w1794) -> (max value=w1810:dbl, min value=w1807:dbl)  [unwired: 2 out]
            n510 = local write "Id max"(w1811) -> ()
            n511 = local write "Id min"(w1808) -> ()
            n512 = local write "Ig max"(w1810) -> ()
            n513 = local write "Ig min"(w1807) -> ()
            n514 = Insert Into Array(array=w1821, new element=w1794) -> (w1805:dbl[])  [unwired: 1 in]
            n515 = Insert Into Array(array=w1820, new element=w1794) -> (w1799:dbl[])  [unwired: 1 in]
            n516 = local write "Is max"(w1812) -> ()
            n517 = local write "Is min"(w1809) -> ()
            n518 = Insert Into Array(array=w1819, new element=w1795) -> (w1798:dbl[])  [unwired: 1 in]
            n519 = Insert Into Array(array=w1816, new element=w1795) -> (w1822:dbl[])  [unwired: 1 in]
            n520 = Insert Into Array(array=w1818, new element=w1796) -> (w1804:dbl[])  [unwired: 1 in]
            n521 = Insert Into Array(array=w1817, new element=w1796) -> (w1797:dbl[])  [unwired: 1 in]
            n522 = control-ref of="Imax vs time"() -> (w1823:refnum<vi>)
            n523 = call "4155C Config Chart Colours.vi"("Numeric"=w1800, "XY Graph 2"=w1823) -> ()  [unwired: 6 in]
            n524 = call "4155C Split array.vi"("Number of VAR2 steps"=w1800, "Y2 data in"=w1798, "X data in"=w1793, "Y1 data in"=w1804, "Y3 data in"=w1805, "error in (no error)"=w1806) -> ("Array of clusters"=w1824:cluster{"Y data in":dbl[], "X data in":dbl[]}[], "error out"=w1803:errorcluster)  [unwired: 1 in]
            n525 = call "4155C Split array.vi"("Number of VAR2 steps"=w1800, "Y2 data in"=w1798, "X data in"=w1793, "Y1 data in"=w1797, "Y3 data in"=w1799, "error in (no error)"=w1803) -> ("Array of clusters"=w1801:cluster{"Y data in":dbl[], "X data in":dbl[]}[], "error out"=w1802:errorcluster)  [unwired: 1 in]
            n526 = local write "Imax vs time"(w1824) -> ()
            n527 = local write "Imin vs time"(w1801) -> ()
          }
        }
        n528 = Insert Into Array(array=w1687, new element=w1694) -> (w1685:dbl[])  [unwired: 1 in]
        n529 = control-ref of="I vs time (Bias Stress)"() -> (w1702:refnum<vi>)
        n530 = call "4155C Split array.vi"("Number of VAR2 steps"=w1695, "Y2 data in"=w1683, "X data in"=w1685, "Y1 data in"=w1684, "Y3 data in"=w1686) -> ("Array of clusters"=w1701:cluster{"Y data in":dbl[], "X data in":dbl[]}[])  [unwired: 2 in, 1 out]
        n531 = call "4155C Config Chart Colours.vi"("Numeric"=w1695, "XY Graph 2"=w1702) -> ()  [unwired: 6 in]
        n532 = local write "I vs time (Bias Stress)"(w1701) -> ()
        n533 = Insert Into Array(array=dbl[][] [] ("Input Array"), new element=w1694) -> (w1700:dbl[][])  [unwired: 2 in]
        n534 = Insert Into Array(array=w1700, new element=w1691) -> (w1754:dbl[][])  [unwired: 2 in]
        n535 = VISA Write(VISA resource name=w1741, write buffer=":DISP ON" ("write buffer (\"\")"), error in (no error)=w1682) -> (VISA resource name out=w1740:refnum<visa-resource-name>, error out=w1742:errorcluster)  [unwired: 1 out]
        n536 = Insert Into Array(array=w1754, new element=w1692) -> (w1753:dbl[][])  [unwired: 2 in]
        n537 = Insert Into Array(array=w1753, new element=w1693) -> (w1746:dbl[][])  [unwired: 2 in]
        n538 = Transpose 2D Array(2D array=w1746) -> (transposed array=w1745:dbl[][])
        n539 = call <vilib>:"compatOverwrite.vi"("overwrite (F)"=TRUE) -> ("overwrite?"=w1728:T8)
        n540 = Open/Create/Replace File(file path (use dialog)=w1751, error in=w1742, operation (0:open)=w1728) -> (refnum out=w1757:refnum<file>, error out=w1756:errorcluster)  [unwired: 3 in, 1 out]
        n541 = call "4155C Write array to file.vi"("Byte Stream File Refnum"=w1757, "Header"=string[] ["Time /Units", "Ig /A", "Id /A", "Is /A"], "Data Array"=w1745, "error in (no error)"=w1756) -> ("dup refnum"=w1759:refnum<file>, "error out"=w1758:errorcluster)  [unwired: 1 in]
        n542 = Close File(refnum=w1759, error in=w1758) -> (error out=w1749:errorcluster)  [unwired: 1 out]
      }
      frame "samplei" {
        w1837 = 1
        # "Adjusts graph colors."
        # "Add a time offset (elapsed time) to the time axis."
        n543 = local read "Sample I - Source/Common"() -> (w1849:u32)
        n544 = Number To Decimal String(number=w1872) -> (decimal integer string=w1920:string)  [unwired: 1 in]
        n545 = local read "Sample I - Probe 4 (Disabled)"() -> (w1852:u32)
        n546 = Concatenate Strings(w1901, "-samplei-" ("Substring"), w1920, w1871, ".txt" ("Substring")) -> (w1918:string)
        n547 = Fract/Exp String To Number(string=w1917) -> (number=w1886:dbl[])  [unwired: 3 in, 1 out]
        n548 = String To Path(string=w1918) -> (path=w1904:path)
        n549 = local read "Sample I - Probe 3 (Disabled)"() -> (w1851:u32)
        n550 = Index Array(array=w1886, index=4 ("Index")) -> (element=w1880:dbl)
        n551 = Index Array(array=w1886, index=3 ("Index")) -> (element=w1881:dbl)
        n552 = Index Array(array=w1886, index=1 ("Index")) -> (element=w1883:dbl)
        n553 = Index Array(array=w1886, index=0 ("Index")) -> (element=w1884:dbl)
        n554 = Index Array(array=w1886, index=2 ("Index")) -> (element=w1882:dbl)
        n555 = local read "Sample I - Drain/Gate"() -> (w1850:u32)
        n556 = call "4155C Config SamplingI Measurements v3.0.vi"("VISA session"=w1923, "Num Points"=w1883, "Sample I - Probe 3 (Disabled)"=w1851, "Display on/off"=TRUE, "Sample I - Source/Common"=w1849, "Sample I - Drain/Gate"=w1850, "Sampling interval"=w1881, "Standby"=w1853, "error in (no error)"=w1922, "Timings"=w1893, "Sample I - Probe 4 (Disabled)"=w1852, "Sample time"=w1882) -> ("dup VISA resource name"=w1925:refnum<visa-resource-name>, "error out"=w1924:errorcluster)  [unwired: 2 in]
        n557 = local read "Plot sample extrema vs time"() -> (w1846:bool)
        n558 = local read "Time Units"() -> (w1842:u16)
        n559 = call "4155C Take SampleI v3.0.vi"("Sample I - Drain/Gate"=w1850, "Emergency Stop"=w1898, "error in (no error)"=w1924, "Idg 2"=w1884, "Vdg compliance 2"=w1880, "VISA resource name in"=w1925) -> ("error out"=w1896:errorcluster, "Idg"=w1829:dbl[], "Vdg"=w1830:dbl[], "VISA Resource Name out"=w1894:refnum<visa-resource-name>, "Is"=w1826:dbl[], "Time"=w1841:dbl[])
        n560 = case shown="0, Default" w1842 {
          tunnel: [w1928 w1929 w1932] -> w1843
          tunnel: w1841 -> [w1927 w1929 w1931]
          frame 2 {
            n561 = Divide(x=w1927, y=3600.0) -> (x/y=w1928:dbl[])
          }
          frame 0, Default {
          }
          frame 1 {
            n562 = Divide(x=w1931, y=60.0) -> (x/y=w1932:dbl[])
          }
        }
        n563 = Add(x=w1843, y=w1840) -> (x+y=w1835:dbl[])
        n564 = Insert Into Array(array=w1836, new element=w1835) -> (w1834:dbl[])  [unwired: 1 in]
        n565 = case shown="True" w1846 {
          tunnel: w1845 -> [w1933 w1935]
          tunnel: [w1933 w1936] -> w1844
          tunnel: w1835 -> [_ w1934]
          frame False {
          }
          frame True {
            n566 = Insert Into Array(array=w1935, new element=w1934) -> (w1936:i32[])  [unwired: 1 in]
          }
        }
        n567 = control-ref of="Vdg vs time (Bias Stress)"() -> (w1839:refnum<vi>)
        n568 = Insert Into Array(array=dbl[][] [] ("Input Array"), new element=w1835) -> (w1908:dbl[][])  [unwired: 2 in]
        n569 = call "4155C Config Chart Colours.vi"("Numeric"=w1837, "XY Graph 2"=w1839) -> ()  [unwired: 6 in]
        n570 = Insert Into Array(array=w1833, new element=w1830) -> (w1825:dbl[])  [unwired: 1 in]
        n571 = call "4155C Split array.vi"("Number of VAR2 steps"=w1837, "X data in"=w1834, "Y1 data in"=w1825) -> ("Array of clusters"=w1838:cluster{"Y data in":dbl[], "X data in":dbl[]}[])  [unwired: 4 in, 1 out]
        n572 = local write "Vdg vs time (Bias Stress)"(w1838) -> ()
        n573 = Insert Into Array(array=w1832, new element=w1829) -> (w1831:dbl[])  [unwired: 1 in]
        n574 = Insert Into Array(array=w1908, new element=w1830) -> (w1907:dbl[][])  [unwired: 2 in]
        n575 = Insert Into Array(array=w1828, new element=w1826) -> (w1827:dbl[])  [unwired: 1 in]
        n576 = Insert Into Array(array=w1907, new element=w1829) -> (w1906:dbl[][])  [unwired: 2 in]
        n577 = VISA Write(VISA resource name=w1894, write buffer=":DISP ON" ("write buffer (\"\")"), error in (no error)=w1896) -> (VISA resource name out=w1879:refnum<visa-resource-name>, error out=w1895:errorcluster)  [unwired: 1 out]
        n578 = Insert Into Array(array=w1906, new element=w1826) -> (w1900:dbl[][])  [unwired: 2 in]
        n579 = call <vilib>:"compatOverwrite.vi"("overwrite (F)"=TRUE) -> ("overwrite?"=w1874:T8)
        n580 = Open/Create/Replace File(file path (use dialog)=w1904, error in=w1895, operation (0:open)=w1874) -> (refnum out=w1911:refnum<file>, error out=w1910:errorcluster)  [unwired: 3 in, 1 out]
        n581 = Transpose 2D Array(2D array=w1900) -> (transposed array=w1899:dbl[][])
        n582 = call "4155C Write array to file.vi"("Byte Stream File Refnum"=w1911, "Header"=string[] ["Time /s", "Vdg /V", "Idg /A", "Is /A"], "Data Array"=w1899, "error in (no error)"=w1910) -> ("dup refnum"=w1913:refnum<file>, "error out"=w1912:errorcluster)  [unwired: 1 in]
        n583 = Close File(refnum=w1913, error in=w1912) -> (error out=w1877:errorcluster)  [unwired: 1 out]
        n584 = VISA Write(VISA resource name=w1879, write buffer=";:PAGE:SCON:STAN OFF;:PAGE:CHAN:VSU2:DIS;" ("write buffer (\"\")"), error in (no error)=w1877) -> (VISA resource name out=w1875:refnum<visa-resource-name>, error out=w1876:errorcluster)  [unwired: 1 out]
      }
      frame "#" {
        n585 = VISA Write(VISA resource name=w1965, write buffer=":DISP ON" ("write buffer (\"\")"), error in (no error)=w1964) -> (VISA resource name out=w1963:refnum<visa-resource-name>, error out=w1962:errorcluster)  [unwired: 1 out]
      }
      frame "stressV" {
        n586 = Number To Decimal String(number=w2000) -> (decimal integer string=w2041:string)  [unwired: 1 in]
        n587 = Concatenate Strings(w2025, "-stressV-" ("Substring"), w2041, w1999, ".txt" ("Substring")) -> (w2039:string)
        n588 = Fract/Exp String To Number(string=w2038) -> (number=w2011:dbl[])  [unwired: 3 in, 1 out]
        n589 = local read "Stress V - Drain"() -> (w1978:u32)
        n590 = String To Path(string=w2039) -> (path=w2029:path)
        n591 = Index Array(array=w2011, index=3 ("Index")) -> (element=w2008:dbl)
        n592 = Index Array(array=w2011, index=1 ("Index")) -> (element=w2006:dbl)
        n593 = Index Array(array=w2011, index=0 ("Index")) -> (element=w2005:dbl)
        n594 = Index Array(array=w2011, index=4 ("Index")) -> (element=w2010:dbl)
        n595 = Index Array(array=w2011, index=2 ("Index")) -> (element=w2007:dbl)
        n596 = local read "Stress V - Gate"() -> (w1979:u32)
        n597 = local read "Stress V - Source/Common"() -> (w1980:u32)
        n598 = call "4155C Config V Stress v3.0.vi"("Display on/off"=TRUE, "Stress V - Gate"=w1979, "Stress V - Drain"=w1978, "Stress V - Source/Common"=w1980, "IG compliance"=w2007, "ID compliance"=w2008, "error in (no error)"=w2043, "VG"=w2005, "VD"=w2006, "VISA session"=w2044) -> ("error out"=w2045:errorcluster, "dup VISA resource name"=w2046:refnum<visa-resource-name>)
        n599 = call "4155C Apply Stress.vi"("error in (no error)"=w2045, "Duration"=w2010, "Emergency Stop"=w2024, "VISA resource name in"=w2046) -> ("error out"=w2022:errorcluster, "VISA Resource Name out"=w2020:refnum<visa-resource-name>)
        n600 = VISA Write(VISA resource name=w2020, write buffer=":DISP ON" ("write buffer (\"\")"), error in (no error)=w2022) -> (VISA resource name out=w2019:refnum<visa-resource-name>, error out=w2021:errorcluster)  [unwired: 1 out]
        n601 = call <vilib>:"compatOverwrite.vi"("overwrite (F)"=TRUE) -> ("overwrite?"=w2004:T8)
        n602 = Open/Create/Replace File(file path (use dialog)=w2029, error in=w2021, operation (0:open)=w2004) -> (refnum out=w2032:refnum<file>, error out=w2031:errorcluster)  [unwired: 3 in, 1 out]
        n603 = call "4155C Write array to file.vi"("Byte Stream File Refnum"=w2032, "Header"=string[] ["V stress completed successfully", ""], "error in (no error)"=w2031) -> ("dup refnum"=w2034:refnum<file>, "error out"=w2033:errorcluster)  [unwired: 2 in]
        n604 = Close File(refnum=w2034, error in=w2033) -> (error out=w2027:errorcluster)  [unwired: 1 out]
      }
      frame "stressI" {
        n605 = Number To Decimal String(number=w2072) -> (decimal integer string=w2109:string)  [unwired: 1 in]
        n606 = Concatenate Strings(w2093, "-stressI-" ("Substring"), w2109, w2071, ".txt" ("Substring")) -> (w2107:string)
        n607 = Fract/Exp String To Number(string=w2106) -> (number=w2081:dbl[])  [unwired: 3 in, 1 out]
        n608 = local read "Stress I - Source/Common"() -> (w2051:u32)
        n609 = Index Array(array=w2081, index=1 ("Index")) -> (element=w2077:dbl)
        n610 = Index Array(array=w2081, index=0 ("Index")) -> (element=w2078:dbl)
        n611 = Index Array(array=w2081, index=2 ("Index")) -> (element=w2079:dbl)
        n612 = String To Path(string=w2107) -> (path=w2097:path)
        n613 = local read "Stress I - Drain/Gate"() -> (w2052:u32)
        n614 = call "4155C Config I Stress v3.0.vi"("Stress I - Drain/Gate"=w2052, "Stress I - Source/Common"=w2051, "Display on/off"=TRUE, "error in (no error)"=w2111, "VDG compliance"=w2077, "IDG"=w2078, "VISA session"=w2112) -> ("error out"=w2113:errorcluster, "dup VISA resource name"=w2114:refnum<visa-resource-name>)  [unwired: 1 in]
        n615 = call "4155C Apply Stress.vi"("error in (no error)"=w2113, "Duration"=w2079, "Emergency Stop"=w2092, "VISA resource name in"=w2114) -> ("error out"=w2090:errorcluster, "VISA Resource Name out"=w2088:refnum<visa-resource-name>)
        n616 = VISA Write(VISA resource name=w2088, write buffer=":DISP ON" ("write buffer (\"\")"), error in (no error)=w2090) -> (VISA resource name out=w2087:refnum<visa-resource-name>, error out=w2089:errorcluster)  [unwired: 1 out]
        n617 = call <vilib>:"compatOverwrite.vi"("overwrite (F)"=TRUE) -> ("overwrite?"=w2076:T8)
        n618 = Open/Create/Replace File(file path (use dialog)=w2097, error in=w2089, operation (0:open)=w2076) -> (refnum out=w2100:refnum<file>, error out=w2099:errorcluster)  [unwired: 3 in, 1 out]
        n619 = call "4155C Write array to file.vi"("Byte Stream File Refnum"=w2100, "Header"=string[] ["I stress completed successfully", ""], "error in (no error)"=w2099) -> ("dup refnum"=w2102:refnum<file>, "error out"=w2101:errorcluster)  [unwired: 2 in]
        n620 = Close File(refnum=w2102, error in=w2101) -> (error out=w2095:errorcluster)  [unwired: 1 out]
      }
      frame "vsu2pulse" {
        n621 = Number To Decimal String(number=w2139) -> (decimal integer string=w2174:string)  [unwired: 1 in]
        n622 = Concatenate Strings(w2159, "-vsu2-" ("Substring"), w2174, w2138, ".txt" ("Substring")) -> (w2172:string)
        n623 = Fract/Exp String To Number(string=w2171) -> (number=w2147:dbl[])  [unwired: 3 in, 1 out]
        n624 = String To Path(string=w2172) -> (path=w2163:path)
        n625 = Index Array(array=w2147, index=1 ("Index")) -> (element=w2146:dbl)
        n626 = Index Array(array=w2147, index=0 ("Index")) -> (element=w2144:dbl)
        n627 = local read "VSU2 Stress - Source/Common"() -> (w2119:u32)
        n628 = call "4155C Config VSU2 Stress v3.0.vi"("VISA session"=w2177, "Display on/off"=TRUE, "VSU2"=w2144, "error in (no error)"=w2176, "VSU2 Stress - Source/Common"=w2119) -> ("dup VISA resource name"=w2179:refnum<visa-resource-name>, "error out"=w2178:errorcluster)
        n629 = call "4155C Apply Stress.vi"("error in (no error)"=w2178, "Duration"=w2146, "Emergency Stop"=w2158, "VISA resource name in"=w2179) -> ("error out"=w2156:errorcluster, "VISA Resource Name out"=w2154:refnum<visa-resource-name>)
        n630 = VISA Write(VISA resource name=w2154, write buffer=":DISP ON" ("write buffer (\"\")"), error in (no error)=w2156) -> (VISA resource name out=w2153:refnum<visa-resource-name>, error out=w2155:errorcluster)  [unwired: 1 out]
        n631 = call <vilib>:"compatOverwrite.vi"("overwrite (F)"=TRUE) -> ("overwrite?"=w2143:T8)
        n632 = Open/Create/Replace File(file path (use dialog)=w2163, error in=w2155, operation (0:open)=w2143) -> (refnum out=w2166:refnum<file>, error out=w2165:errorcluster)  [unwired: 3 in, 1 out]
        n633 = call "4155C Write array to file.vi"("Byte Stream File Refnum"=w2166, "Header"=string[] ["VSU2 pulse completed successfully", ""], "error in (no error)"=w2165) -> ("dup refnum"=w2168:refnum<file>, "error out"=w2167:errorcluster)  [unwired: 2 in]
        n634 = Close File(refnum=w2168, error in=w2167) -> (error out=w2161:errorcluster)  [unwired: 1 out]
      }
      frame "sample-fpp" {
        w2191 = 1
        w2249 = string[] ["Time /s", "Id VgVd /A", "Ig VgVd /A", "Vp1 VgVd /V", "Vp2 VgVd /V"] ("Header")
        w2253 = "%d" ("format string")
        # "Y1 = Y2 = ID\nY3 = IG"
        # "Y1 = Vp2\nY2 = Y3 = Vp1"
        # "Add a time offset (elapsed time) to the time axis."
        n635 = local read "FPP - Drain"() -> (w2226:u32)
        n636 = local read "FPP - Source"() -> (w2225:u32)
        n637 = local read "Plot sample extrema vs time"() -> (w2199:bool)
        n638 = Fract/Exp String To Number(string=w2292) -> (number=w2280:dbl[])  [unwired: 3 in, 1 out]
        n639 = local read "FPP - Probe 1"() -> (w2229:u32)
        n640 = Number To Decimal String(number=w2241) -> (decimal integer string=w2295:string)  [unwired: 1 in]
        n641 = local read "Plot sample extrema vs time"() -> (w2202:bool)
        n642 = Concatenate Strings(w2286, "-samplefpp-" ("Substring"), w2295, w2240, ".txt" ("Substring")) -> (w2293:string)
        n643 = local read "FPP - Gate"() -> (w2227:u32)
        n644 = local read "Time Units"() -> (w2217:u16)
        n645 = String To Path(string=w2293) -> (path=w2261:path)
        n646 = local read "FPP - Probe 2"() -> (w2228:u32)
        n647 = Index Array(array=w2280, index=0 ("Index")) -> (element=w2248:dbl)
        n648 = Index Array(array=w2280, index=1 ("Index")) -> (element=w2247:dbl)
        n649 = control-ref of="I vs time (Bias Stress)"() -> (w2219:refnum<vi>)
        n650 = Index Array(array=w2280, index=2 ("Index")) -> (element=w2288:dbl)
        n651 = Index Array(array=w2280, index=3 ("Index")) -> (element=w2278:dbl)
        n652 = call "4155C Config Sampling Measurements FPP v3.0.vi"("VISA session"=w2298, "Gate Compliance"=w2287, "FPP - Source"=w2225, "FPP - Drain"=w2226, "Drain Compliance"=w2296, "error in (no error)"=w2297, "Num Points"=w2288, "Timings"=w2285, "FPP - Gate"=w2227, "FPP - Probe 1"=w2229, "Vg"=w2248, "Vd"=w2247, "Display on/off"=TRUE, "Sample time"=w2278, "FPP - Probe 2"=w2228, "Standby"=w2230) -> ("dup VISA resource name"=w2263:refnum<visa-resource-name>, "error out"=w2262:errorcluster)  [unwired: 2 in]
        n653 = Number To Decimal String(number=w2248) -> (decimal integer string=w2269:string)  [unwired: 1 in]
        n654 = call "4155C Take Sample FPP.vi"("VISA resource name in"=w2263, "error in (no error)"=w2262, "Emergency Stop"=w2264) -> ("Time"=w2216:dbl[], "Vp1"=w2185:dbl[], "VISA Resource Name out"=w2245:refnum<visa-resource-name>, "Ig"=w2196:dbl[], "Id"=w2195:dbl[], "Vp2"=w2184:dbl[], "error out"=w2198:errorcluster)  [unwired: 10 in]
        n655 = Insert Into Array(array=w2223, new element=w2195) -> (w2182:dbl[])  [unwired: 1 in]
        n656 = Insert Into Array(array=w2224, new element=w2196) -> (w2221:dbl[])  [unwired: 1 in]
        n657 = case shown="0, Default" w2217 {
          tunnel: [w2338 w2339 w2342] -> w2218
          tunnel: w2216 -> [w2337 w2339 w2341]
          frame 2 {
            n658 = Divide(x=w2337, y=3600.0) -> (x/y=w2338:dbl[])
          }
          frame 0, Default {
          }
          frame 1 {
            n659 = Divide(x=w2341, y=60.0) -> (x/y=w2342:dbl[])
          }
        }
        n660 = Add(x=w2218, y=w2215) -> (x+y=w2189:dbl[])
        n661 = case shown="True" w2199 {
          tunnel: w2201 -> [w2299 w2301]
          tunnel: [w2299 w2302] -> w2200
          tunnel: w2189 -> [_ w2300]
          frame False {
          }
          frame True {
            n662 = Insert Into Array(array=w2301, new element=w2300) -> (w2302:i32[])  [unwired: 1 in]
          }
        }
        n663 = Insert Into Array(array=w2222, new element=w2189) -> (w2190:dbl[])  [unwired: 1 in]
        n664 = case shown="True" w2202 {
          tunnel: w2195 -> [_ w2327]
          tunnel: w2196 -> [_ w2328]
          tunnel: [w2309 w2319] -> w2197
          tunnel: w2198 -> [w2309 w2322]
          tunnel: w2214 -> [w2308 w2312]
          tunnel: w2213 -> [w2307 w2311]
          tunnel: w2212 -> [w2306 w2330]
          tunnel: w2211 -> [w2305 w2329]
          tunnel: w2210 -> [w2304 w2332]
          tunnel: w2209 -> [w2303 w2331]
          tunnel: [w2308 w2312] -> w2208
          tunnel: [w2307 w2311] -> w2207
          tunnel: [w2306 w2310] -> w2206
          tunnel: [w2305 w2333] -> w2205
          tunnel: [w2304 w2321] -> w2204
          tunnel: [w2303 w2316] -> w2203
          tunnel: w2200 -> [_ w2313]
          frame False {
          }
          frame True {
            w2317 = 1
            # "Y1 = Y2 = ID\nY3 = IG"
            # "Number of VAR2 steps is 1."
            # "abs(Ig)"
            # "abs(Id)"
            # "Adjusts graph colors."
            n665 = Absolute Value(x=w2328) -> (abs(x)=w2314:dbl[])
            n666 = Absolute Value(x=w2327) -> (abs(x)=w2315:dbl[])
            n667 = Array Max & Min(array=w2315) -> (max value=w2326:dbl, min value=w2324:dbl)  [unwired: 2 out]
            n668 = Array Max & Min(array=w2314) -> (max value=w2325:dbl, min value=w2323:dbl)  [unwired: 2 out]
            n669 = local write "Id max"(w2326) -> ()
            n670 = local write "Id min"(w2324) -> ()
            n671 = local write "Ig max"(w2325) -> ()
            n672 = local write "Ig min"(w2323) -> ()
            n673 = Insert Into Array(array=w2332, new element=w2314) -> (w2321:dbl[])  [unwired: 1 in]
            n674 = Insert Into Array(array=w2331, new element=w2314) -> (w2316:dbl[])  [unwired: 1 in]
            n675 = Insert Into Array(array=w2330, new element=w2315) -> (w2310:dbl[])  [unwired: 1 in]
            n676 = Insert Into Array(array=w2329, new element=w2315) -> (w2333:dbl[])  [unwired: 1 in]
            n677 = control-ref of="Imax vs time"() -> (w2334:refnum<vi>)
            n678 = call "4155C Config Chart Colours.vi"("Numeric"=w2317, "XY Graph 2"=w2334) -> ()  [unwired: 6 in]
            n679 = call "4155C Split array.vi"("Number of VAR2 steps"=w2317, "Y2 data in"=w2310, "X data in"=w2313, "Y1 data in"=w2310, "Y3 data in"=w2321, "error in (no error)"=w2322) -> ("Array of clusters"=w2335:cluster{"Y data in":dbl[], "X data in":dbl[]}[], "error out"=w2320:errorcluster)  [unwired: 1 in]
            n680 = call "4155C Split array.vi"("Number of VAR2 steps"=w2317, "Y2 data in"=w2310, "X data in"=w2313, "Y1 data in"=w2310, "Y3 data in"=w2316, "error in (no error)"=w2320) -> ("Array of clusters"=w2318:cluster{"Y data in":dbl[], "X data in":dbl[]}[], "error out"=w2319:errorcluster)  [unwired: 1 in]
            n681 = local write "Imax vs time"(w2335) -> ()
            n682 = local write "Imin vs time"(w2318) -> ()
          }
        }
        n683 = call "4155C Split array.vi"("Number of VAR2 steps"=w2191, "Y2 data in"=w2182, "X data in"=w2190, "Y1 data in"=w2182, "Y3 data in"=w2221) -> ("Array of clusters"=w2220:cluster{"Y data in":dbl[], "X data in":dbl[]}[])  [unwired: 2 in, 1 out]
        n684 = call "4155C Config Chart Colours.vi"("Numeric"=w2191, "XY Graph 2"=w2219) -> ()  [unwired: 6 in]
        n685 = local write "I vs time (Bias Stress)"(w2220) -> ()
        n686 = Number To Decimal String(number=w2247) -> (decimal integer string=w2267:string)  [unwired: 1 in]
        n687 = Insert Into Array(array=w2188, new element=w2185) -> (w2183:dbl[])  [unwired: 1 in]
        n688 = Concatenate Strings("(Vg = " ("Substring"), w2269, "V, Vd = " ("Substring"), w2267, "V)" ("Substring")) -> (w2265:string)
        n689 = Insert Into Array(array=dbl[][] [] ("Input Array"), new element=w2189) -> (w2276:dbl[][])  [unwired: 2 in]
        n690 = Insert Into Array(array=w2187, new element=w2184) -> (w2186:dbl[])  [unwired: 1 in]
        n691 = Insert Into Array(array=w2276, new element=w2195) -> (w2275:dbl[][])  [unwired: 2 in]
        n692 = control-ref of="Vp vs time (FPP Bias Stress)"() -> (w2192:refnum<vi>)
        n693 = Insert Into Array(array=w2275, new element=w2196) -> (w2274:dbl[][])  [unwired: 2 in]
        n694 = Insert Into Array(array=w2274, new element=w2185) -> (w2272:dbl[][])  [unwired: 2 in]
        n695 = call "4155C Config Chart Colours.vi"("Numeric"=w2191, "XY Graph 2"=w2192) -> ()  [unwired: 6 in]
        n696 = call "4155C Split array.vi"("Number of VAR2 steps"=w2191, "Y2 data in"=w2183, "X data in"=w2190, "Y1 data in"=w2186, "Y3 data in"=w2183) -> ("Array of clusters"=w2193:cluster{"Y data in":dbl[], "X data in":dbl[]}[])  [unwired: 2 in, 1 out]
        n697 = Array To Spreadsheet String(array=w2249, 3:w2253) -> (spreadsheet string=w2255:string)  [unwired: 1 in]
        n698 = Insert Into Array(array=w2272, new element=w2184) -> (w2246:dbl[][])  [unwired: 2 in]
        n699 = Search and Replace String(replace all?=TRUE ("replace all? (F)"), input string=w2255, search string="VgVd", replace string=w2265) -> (result string=w2251:string)  [unwired: 4 in, 3 out]
        n700 = local write "Vp vs time (FPP Bias Stress)"(w2193) -> ()
        n701 = Spreadsheet String To Array(format string=w2253, spreadsheet string=w2251, array type (2D Dbl)=w2249) -> (array=w2250:string[])  [unwired: 1 in]
        n702 = Transpose 2D Array(2D array=w2246) -> (transposed array=w2271:dbl[][])
        n703 = call <vilib>:"compatOverwrite.vi"("overwrite (F)"=TRUE) -> ("overwrite?"=w2243:T8)
        n704 = Open/Create/Replace File(file path (use dialog)=w2261, error in=w2197, operation (0:open)=w2243) -> (refnum out=w2258:refnum<file>, error out=w2259:errorcluster)  [unwired: 3 in, 1 out]
        n705 = call "4155C Write array to file.vi"("Byte Stream File Refnum"=w2258, "Header"=w2250, "Data Array"=w2271, "error in (no error)"=w2259) -> ("dup refnum"=w2256:refnum<file>, "error out"=w2257:errorcluster)  [unwired: 1 in]
        n706 = Close File(refnum=w2256, error in=w2257) -> (error out=w2244:errorcluster)  [unwired: 1 out]
      }
      frame "resample-fpp" {
        w2354 = 1
        w2409 = string[] ["Time /s", "Id VgVd /A", "Ig VgVd /A", "Vp1 VgVd /V", "Vp2 VgVd /V"] ("Header")
        w2413 = "%d" ("format string")
        # "Y1 = Y2 = ID\nY3 = IG"
        # "Y1 = Vp2\nY2 = Y3 = Vp1"
        # "Add a time offset (elapsed time) to the time axis."
        n707 = Number To Decimal String(number=w2397) -> (decimal integer string=w2447:string)  [unwired: 1 in]
        n708 = Fract/Exp String To Number(string=w2444) -> (number=w2402:dbl[])  [unwired: 3 in, 1 out]
        n709 = Concatenate Strings(w2440, "-resamplefpp-" ("Substring"), w2447, w2398, ".txt" ("Substring")) -> (w2445:string)
        n710 = local read "Time Units"() -> (w2378:u16)
        n711 = local read "Plot sample extrema vs time"() -> (w2376:bool)
        n712 = String To Path(string=w2445) -> (path=w2421:path)
        n713 = Index Array(array=w2402, index=0 ("Index")) -> (element=w2408:dbl)
        n714 = Index Array(array=w2402, index=1 ("Index")) -> (element=w2407:dbl)
        n715 = Number To Decimal String(number=w2408) -> (decimal integer string=w2427:string)  [unwired: 1 in]
        n716 = call "4155C Take Sample FPP.vi"("VISA resource name in"=w2404, "error in (no error)"=w2403, "Emergency Stop"=w2422) -> ("Time"=w2379:dbl[], "Vp1"=w2348:dbl[], "VISA Resource Name out"=w2406:refnum<visa-resource-name>, "Ig"=w2359:dbl[], "Id"=w2358:dbl[], "Vp2"=w2347:dbl[], "error out"=w2361:errorcluster)  [unwired: 10 in]
        n717 = Insert Into Array(array=w2386, new element=w2358) -> (w2345:dbl[])  [unwired: 1 in]
        n718 = case shown="0, Default" w2378 {
          tunnel: [w2488 w2489 w2492] -> w2380
          tunnel: w2379 -> [w2487 w2489 w2491]
          frame 2 {
            n719 = Divide(x=w2487, y=3600.0) -> (x/y=w2488:dbl[])
          }
          frame 0, Default {
          }
          frame 1 {
            n720 = Divide(x=w2491, y=60.0) -> (x/y=w2492:dbl[])
          }
        }
        n721 = Insert Into Array(array=w2387, new element=w2359) -> (w2384:dbl[])  [unwired: 1 in]
        n722 = control-ref of="I vs time (Bias Stress)"() -> (w2382:refnum<vi>)
        n723 = Number To Decimal String(number=w2407) -> (decimal integer string=w2425:string)  [unwired: 1 in]
        n724 = Add(x=w2380, y=w2381) -> (x+y=w2352:dbl[])
        n725 = Insert Into Array(array=w2385, new element=w2352) -> (w2353:dbl[])  [unwired: 1 in]
        n726 = call "4155C Split array.vi"("Number of VAR2 steps"=w2354, "Y2 data in"=w2345, "X data in"=w2353, "Y1 data in"=w2345, "Y3 data in"=w2384) -> ("Array of clusters"=w2383:cluster{"Y data in":dbl[], "X data in":dbl[]}[])  [unwired: 2 in, 1 out]
        n727 = Concatenate Strings("(Vg = " ("Substring"), w2427, "V, Vd = " ("Substring"), w2425, "V)" ("Substring")) -> (w2423:string)
        n728 = call "4155C Config Chart Colours.vi"("Numeric"=w2354, "XY Graph 2"=w2382) -> ()  [unwired: 6 in]
        n729 = local write "I vs time (Bias Stress)"(w2383) -> ()
        n730 = Insert Into Array(array=dbl[][] [] ("Input Array"), new element=w2352) -> (w2434:dbl[][])  [unwired: 2 in]
        n731 = Insert Into Array(array=w2434, new element=w2358) -> (w2433:dbl[][])  [unwired: 2 in]
        n732 = Insert Into Array(array=w2433, new element=w2359) -> (w2432:dbl[][])  [unwired: 2 in]
        n733 = Array To Spreadsheet String(array=w2409, 3:w2413) -> (spreadsheet string=w2415:string)  [unwired: 1 in]
        n734 = Insert Into Array(array=w2432, new element=w2348) -> (w2430:dbl[][])  [unwired: 2 in]
        n735 = Insert Into Array(array=w2351, new element=w2348) -> (w2346:dbl[])  [unwired: 1 in]
        n736 = Search and Replace String(replace all?=TRUE ("replace all? (F)"), input string=w2415, search string="VgVd", replace string=w2423) -> (result string=w2411:string)  [unwired: 4 in, 3 out]
        n737 = Insert Into Array(array=w2430, new element=w2347) -> (w2401:dbl[][])  [unwired: 2 in]
        n738 = Insert Into Array(array=w2350, new element=w2347) -> (w2349:dbl[])  [unwired: 1 in]
        n739 = Spreadsheet String To Array(format string=w2413, spreadsheet string=w2411, array type (2D Dbl)=w2409) -> (array=w2410:string[])  [unwired: 1 in]
        n740 = control-ref of="Vp vs time (FPP Bias Stress)"() -> (w2355:refnum<vi>)
        n741 = local read "Plot sample extrema vs time"() -> (w2363:bool)
        n742 = call <vilib>:"compatOverwrite.vi"("overwrite (F)"=TRUE) -> ("overwrite?"=w2400:T8)
        n743 = Transpose 2D Array(2D array=w2401) -> (transposed array=w2429:dbl[][])
        n744 = call "4155C Config Chart Colours.vi"("Numeric"=w2354, "XY Graph 2"=w2355) -> ()  [unwired: 6 in]
        n745 = call "4155C Split array.vi"("Number of VAR2 steps"=w2354, "Y2 data in"=w2346, "X data in"=w2353, "Y1 data in"=w2349, "Y3 data in"=w2346) -> ("Array of clusters"=w2356:cluster{"Y data in":dbl[], "X data in":dbl[]}[])  [unwired: 2 in, 1 out]
        n746 = case shown="True" w2363 {
          tunnel: w2364 -> [w2449 w2451]
          tunnel: [w2449 w2452] -> w2362
          tunnel: w2352 -> [_ w2450]
          frame False {
          }
          frame True {
            n747 = Insert Into Array(array=w2451, new element=w2450) -> (w2452:i32[])  [unwired: 1 in]
          }
        }
        n748 = case shown="True" w2376 {
          tunnel: w2358 -> [_ w2477]
          tunnel: w2359 -> [_ w2478]
          tunnel: [w2459 w2469] -> w2360
          tunnel: w2361 -> [w2459 w2472]
          tunnel: w2377 -> [w2458 w2462]
          tunnel: w2374 -> [w2457 w2461]
          tunnel: w2373 -> [w2456 w2480]
          tunnel: w2372 -> [w2455 w2479]
          tunnel: w2371 -> [w2454 w2482]
          tunnel: w2370 -> [w2453 w2481]
          tunnel: [w2458 w2462] -> w2375
          tunnel: [w2457 w2461] -> w2365
          tunnel: [w2456 w2460] -> w2367
          tunnel: [w2455 w2483] -> w2366
          tunnel: [w2454 w2471] -> w2369
          tunnel: [w2453 w2466] -> w2368
          tunnel: w2362 -> [_ w2463]
          frame False {
          }
          frame True {
            w2467 = 1
            # "Y1 = Y2 = ID\nY3 = IG"
            # "Number of VAR2 steps is 1."
            # "abs(Ig)"
            # "abs(Id)"
            # "Adjusts graph colors."
            n749 = Absolute Value(x=w2478) -> (abs(x)=w2464:dbl[])
            n750 = Absolute Value(x=w2477) -> (abs(x)=w2465:dbl[])
            n751 = Array Max & Min(array=w2465) -> (max value=w2476:dbl, min value=w2474:dbl)  [unwired: 2 out]
            n752 = Array Max & Min(array=w2464) -> (max value=w2475:dbl, min value=w2473:dbl)  [unwired: 2 out]
            n753 = local write "Id max"(w2476) -> ()
            n754 = local write "Id min"(w2474) -> ()
            n755 = local write "Ig max"(w2475) -> ()
            n756 = local write "Ig min"(w2473) -> ()
            n757 = Insert Into Array(array=w2482, new element=w2464) -> (w2471:dbl[])  [unwired: 1 in]
            n758 = Insert Into Array(array=w2481, new element=w2464) -> (w2466:dbl[])  [unwired: 1 in]
            n759 = Insert Into Array(array=w2480, new element=w2465) -> (w2460:dbl[])  [unwired: 1 in]
            n760 = Insert Into Array(array=w2479, new element=w2465) -> (w2483:dbl[])  [unwired: 1 in]
            n761 = control-ref of="Imax vs time"() -> (w2484:refnum<vi>)
            n762 = call "4155C Config Chart Colours.vi"("Numeric"=w2467, "XY Graph 2"=w2484) -> ()  [unwired: 6 in]
            n763 = call "4155C Split array.vi"("Number of VAR2 steps"=w2467, "Y2 data in"=w2460, "X data in"=w2463, "Y1 data in"=w2460, "Y3 data in"=w2471, "error in (no error)"=w2472) -> ("Array of clusters"=w2485:cluster{"Y data in":dbl[], "X data in":dbl[]}[], "error out"=w2470:errorcluster)  [unwired: 1 in]
            n764 = call "4155C Split array.vi"("Number of VAR2 steps"=w2467, "Y2 data in"=w2460, "X data in"=w2463, "Y1 data in"=w2460, "Y3 data in"=w2466, "error in (no error)"=w2470) -> ("Array of clusters"=w2468:cluster{"Y data in":dbl[], "X data in":dbl[]}[], "error out"=w2469:errorcluster)  [unwired: 1 in]
            n765 = local write "Imax vs time"(w2485) -> ()
            n766 = local write "Imin vs time"(w2468) -> ()
          }
        }
        n767 = Open/Create/Replace File(file path (use dialog)=w2421, error in=w2360, operation (0:open)=w2400) -> (refnum out=w2418:refnum<file>, error out=w2419:errorcluster)  [unwired: 3 in, 1 out]
        n768 = call "4155C Write array to file.vi"("Byte Stream File Refnum"=w2418, "Header"=w2410, "Data Array"=w2429, "error in (no error)"=w2419) -> ("dup refnum"=w2416:refnum<file>, "error out"=w2417:errorcluster)  [unwired: 1 in]
        n769 = local write "Vp vs time (FPP Bias Stress)"(w2356) -> ()
        n770 = Close File(refnum=w2416, error in=w2417) -> (error out=w2405:errorcluster)  [unwired: 1 out]
      }
      frame "serial" {
        n771 = local read "Termination char\n(0xA = '\\n' = LF)\n(0xD = '\\r' = CR)"() -> (w2522:u8)
        n772 = local read "Enable Termination\nChar (T)"() -> (w2523:bool)
        n773 = Index Array(array=w2530, index=0 ("Index")) -> (element=w2529:string)
        n774 = local read "parity"() -> (w2513:u16)
        n775 = local read "Delay before read (ms)"() -> (w2524:u32)
        n776 = local read "byte count"() -> (w2521:u32)
        n777 = local read "VISA resource name"() -> (w2517:refnum<visa-resource-name>)
        n778 = local read "baud rate"() -> (w2516:u32)
        n779 = local read "Serial End Mode for Reads"() -> (w2515:u16)
        n780 = local read "Timeout (ms)"() -> (w2520:u32)
        n781 = local read "data bits"() -> (w2514:u16)
        n782 = local read "stop bits"() -> (w2519:u16)
        n783 = local read "flow control"() -> (w2518:u16)
        n784 = call "Serial write and read v0.5.vi"("Delay before read (ms)"=w2524, "Termination char\n(0xA = '\\n' = LF)\n(0xD = '\\r' = CR)"=w2522, "Enable Termination\nChar (T)"=w2523, "parity"=w2513, "stop bits"=w2519, "string to write"=w2529, "flow control"=w2518, "byte count"=w2521, "Serial Settings:Serial End Mode for Reads"=w2515, "Timeout (ms)"=w2520, "error in (no error)"=w2535, "VISA resource name"=w2517, "baud rate"=w2516, "data bits"=w2514) -> ("Serial port output"=w2525:string, "error out"=w2534:errorcluster)
        n785 = Build Array (concatenate)(w2525, w2526) -> (w2527:string[])
      }
    }
    "Probe 4 Indicator" <- w70
    "Timings Indicator" <- w71
    n786 = local read "Time Units"() -> (w104:u16)
    n787 = case shown="0" w104 {
      tunnel: ["Time (Seconds)" ("element") "Time (Minutes)" ("element") "Time (Hours)" ("element")] -> w73
      frame 0 {
      }
      frame 1, Default {
      }
      frame 2 {
      }
    }
    n788 = Build Array(w153, w110, w120, w119, w118, w117, w116, w115, w114, w113, w112, w111, w109) -> (w174:dbl[][])
    n789 = Transpose 2D Array(2D array=w174) -> (transposed array=w173:dbl[][])
    n790 = Concatenate Strings(w79, "-I-vs-time.txt" ("Suffix (Imax,Imin,Ion,Ioff)")) -> (w184:string)
    n791 = Build Array(w73, "Is max (A)" ("VAR2 Name"), "Is min (A)" ("VAR2 Name"), "Id max (A)" ("VAR2 Name"), "Id min (A)" ("VAR2 Name"), "Ig max (A)" ("VAR2 Name"), "Ig min (A)" ("VAR2 Name"), "Is on (A)" ("VAR2 Name"), "Is off (A)" ("VAR2 Name"), "Id on (A)" ("VAR2 Name"), "Id off (A)" ("VAR2 Name"), "Ig on (A)" ("VAR2 Name"), "Ig off (A)" ("VAR2 Name")) -> (w179:string[])
    n792 = Array To Spreadsheet String(array=w173, 3:"%e" ("format string")) -> (spreadsheet string=w177:string)  [unwired: 1 in]
    n793 = Array To Spreadsheet String(array=w179, 3:"" ("format string")) -> (spreadsheet string=w178:string)  [unwired: 1 in]
    n794 = String To Path(string=w184) -> (path=w183:path)
    n795 = Build Array(w178, w177) -> (w176:string[])
    n796 = Write to Text File(file (use dialog)=w183, text=w176, error in=w152) -> (refnum out=w185:refnum<file>, error out=w175:errorcluster)  [unwired: 1 in, 1 out]
    n797 = Close File(refnum=w185, error in=w175) -> (error out=w107:errorcluster)  [unwired: 1 out]
    n798 = Concatenate Strings(w79, "-serial-port.txt" ("Suffix (serial port log)")) -> (w155:string)
    n799 = String To Path(string=w155) -> (path=w154:path)
    n800 = Build Array(w73, "Serial port input" ("VAR2 Name"), "Serial port output: ") -> (w145:string[])
    n801 = Array To Spreadsheet String(array=w149, 3:"" ("format string")) -> (spreadsheet string=w142:string)  [unwired: 1 in]
    n802 = Array To Spreadsheet String(array=w145, 3:"" ("format string")) -> (spreadsheet string=w143:string)  [unwired: 1 in]
    n803 = Build Array(w143, w142) -> (w144:string[])
    n804 = Array To Spreadsheet String(array=w148, 3:"" ("format string")) -> (spreadsheet string=w160:string)  [unwired: 1 in]
    n805 = Write to Text File(file (use dialog)=w154, text=w144, error in=w107) -> (refnum out=w156:refnum<file>, error out=w157:errorcluster)  [unwired: 1 in, 1 out]
    n806 = Close File(refnum=w156, error in=w157) -> (error out=w80:errorcluster)  [unwired: 1 out]
    n807 = local write "Serial port data"(w160) -> ()
    n808 = Build Array(w78, w77, w76, w75) -> (w89:dbl[][])
    n809 = Build Array(w73, "Is (A)" ("VAR2 Name"), "Id (A)" ("VAR2 Name"), "Ig (A)" ("VAR2 Name")) -> (w85:string[])
    n810 = Transpose 2D Array(2D array=w89) -> (transposed array=w88:dbl[][])
    n811 = Concatenate Strings(w79, "-sample.txt" ("Suffix (Imax,Imin,Ion,Ioff)")) -> (w95:string)
    n812 = Array To Spreadsheet String(array=w85, 3:"" ("format string")) -> (spreadsheet string=w84:string)  [unwired: 1 in]
    n813 = Array To Spreadsheet String(array=w88, 3:"%e" ("format string")) -> (spreadsheet string=w92:string)  [unwired: 1 in]
    n814 = String To Path(string=w95) -> (path=w94:path)
    n815 = Build Array(w84, w92) -> (w91:string[])
    n816 = Write to Text File(file (use dialog)=w94, text=w91, error in=w80) -> (refnum out=w96:refnum<file>, error out=w90:errorcluster)  [unwired: 1 in, 1 out]
    n817 = Close File(refnum=w96, error in=w90) -> (error out=w72:errorcluster)  [unwired: 1 out]
    "error out" <- w72
  }
  "Is max" <- w13
  "Id max" <- w13
  "Ig max" <- w13
  "Imax vs time" <- w2
  "I vs Vg" <- w2
  "Imin vs time" <- w2
  "I vs Vd" <- w2
  "Serial port data" <- "" ("Serial port data")
  "Is min" <- w12
  "Id min" <- w12
  "Ig min" <- w12
  "Ion vs time" <- w2
  "Ioff vs time" <- w2
  "Is on" <- w11
  "Id on" <- w11
  "Ig on" <- w11
  "Is off" <- w10
  "Id off" <- w10
  "Ig off" <- w10
  "I vs time (Bias Stress)" <- w2
  "Vp1" <- w3
  "Vp2" <- w3
  "Vp vs time (FPP Bias Stress)" <- w2
  "Vp vs Vg (FPP)" <- w2
  "Vdg vs time (Bias Stress)" <- w2
